vi "OP_Print_TPS_cluster_20171103.vi"() -> ()   [LabVIEW 2013]
uses:
  <vilib>/addons/database/Connection.llb/DB Tools Open Connec (Path).vi
  <vilib>/addons/database/Connection.llb/Conn Execute.vi
  <vilib>/addons/database/Recordset.llb/Rec Fetch Recordset Data (R).vi
  <vilib>/addons/database/Recordset.llb/Rec Destroy - Connection.vi
  <userlib>/caLab/Private/Get_PV-1D.vi
  <userlib>/caLab/Private/Get_PV.vi
  <vilib>/addons/database/_DB Variant To Data/Database Variant To Data.xnode
  <vilib>/addons/database/NI_Database_API.lvlib
panel:
  in  "Switch Tab":bool=TRUE
  out "Tab Control":enum32{"_____", "           "}(tab)
  out "Cluster":T1={"SR Fill Pattern"=array[864 elements], "Beam Current(mA"=320.769453, "Beam Lifetime(min)"=354.3939151043138, "Beamsize X(um)"=63.15189373514937, "Beamsize Y(um)"=38.03691397287648, "Tune X(from BPM)"=0.1487279843444227, "Tune Y(from BPM)"=0.2309197651663405, "Mode"="Top-Up", "NuX(from BBF) "=0.15142063757609414, "NuY(from BBF)"=0.22496346361412184, "IU22-23gap(R)"=7.0, "IU22-05gap(R)"=7.372, "IU22-05M"=TRUE, "IU22A-09gap(R)"=8.05, "IU22A-09M"=TRUE, "IU22B-09gap(R)"=40.001, "IU22B-09M"=FALSE, "IUT22-21gap(R)"=7.0, "IUT22-21M"=TRUE, "IU22-23M"=TRUE, "IU22A-25gap(R)"=7.0, "IU22A-25M"=TRUE, "IU22B-25gap(R)"=40.0, "IU22B-25M"=FALSE, "EPU48A-41gap(R)"=65.00055, "EPU48A-41gM"=FALSE, "EPU48B-41gap(R)"=27.450000000000003, "EPU48B-41gM"=TRUE, "EPU46-45gap(R)"=44.99850000000001, "EPU46-45gM"=FALSE, "EPU48A-41phase(R)"=0.00055, "EPU48B-41phase(R)"=0.0, "EPU46-45phase(R)"=5e-05, "Grid volt.(V)(S)"=33.0, "Gun mode"="MBM", "Mod.3 HV(kV)(S)"=35.37999999999996, "SR"="SR_DMB_2017_1024_0300LOCO.data", "BR"="Booster_2017_1023_0900.data", "Linac"="Linac_2017_0413_1015.data", "LTB"="LTB_JT_2017_0828_1050.data", "BTS"="BTS_2017_1023_0900.data", "RF2 remote"=TRUE, "RF2 OP mode"=TRUE, "RF2 phase.(S)"=-42.0, "RF Freq.(s)"=499655365.67399085, "RF2 gap volt.(S)"=1600.0, "RF3 remote"=TRUE, "RF3 OP mode"=TRUE, "RF3 phase.(S)"=1.1999999999999995, "RF3 gap volt.(S)"=1600.0, "BBF V"=TRUE, "BBF H"=TRUE, "BR ext. kicker1(kV)"=17.666, "BR ext. kicker2(kV)"=17.666, "BR ext. sep.1(V)"=322.14, "BR ext. sep.2(V)"=441.1, "BR inj. sep.(V)"=104.95, "BR inj. kicker(kV)"=13.449999999999969, "SR kicker4(kV)"=7.945, "SR kicker3(kV)"=8.02, "SR kicker2(kV)"=8.142, "SR kicker1(kV)"=8.1, "SR inj. sep.2(V)"=397.2, "SR inj. sep.1(V)"=398.04, "Bucket Start"=100.0, "Bucket Last"=450.0, "Bucket Step"=10.0, "Orbit ILK(P)"=TRUE, "IU22-05 Hutch Enable"=TRUE, "IU22A-09M Hutch Enable"=TRUE, "IUT22-21M Hutch Enable"=TRUE, "IU22-23M Hutch Enable"=TRUE, "IU22A-25M Hutch Enable"=TRUE, "EPU48A-41M Hutch Enable"=TRUE, "EPU46-45M Hutch Enable"=FALSE, "EPU46-45 FE Enable"=TRUE, "EPU48A-41 FE Enable"=TRUE, "IU22A-25 FE Enable"=TRUE, "IU22-23 FE Enable"=TRUE, "IUT22-21 FE Enable"=TRUE, "IU22A-09 FE Enable"=TRUE, "IU22-05 FE Enable"=TRUE, "EPU48A-41pM"=FALSE, "EPU48B-41pM"=TRUE, "EPU46-45pM"=FALSE, "Gun volt.(V)(S)"=23.5, "Width count"=75.0, "2ns step"=2.0, "10ps delay"=150.0, "phase shifter"=130.0015, "Taper"=1.0899999999999999, "05XBPMX 1"=14.279, "09XBPMX 1"=-34.837, "21XBPMX 1"=-36.466, "23XBPMX 1"=-38.547000000000004, "25XBPMX 1"=-40.08, "41XBPMX 1"=-513.551, "45XBPMX 1"=-12.86, "05XBPMY 1"=51.999, "09XBPMY 1"=30.004, "21XBPMY 1"=-4.771, "23XBPMY 1"=19.080000000000002, "25XBPMY 1"=-4.366, "41XBPMY 1"=309.241, "45XBPMY 1"=1.842, "FOFB H"="On", "FOFB V"="On", "time string"="15:45:09", "date"="2017/10/28", "date (last kicker ON)"="2017/10/28", "time string (last kicker ON)"="15:43:52", "Radio Buttons 2"=enum."absolute", "09XBPMX 2"="23.77", "09XBPMY 2"="-18.01", "05XBPMY 2"="-459.85", "05XBPMX 2"="-403.56", "21XBPMY 2"="-134.87", "21XBPMX 2"="-31.92", "23XBPMY 2"="233.82", "23XBPMX 2"="11.09", "25XBPMY 2"="5171.53", "25XBPMX 2"="2152.43", "41XBPMY 2"=" closed", "41XBPMX 2"=" PAB ", "45XBPMX 2"=" Hutch ", "45XBPMY 2"=" closed", "05 mode"="Follow", "09A mode"="Follow", "09B mode"="Follow", "21 mode"="Follow", "23 mode"="Follow", "25A mode"="Follow", "25B mode"="Follow", "41A mode"="Follow", "41B mode"="Follow", "46 mode"="Follow", "BeamCurrent History"={"BPM NO.  1_172"=array[4319 elements], array[4319 elements]}, "SR Beam Current in            hours"=12.0, "RF FB"="On", "BPMX Graph 2"={"Array of X axis  平均分配至各段"=[1.0, 1.1666666666666667, 1.3333333333333333, 1.5, 1.6666666666666665, 1.8333333333333333, 2.0, 2.142857142857143, 2.2857142857142856, 2.4285714285714284, 2.571428571428571, 2.7142857142857144, 2.857142857142857, 3.0, 3.142857142857143, 3.2857142857142856, 3.4285714285714284, 3.571428571428571, 3.7142857142857144, 3.857142857142857, 4.0, 4.125, 4.25, 4.375, 4.5, 4.625, 4.75, 4.875, 5.0, 5.125, 5.25, 5.375, 5.5, 5.625, 5.75, 5.875, 6.0, 6.142857142857143, 6.285714285714286, 6.428571428571429, 6.571428571428571, 6.714285714285714, 6.857142857142857, 7.0, 7.142857142857143, 7.285714285714286, 7.428571428571429, 7.571428571428571, 7.714285714285714, 7.857142857142857, 8.0, 8.142857142857142, 8.285714285714286, 8.428571428571429, 8.571428571428571, 8.714285714285714, 8.857142857142858, 9.0, 9.142857142857142, 9.285714285714286, 9.428571428571429, 9.571428571428571, 9.714285714285714, 9.857142857142858, 10.0, 10.142857142857142, 10.285714285714286, 10.428571428571429, 10.571428571428571, 10.714285714285714, 10.857142857142858, 11.0, 11.142857142857142, 11.285714285714286, 11.428571428571429, 11.571428571428571, 11.714285714285714, 11.857142857142858, 12.0, 12.125, 12.25, 12.375, 12.5, 12.625, 12.75, 12.875, 13.0, 13.125, 13.25, 13.375, 13.5, 13.625, 13.75, 13.875, 14.0, 14.142857142857142, 14.285714285714286, 14.428571428571429, 14.571428571428571, 14.714285714285714, 14.857142857142858, 15.0, 15.142857142857142, 15.285714285714286, 15.428571428571429, 15.571428571428571, 15.714285714285714, 15.857142857142858, 16.0, 16.142857142857142, 16.285714285714285, 16.428571428571427, 16.571428571428573, 16.714285714285715, 16.857142857142858, 17.0, 17.142857142857142, 17.285714285714285, 17.428571428571427, 17.571428571428573, 17.714285714285715, 17.857142857142858, 18.0, 18.142857142857142, 18.285714285714285, 18.428571428571427, 18.571428571428573, 18.714285714285715, 18.857142857142858, 19.0, 19.142857142857142, 19.285714285714285, 19.428571428571427, 19.571428571428573, 19.714285714285715, 19.857142857142858, 20.0, 20.125, 20.25, 20.375, 20.5, 20.625, 20.75, 20.875, 21.0, 21.125, 21.25, 21.375, 21.5, 21.625, 21.75, 21.875, 22.0, 22.142857142857142, 22.285714285714285, 22.428571428571427, 22.571428571428573, 22.714285714285715, 22.857142857142858, 23.0, 23.142857142857142, 23.285714285714285, 23.428571428571427, 23.571428571428573, 23.714285714285715, 23.857142857142858, 24.0, 24.166666666666668, 24.333333333333332, 24.5, 24.666666666666668, 24.833333333333332], [-104.35000000000001, -27.61, -81.269, 31.074, 6.062, -136.0, 99.494, -88.141, -46.889, -165.06900000000002, 6.021, -84.98, 1.75, -8.811, 8.532, -133.949, -96.848, 24.799, 5.059, -100.301, 144.643, -9.353, 21.271, -55.053000000000004, 53.308, 191.175, 158.868, 222.566, -123.501, -26.869, 534.8770000000001, 573.141, -225.076, -6.779, 120.711, -75.419, 85.256, 50.948, -59.4, -203.09900000000002, -20.847, 130.465, -112.508, 76.115, 15.039, -35.207, -105.659, -16.897000000000002, 68.91, -141.159, 107.378, 144.351, -55.053000000000004, -193.076, 129.21, 58.157000000000004, -162.566, 153.643, 28.149, 9.358, -84.211, 85.112, 22.422, -31.252, 89.379, -47.49, 54.793, -68.275, 110.611, -118.584, -371.90500000000003, -20.115000000000002, -329.103, -249.097, -146.817, 118.556, -25.749, -98.32600000000001, 55.269, -122.093, 50.967, -55.89, 88.019, -0.462, -608.1560000000001, -139.752, -304.999, -215.022, 93.23400000000001, 44.699, -65.235, 37.049, -3.491, -169.852, 216.458, 50.398, -92.285, -132.13400000000001, -12.869, 66.74, -188.53300000000002, 148.653, -5.112, -71.334, -177.681, 41.168, -12.532, -184.913, 194.919, 52.414, -75.628, -80.415, -36.814, 105.73100000000001, -104.36800000000001, 110.101, 49.669000000000004, -67.327, -157.372, 29.624000000000002, 22.156, -105.663, 47.799, 11.591000000000001, -75.285, -79.821, 34.331, -24.937, -158.703, 177.15, 200.872, -165.849, -60.67, 20.183, -15.311, -111.206, 107.58800000000001, 26.489, 69.547, -41.230000000000004, 81.986, 54.43, 253.076, 378.43600000000004, -117.003, -304.999, 131.013, 2.21, -158.435, 94.489, 63.017, -82.94500000000001, 99.147, 65.752, -37.261, -102.577, 41.791000000000004, 66.599, -163.73, 160.137, -7.15, -51.275, -140.353, 33.772, 54.203, -147.597, 128.696, 58.22, -47.144, -184.493, 56.980000000000004, 67.437, -54.227000000000004, -0.031]}, "BPMY Graph 2"={"Array of X axis  平均分配至各段"=[1.0, 1.1666666666666667, 1.3333333333333333, 1.5, 1.6666666666666665, 1.8333333333333333, 2.0, 2.142857142857143, 2.2857142857142856, 2.4285714285714284, 2.571428571428571, 2.7142857142857144, 2.857142857142857, 3.0, 3.142857142857143, 3.2857142857142856, 3.4285714285714284, 3.571428571428571, 3.7142857142857144, 3.857142857142857, 4.0, 4.125, 4.25, 4.375, 4.5, 4.625, 4.75, 4.875, 5.0, 5.125, 5.25, 5.375, 5.5, 5.625, 5.75, 5.875, 6.0, 6.142857142857143, 6.285714285714286, 6.428571428571429, 6.571428571428571, 6.714285714285714, 6.857142857142857, 7.0, 7.142857142857143, 7.285714285714286, 7.428571428571429, 7.571428571428571, 7.714285714285714, 7.857142857142857, 8.0, 8.142857142857142, 8.285714285714286, 8.428571428571429, 8.571428571428571, 8.714285714285714, 8.857142857142858, 9.0, 9.142857142857142, 9.285714285714286, 9.428571428571429, 9.571428571428571, 9.714285714285714, 9.857142857142858, 10.0, 10.142857142857142, 10.285714285714286, 10.428571428571429, 10.571428571428571, 10.714285714285714, 10.857142857142858, 11.0, 11.142857142857142, 11.285714285714286, 11.428571428571429, 11.571428571428571, 11.714285714285714, 11.857142857142858, 12.0, 12.125, 12.25, 12.375, 12.5, 12.625, 12.75, 12.875, 13.0, 13.125, 13.25, 13.375, 13.5, 13.625, 13.75, 13.875, 14.0, 14.142857142857142, 14.285714285714286, 14.428571428571429, 14.571428571428571, 14.714285714285714, 14.857142857142858, 15.0, 15.142857142857142, 15.285714285714286, 15.428571428571429, 15.571428571428571, 15.714285714285714, 15.857142857142858, 16.0, 16.142857142857142, 16.285714285714285, 16.428571428571427, 16.571428571428573, 16.714285714285715, 16.857142857142858, 17.0, 17.142857142857142, 17.285714285714285, 17.428571428571427, 17.571428571428573, 17.714285714285715, 17.857142857142858, 18.0, 18.142857142857142, 18.285714285714285, 18.428571428571427, 18.571428571428573, 18.714285714285715, 18.857142857142858, 19.0, 19.142857142857142, 19.285714285714285, 19.428571428571427, 19.571428571428573, 19.714285714285715, 19.857142857142858, 20.0, 20.125, 20.25, 20.375, 20.5, 20.625, 20.75, 20.875, 21.0, 21.125, 21.25, 21.375, 21.5, 21.625, 21.75, 21.875, 22.0, 22.142857142857142, 22.285714285714285, 22.428571428571427, 22.571428571428573, 22.714285714285715, 22.857142857142858, 23.0, 23.142857142857142, 23.285714285714285, 23.428571428571427, 23.571428571428573, 23.714285714285715, 23.857142857142858, 24.0, 24.166666666666668, 24.333333333333332, 24.5, 24.666666666666668, 24.833333333333332], [-143.858, -13.775, -13.785, 122.665, -66.475, 31.541, 2.118, -24.67, 28.275000000000002, 0.139, -36.578, -28.396, 48.925000000000004, 9.287, -3.412, 70.053, -21.479, 14.89, -7.234, 5.521, -3.164, 19.558, -37.538000000000004, 37.11, -77.159, -13.755, 77.63, 28.249000000000002, -209.114, -44.569, 92.851, 173.641, -70.156, -22.722, 17.795, -6.59, 25.654, -41.882, 53.713, 9.237, -26.164, 18.357, 63.695, -8.542, 5.183, -5.99, 9.508000000000001, -5.462, -29.446, 36.574, -52.552, 51.439, -48.502, 0.73, -23.836000000000002, -3.648, -9.628, -5.485, -68.679, 95.486, -62.041000000000004, 54.633, -58.791000000000004, 68.305, -49.682, 29.838, -8.459, 3.213, -5.561, -80.617, 58.144, 15.346, -158.743, -40.726, 5.259, 3.258, 41.128, -54.377, 5.01, 18.84, 11.403, -20.73, 21.792, -17.296, 27.29, 0.783, -6.804, -137.476, 116.70700000000001, -6.929, 17.846, -3.586, 11.754, 6.341, 0.292, -0.911, -8.236, -5.312, 14.939, -29.945, 30.573, -9.991, -49.344, 82.117, -27.45, 22.291, -6.636, -9.389, 10.034, -14.218, 14.215, -7.3, 12.409, -44.302, 50.197, -36.089, -9.120000000000001, 45.881, 14.836, -27.324, 10.765, -10.139, -33.252, 2.737, -9.99, -6.019, -53.329, -28.159, 2.676, -36.9, -2.372, 8.92, 13.599, -25.723, -16.436, 7.722, -0.088, -29.122, 32.814, -20.521, 30.155, -45.734, 36.611000000000004, 74.528, 68.482, -22.548000000000002, -31.398, 134.603, -45.587, -0.981, -40.156, 24.441, 20.477, -31.424, 19.5, -11.789, 16.394000000000002, -38.567, 9.523, 0.09, -0.058, -4.8500000000000005, 11.71, 25.637, -10.51, -18.101, -12.389000000000001, 95.417, -138.726, 30.355, 96.245, -48.666000000000004, 40.851, -0.71]}, "gap value："=0} {"SR Beam Current in            hours" min=1.0 max=24.0 step=1.0 format="%#_2f"; "45XBPMY 1" format="%#.2f"; "41XBPMY 1" format="%#.2f"; "25XBPMY 1" format="%#.2f"; "23XBPMY 1" format="%#.2f"; "21XBPMY 1" format="%#.2f"; "09XBPMY 1" format="%#.2f"; "05XBPMY 1" format="%#.2f"; "45XBPMX 1" format="%#.2f"; "41XBPMX 1" format="%#.2f"; "25XBPMX 1" format="%#.2f"; "23XBPMX 1" format="%#.2f"; "21XBPMX 1" format="%#.2f"; "09XBPMX 1" format="%#.2f"; "05XBPMX 1" format="%#.2f"; "Taper" format="%#.4f"; "phase shifter" format="%#.3f"; "10ps delay" format="%#.1f"; "2ns step" format="%#.1f"; "Width count" format="%#.1f"; "Gun volt.(V)(S)" format="%#.1f"; "Bucket Step" format="%#.2f"; "Bucket Last" format="%#.2f"; "Bucket Start" format="%#.2f"; "BR ext. kicker1(kV)" format="%#.2f"; "BR ext. kicker2(kV)" format="%#.2f"; "BR ext. sep.1(V)" format="%#.2f"; "BR ext. sep.2(V)" format="%#.2f"; "BR inj. sep.(V)" format="%#.3f"; "BR inj. kicker(kV)" format="%#.3f"; "SR kicker4(kV)" format="%#.2f"; "SR kicker3(kV)" format="%#.2f"; "SR kicker2(kV)" format="%#.2f"; "SR kicker1(kV)" format="%#.2f"; "SR inj. sep.2(V)" format="%#.2f"; "SR inj. sep.1(V)" format="%#.2f"; "RF3 gap volt.(S)" format="%#.0f"; "RF3 phase.(S)" format="%#.1f"; "RF2 gap volt.(S)" format="%#.0f"; "RF Freq.(s)" format="%#.1f"; "RF2 phase.(S)" format="%#.1f"; "Mod.3 HV(kV)(S)" format="%#.3f"; "Grid volt.(V)(S)" format="%#.1f"; "EPU46-45phase(R)" format="%#.4f"; "EPU48B-41phase(R)" format="%#.4f"; "EPU48A-41phase(R)" format="%#.4f"; "EPU46-45gap(R)" format="%#.4f"; "EPU48B-41gap(R)" format="%#.4f"; "EPU48A-41gap(R)" format="%#.4f"; "IU22B-25gap(R)" format="%#.4f"; "IU22A-25gap(R)" format="%#.4f"; "IUT22-21gap(R)" format="%#.4f"; "IU22B-09gap(R)" format="%#.4f"; "IU22A-09gap(R)" format="%#.4f"; "IU22-05gap(R)" format="%#.4f"; "IU22-23gap(R)" format="%#.4f"; "NuY(from BBF)" format="%#.4f"; "NuX(from BBF)" format="%#.4f"; "Tune Y(from BPM)" format="%#.4f"; "Tune X(from BPM)" format="%#.4f"; "Beamsize Y(um)" format="%#.2f"; "Beamsize X(um)" format="%#.2f"; "Beam Lifetime(min)" format="%#.3f"; "Beam Current(mA" format="%#.3f"}
  out "Diff list":string[][](array[string])
  out "EVENTs":i32
  out "check loop":i32
  in  "Check period":i32=10 min=0 max=10
  out "Program Start Time":dbl=3592021508.642459
  out "dT":u32=325
  out "x > y?":bool
  out "PV list":string[](array[string])=["LI-ES-CPS-01:SETMODE", "LI-ES-CPS-01:PULSEMODE", "LI-ES-BPS-01:SETU:GRID", "LI-ES-BPS-01:SETU:SBM", "LI-ES-BPS-01:SETU:MBM", "LI-RF-CAB-07:SET:MODE", "LI-RF-HVP-11:SET:U", "LI-RF-CAB-09:SET:MODE", "LI-RF-HVP-21:SET:U", "LI-RF-CAB-11:SET:MODE", "LI-RF-HVP-31:SET:U", "LI-RF-WGA-01:SET:POS", "LI-RF-WGA-02:SET:POS", "LI-RF-WGA-03:SET:POS", "LI-RF-SFT-01:SET:POS", "LI-RF-SFT-02:SET:POS", "LI-RF-SFT-03:SET:POS", "LI-RF-CTR-01:ES:SET:DEG", "LI-RF-CTR-01:SP:SET:DEG", "LI-RF-CTR-01:K123:SET:DEG", "LI-RF-CTR-01:K1:SET:DEG", "LI-RF-CTR-01:K3:SET:DEG", "LI-RF-AMP-01:SET:PWR", "LI-RF-AMP-02:SET:PWR", "LI-MA-SPS-01:SET:I", "LI-MA-SPS-02:SET:I", "LI-MA-SPS-03:SET:I", "LI-MA-SPS-04:SET:I", "LI-MA-SPS-05:SET:I", "LI-MA-SPS-06:SET:I", "LI-MA-SPS-07:SET:I", "LI-MA-SPS-08:SET:I", "LI-MA-SPS-09:SET:I", "LI-MA-SPS-10:SET:I", "LI-MA-SPS-11:SET:I", "LI-MA-SPS-12:SET:I", "LI-MA-SPS-13:SET:I", "LI-MA-SPS-14:SET:I", "LI-MA-SPS-15:SET:I", "LI-MA-SPS-16:SET:I", "LI-MA-STP-01:SET:I", "LI-MA-STP-02:SET:I", "LI-MA-STP-03:SET:I", "LI-MA-STP-04:SET:I", "LI-MA-STP-05:SET:I", "LI-MA-STP-06:SET:I", "LI-MA-STP-07:SET:I", "LI-MA-STP-08:SET:I", "LI-MA-STP-09:SET:I", "LI-MA-STP-10:SET:I", "LI-MA-STP-11:SET:I", "LI-MA-STP-12:SET:I", "LI-MA-STP-13:SET:I", "LI-MA-STP-14:SET:I", "LI-MA-STP-15:SET:I", "LI-MA-STP-16:SET:I", "LI-MA-QPS-01:SET:I", "LI-MA-QPS-02:SET:I", "LI-MA-QPS-03:SET:I", "LI-MA-QPS-04:SET:I", "LI-MA-QPS-05:SET:I", "LI-MA-QPS-06:SET:I", "CPCITM-TI-EVRTG:Pulse7DelaySet", "CPCITM-TI-EVRTG:Pulse7WidthSet", "CPCITM-TI-EVRTG:GTX7CtrlGTXPHSet", "CPCITM-TI-EVRTG:GTX7DlySet", "CPCITM-TI-EVRTG:Pulse6DelaySet", "CPCITM-TI-EVRTG:Pulse6WidthSet", "CPCITM-TI-EVRTG:GTX6CtrlGTXPHSet", "CPCITM-TI-EVRTG:GTX6DlySet", "CPCILI-TI-EVR:Pulse2DelaySet", "CPCILI-TI-EVR:Pulse2WidthSet", "CPCILI-TI-EVR:Pulse3DelaySet", "CPCILI-TI-EVR:Pulse3WidthSet", "CPCILI-TI-EVR:Pulse4DelaySet", "CPCILI-TI-EVR:Pulse4WidthSet", "CPCILI-TI-EVR:Pulse5DelaySet", "CPCILI-TI-EVR:Pulse5WidthSet", "CPCILI-TI-EVR:Pulse6DelaySet", "CPCILI-TI-EVR:Pulse6WidthSet", "CPCILI-TI-EVR:Pulse7DelaySet", "CPCILI-TI-EVR:Pulse7WidthSet", "CPCILI-TI-EVR:Pulse8DelaySet", "CPCILI-TI-EVR:Pulse8WidthSet", "CPCILI-TI-EVR:Pulse9DelaySet", "CPCILI-TI-EVR:Pulse9WidthSet", "CPCITM-TI-EVRTG:GTX6DlySet", "CPCITM-TI-EVRTG:GTX7DlySet", "LTB-PS-HC-1:setI", "LTB-PS-HC-2:setI", "LTB-PS-HC-3:setI", "LTB-PS-HC-4:setI", "LTB-PS-HC-5:setI", "LTB-PS-VC-1:setI", "LTB-PS-VC-2:setI", "LTB-PS-VC-3:setI", "LTB-PS-VC-4:setI", "LTB-PS-VC-5:setI", "LTB-PS-VC-6:setI", "LTB-PS-VC-7:setI", "LTB-PS-Q1A:setI", "LTB-PS-Q1B:setI", "LTB-PS-Q1C:setI", "LTB-PS-Q2A:setI", "LTB-PS-Q2B:setI", "LTB-PS-Q2C:setI", "LTB-PS-Q3A:setI", "LTB-PS-Q3B:setI", "LTB-PS-Q4A:setI", "LTB-PS-Q4B:setI", "LTB-PS-QQ:setI", "LTB-PS-BEND-1:setI", "LTB-PS-VC-2a:setI", "LTB-PS-HC-3a:setI", "LTB-PS-HC-3b:setI", "LTB-PS-HC-4a:setI", "LTB-PS-HC-5a:setI", "LI-DI-SLIT-motor:axis2Position1", "LI-DI-SLIT-motor:axis1Position1", "BR-PS-HC-101:setI", "BR-PS-HC-102:setI", "BR-PS-HC-103:setI", "BR-PS-HC-104:setI", "BR-PS-HC-105:setI", "BR-PS-HC-106:setI", "BR-PS-HC-107:setI", "BR-PS-HC-108:setI", "BR-PS-HC-109:setI", "BR-PS-HC-110:setI", "BR-PS-HC-201:setI", "BR-PS-HC-202:setI", "BR-PS-HC-203:setI", "BR-PS-HC-204:setI", "BR-PS-HC-205:setI", "BR-PS-HC-206:setI", "BR-PS-HC-207:setI", "BR-PS-HC-208:setI", "BR-PS-HC-209:setI", "BR-PS-HC-210:setI", "BR-PS-HC-301:setI", "BR-PS-HC-302:setI", "BR-PS-HC-303:setI", "BR-PS-HC-304:setI", "BR-PS-HC-305:setI", "BR-PS-HC-306:setI", "BR-PS-HC-307:setI", "BR-PS-HC-308:setI", "BR-PS-HC-309:setI", "BR-PS-HC-310:setI", "BR-PS-HC-401:setI", "BR-PS-HC-402:setI", "BR-PS-HC-403:setI", "BR-PS-HC-404:setI", "BR-PS-HC-405:setI", "BR-PS-HC-406:setI", "BR-PS-HC-407:setI", "BR-PS-HC-408:setI", "BR-PS-HC-409:setI", "BR-PS-HC-410:setI", "BR-PS-HC-501:setI", "BR-PS-HC-502:setI", "BR-PS-HC-503:setI", "BR-PS-HC-504:setI", "BR-PS-HC-505:setI", "BR-PS-HC-506:setI", "BR-PS-HC-507:setI", "BR-PS-HC-508:setI", "BR-PS-HC-509:setI", "BR-PS-HC-510:setI", "BR-PS-HC-601:setI", "BR-PS-HC-602:setI", "BR-PS-HC-603:setI", "BR-PS-HC-603a:setI", "BR-PS-HC-604:setI", "BR-PS-HC-605:setI", "BR-PS-HC-606:setI", "BR-PS-HC-606a:setI", "BR-PS-HC-607:setI", "BR-PS-HC-608:setI", "BR-PS-HC-609:setI", "BR-PS-HC-610:setI", "BR-PS-VC-101:setI", "BR-PS-VC-102:setI", "BR-PS-VC-103:setI", "BR-PS-VC-104:setI", "BR-PS-VC-105:setI", "BR-PS-VC-106:setI", "BR-PS-VC-201:setI", "BR-PS-VC-202:setI", "BR-PS-VC-203:setI", "BR-PS-VC-204:setI", "BR-PS-VC-205:setI", "BR-PS-VC-206:setI", "BR-PS-VC-301:setI", "BR-PS-VC-302:setI", "BR-PS-VC-303:setI", "BR-PS-VC-304:setI", "BR-PS-VC-305:setI", "BR-PS-VC-306:setI", "BR-PS-VC-401:setI", "BR-PS-VC-402:setI", "BR-PS-VC-403:setI", "BR-PS-VC-404:setI", "BR-PS-VC-405:setI", "BR-PS-VC-406:setI", "BR-PS-VC-501:setI", "BR-PS-VC-502:setI", "BR-PS-VC-503:setI", "BR-PS-VC-504:setI", "BR-PS-VC-505:setI", "BR-PS-VC-506:setI", "BR-PS-VC-601:setI", "BR-PS-VC-602:setI", "BR-PS-VC-602a:setI", "BR-PS-VC-603:setI", "BR-PS-VC-604:setI", "BR-PS-VC-604a:setI", "BR-PS-VC-605:setI", "BR-PS-VC-606:setI", "BR-PS-VC-100a:setI", "BR-PS-SD:setI", "BR-PS-SF:setI", "cpsc_027:AO:SLOW_SET:CH:1", "cpsc_037:AO:SLOW_SET:CH:3", "BR-RF-LLRF:setStationPhase", "TI-INJ-PROC:setTinj", "BR-PS-INJ-SE:setHV", "CPCIPM-TI-EVR:Pulse1DelaySet", "BR-PS-INJ-KI:setHV", "CPCIPM-TI-EVR:Pulse2DelaySet", "BR-PS-QF:setWfDC", "BR-PS-QM:setWfDC", "BR-PS-Q1:setWfDC", "BR-PS-Q2:setWfDC", "BR-PS-BEND:setWfDC", "BTS-PS-HC-1:setI", "BTS-PS-HC-2:setI", "BTS-PS-HC-3:setI", "BTS-PS-HC-4:setI", "BTS-PS-HC-5:setI", "BTS-PS-VC-2:setI", "BTS-PS-VC-3:setI", "BTS-PS-VC-4:setI", "BTS-PS-VC-5:setI", "BTS-PS-VC-6:setI", "BTS-PS-Q1A:setI", "BTS-PS-Q1B:setI", "BTS-PS-Q1C:setI", "BTS-PS-Q2A:setI", "BTS-PS-Q2B:setI", "BTS-PS-Q2C:setI", "BTS-PS-Q3A:setI", "BTS-PS-BEND-1:setI", "BTS-PS-BEND-2:setI", "BR-PS-EXT-K1:setHV", "BR-PS-EXT-K2:setHV", "SR-PS-INJ-SE1:setHV", "SR-PS-INJ-SE2:setHV", "SR-PS-INJ-K1:setHV", "SR-PS-INJ-K2:setHV", "SR-PS-INJ-K3:setHV", "SR-PS-INJ-K4:setHV", "CPCIPM-TI-EVR:Pulse4DelaySet", "CPCIPM-TI-EVR:Pulse5DelaySet", "CPCIPM-TI-EVR:Pulse3DelaySet", "CPCIPM-TI-EVR:Pulse6DelaySet", "CPCIPM-TI-EVR:Pulse7DelaySet", "T560:setADelay", "T560:setBDelay", "T560:setCDelay", "T560:setDDelay", "CPCIPM-TI-EVR:Pulse4DelaySet", "CPCIPM-TI-EVR:Pulse5DelaySet", "BR-PS-EXT-SE1:setHV", "BR-PS-EXT-SE2:setHV", "CPCIPM-TI-EVR:Pulse3DelaySet", "CPCIPM-TI-EVR:Pulse11DelaySet", "SR-PS-BEND:setI", "SR-PS-HC-011:setI", "SR-PS-HC-012:setI", "SR-PS-HC-013:setI", "SR-PS-HC-014:setI", "SR-PS-HC-015:setI", "SR-PS-HC-016:setI", "SR-PS-HC-017:setI", "SR-PS-HC-021:setI", "SR-PS-HC-022:setI", "SR-PS-HC-023:setI", "SR-PS-HC-024:setI", "SR-PS-HC-025:setI", "SR-PS-HC-026:setI", "SR-PS-HC-027:setI", "SR-PS-HC-031:setI", "SR-PS-HC-032:setI", "SR-PS-HC-033:setI", "SR-PS-HC-034:setI", "SR-PS-HC-035:setI", "SR-PS-HC-036:setI", "SR-PS-HC-037:setI", "SR-PS-HC-041:setI", "SR-PS-HC-042:setI", "SR-PS-HC-043:setI", "SR-PS-HC-044:setI", "SR-PS-HC-045:setI", "SR-PS-HC-046:setI", "SR-PS-HC-047:setI", "SR-PS-HC-051:setI", "SR-PS-HC-052:setI", "SR-PS-HC-053:setI", "SR-PS-HC-054:setI", "SR-PS-HC-055:setI", "SR-PS-HC-056:setI", "SR-PS-HC-057:setI", "SR-PS-HC-061:setI", "SR-PS-HC-062:setI", "SR-PS-HC-063:setI", "SR-PS-HC-064:setI", "SR-PS-HC-065:setI", "SR-PS-HC-066:setI", "SR-PS-HC-067:setI", "SR-PS-HC-071:setI", "SR-PS-HC-072:setI", "SR-PS-HC-073:setI", "SR-PS-HC-074:setI", "SR-PS-HC-075:setI", "SR-PS-HC-076:setI", "SR-PS-HC-077:setI", "SR-PS-HC-081:setI", "SR-PS-HC-082:setI", "SR-PS-HC-083:setI", "SR-PS-HC-084:setI", "SR-PS-HC-085:setI", "SR-PS-HC-086:setI", "SR-PS-HC-087:setI", "SR-PS-HC-091:setI", "SR-PS-HC-092:setI", "SR-PS-HC-093:setI", "SR-PS-HC-094:setI", "SR-PS-HC-095:setI", "SR-PS-HC-096:setI", "SR-PS-HC-097:setI", "SR-PS-HC-101:setI", "SR-PS-HC-102:setI", "SR-PS-HC-103:setI", "SR-PS-HC-104:setI", "SR-PS-HC-105:setI", "SR-PS-HC-106:setI", "SR-PS-HC-107:setI", "SR-PS-HC-111:setI", "SR-PS-HC-112:setI", "SR-PS-HC-113:setI", "SR-PS-HC-114:setI", "SR-PS-HC-115:setI", "SR-PS-HC-116:setI", "SR-PS-HC-117:setI", "SR-PS-HC-121:setI", "SR-PS-HC-122:setI", "SR-PS-HC-123:setI", "SR-PS-HC-124:setI", "SR-PS-HC-125:setI", "SR-PS-HC-126:setI", "SR-PS-HC-127:setI", "SR-PS-HC-131:setI", "SR-PS-HC-132:setI", "SR-PS-HC-133:setI", "SR-PS-HC-134:setI", "SR-PS-HC-135:setI", "SR-PS-HC-136:setI", "SR-PS-HC-137:setI", "SR-PS-HC-141:setI", "SR-PS-HC-142:setI", "SR-PS-HC-143:setI", "SR-PS-HC-144:setI", "SR-PS-HC-145:setI", "SR-PS-HC-146:setI", "SR-PS-HC-147:setI", "SR-PS-HC-151:setI", "SR-PS-HC-152:setI", "SR-PS-HC-153:setI", "SR-PS-HC-154:setI", "SR-PS-HC-155:setI", "SR-PS-HC-156:setI", "SR-PS-HC-157:setI", "SR-PS-HC-161:setI", "SR-PS-HC-162:setI", "SR-PS-HC-163:setI", "SR-PS-HC-164:setI", "SR-PS-HC-165:setI", "SR-PS-HC-166:setI", "SR-PS-HC-167:setI", "SR-PS-HC-171:setI", "SR-PS-HC-172:setI", "SR-PS-HC-173:setI", "SR-PS-HC-174:setI", "SR-PS-HC-175:setI", "SR-PS-HC-176:setI", "SR-PS-HC-177:setI", "SR-PS-HC-181:setI", "SR-PS-HC-182:setI", "SR-PS-HC-183:setI", "SR-PS-HC-184:setI", "SR-PS-HC-185:setI", "SR-PS-HC-186:setI", "SR-PS-HC-187:setI", "SR-PS-HC-191:setI", "SR-PS-HC-192:setI", "SR-PS-HC-193:setI", "SR-PS-HC-194:setI", "SR-PS-HC-195:setI", "SR-PS-HC-196:setI", "SR-PS-HC-197:setI", "SR-PS-HC-201:setI", "SR-PS-HC-202:setI", "SR-PS-HC-203:setI", "SR-PS-HC-204:setI", "SR-PS-HC-205:setI", "SR-PS-HC-206:setI", "SR-PS-HC-207:setI", "SR-PS-HC-211:setI", "SR-PS-HC-212:setI", "SR-PS-HC-213:setI", "SR-PS-HC-214:setI", "SR-PS-HC-215:setI", "SR-PS-HC-216:setI", "SR-PS-HC-217:setI", "SR-PS-HC-221:setI", "SR-PS-HC-222:setI", "SR-PS-HC-223:setI", "SR-PS-HC-224:setI", "SR-PS-HC-225:setI", "SR-PS-HC-226:setI", "SR-PS-HC-227:setI", "SR-PS-HC-231:setI", "SR-PS-HC-232:setI", "SR-PS-HC-233:setI", "SR-PS-HC-234:setI", "SR-PS-HC-235:setI", "SR-PS-HC-236:setI", "SR-PS-HC-237:setI", "SR-PS-HC-241:setI", "SR-PS-HC-242:setI", "SR-PS-HC-243:setI", "SR-PS-HC-244:setI", "SR-PS-HC-245:setI", "SR-PS-HC-246:setI", "SR-PS-HC-247:setI", "SR-PS-VC-011:setI", "SR-PS-VC-012:setI", "SR-PS-VC-013:setI", "SR-PS-VC-014:setI", "SR-PS-VC-015:setI", "SR-PS-VC-016:setI", "SR-PS-VC-017:setI", "SR-PS-VC-021:setI", "SR-PS-VC-022:setI", "SR-PS-VC-023:setI", "SR-PS-VC-024:setI", "SR-PS-VC-025:setI", "SR-PS-VC-026:setI", "SR-PS-VC-027:setI", "SR-PS-VC-031:setI", "SR-PS-VC-032:setI", "SR-PS-VC-033:setI", "SR-PS-VC-034:setI", "SR-PS-VC-035:setI", "SR-PS-VC-036:setI", "SR-PS-VC-037:setI", "SR-PS-VC-041:setI", "SR-PS-VC-042:setI", "SR-PS-VC-043:setI", "SR-PS-VC-044:setI", "SR-PS-VC-045:setI", "SR-PS-VC-046:setI", "SR-PS-VC-047:setI", "SR-PS-VC-051:setI", "SR-PS-VC-052:setI", "SR-PS-VC-053:setI", "SR-PS-VC-054:setI", "SR-PS-VC-055:setI", "SR-PS-VC-056:setI", "SR-PS-VC-057:setI", "SR-PS-VC-061:setI", "SR-PS-VC-062:setI", "SR-PS-VC-063:setI", "SR-PS-VC-064:setI", "SR-PS-VC-065:setI", "SR-PS-VC-066:setI", "SR-PS-VC-067:setI", "SR-PS-VC-071:setI", "SR-PS-VC-072:setI", "SR-PS-VC-073:setI", "SR-PS-VC-074:setI", "SR-PS-VC-075:setI", "SR-PS-VC-076:setI", "SR-PS-VC-077:setI", "SR-PS-VC-081:setI", "SR-PS-VC-082:setI", "SR-PS-VC-083:setI", "SR-PS-VC-084:setI", "SR-PS-VC-085:setI", "SR-PS-VC-086:setI", "SR-PS-VC-087:setI", "SR-PS-VC-091:setI", "SR-PS-VC-092:setI", "SR-PS-VC-093:setI", "SR-PS-VC-094:setI", "SR-PS-VC-095:setI", "SR-PS-VC-096:setI", "SR-PS-VC-097:setI", "SR-PS-VC-101:setI", "SR-PS-VC-102:setI", "SR-PS-VC-103:setI", "SR-PS-VC-104:setI", "SR-PS-VC-105:setI", "SR-PS-VC-106:setI", "SR-PS-VC-107:setI", "SR-PS-VC-111:setI", "SR-PS-VC-112:setI", "SR-PS-VC-113:setI", "SR-PS-VC-114:setI", "SR-PS-VC-115:setI", "SR-PS-VC-116:setI", "SR-PS-VC-117:setI", "SR-PS-VC-121:setI", "SR-PS-VC-122:setI", "SR-PS-VC-123:setI", "SR-PS-VC-124:setI", "SR-PS-VC-125:setI", "SR-PS-VC-126:setI", "SR-PS-VC-127:setI", "SR-PS-VC-131:setI", "SR-PS-VC-132:setI", "SR-PS-VC-133:setI", "SR-PS-VC-134:setI", "SR-PS-VC-135:setI", "SR-PS-VC-136:setI", "SR-PS-VC-137:setI", "SR-PS-VC-141:setI", "SR-PS-VC-142:setI", "SR-PS-VC-143:setI", "SR-PS-VC-144:setI", "SR-PS-VC-145:setI", "SR-PS-VC-146:setI", "SR-PS-VC-147:setI", "SR-PS-VC-151:setI", "SR-PS-VC-152:setI", "SR-PS-VC-153:setI", "SR-PS-VC-154:setI", "SR-PS-VC-155:setI", "SR-PS-VC-156:setI", "SR-PS-VC-157:setI", "SR-PS-VC-161:setI", "SR-PS-VC-162:setI", "SR-PS-VC-163:setI", "SR-PS-VC-164:setI", "SR-PS-VC-165:setI", "SR-PS-VC-166:setI", "SR-PS-VC-167:setI", "SR-PS-VC-171:setI", "SR-PS-VC-172:setI", "SR-PS-VC-173:setI", "SR-PS-VC-174:setI", "SR-PS-VC-175:setI", "SR-PS-VC-176:setI", "SR-PS-VC-177:setI", "SR-PS-VC-181:setI", "SR-PS-VC-182:setI", "SR-PS-VC-183:setI", "SR-PS-VC-184:setI", "SR-PS-VC-185:setI", "SR-PS-VC-186:setI", "SR-PS-VC-187:setI", "SR-PS-VC-191:setI", "SR-PS-VC-192:setI", "SR-PS-VC-193:setI", "SR-PS-VC-194:setI", "SR-PS-VC-195:setI", "SR-PS-VC-196:setI", "SR-PS-VC-197:setI", "SR-PS-VC-201:setI", "SR-PS-VC-202:setI", "SR-PS-VC-203:setI", "SR-PS-VC-204:setI", "SR-PS-VC-205:setI", "SR-PS-VC-206:setI", "SR-PS-VC-207:setI", "SR-PS-VC-211:setI", "SR-PS-VC-212:setI", "SR-PS-VC-213:setI", "SR-PS-VC-214:setI", "SR-PS-VC-215:setI", "SR-PS-VC-216:setI", "SR-PS-VC-217:setI", "SR-PS-VC-221:setI", "SR-PS-VC-222:setI", "SR-PS-VC-223:setI", "SR-PS-VC-224:setI", "SR-PS-VC-225:setI", "SR-PS-VC-226:setI", "SR-PS-VC-227:setI", "SR-PS-VC-231:setI", "SR-PS-VC-232:setI", "SR-PS-VC-233:setI", "SR-PS-VC-234:setI", "SR-PS-VC-235:setI", "SR-PS-VC-236:setI", "SR-PS-VC-237:setI", "SR-PS-VC-241:setI", "SR-PS-VC-242:setI", "SR-PS-VC-243:setI", "SR-PS-VC-244:setI", "SR-PS-VC-245:setI", "SR-PS-VC-246:setI", "SR-PS-VC-247:setI", "SR-PS-QL1-0101:setI", "SR-PS-QL2-0102:setI", "SR-PS-QL3-0103:setI", "SR-PS-QS4-0104:setI", "SR-PS-QS5-0105:setI", "SR-PS-QS5-0106:setI", "SR-PS-QS4-0107:setI", "SR-PS-QS3-0108:setI", "SR-PS-QS2-0109:setI", "SR-PS-QS1-0110:setI", "SR-PS-QS1-0201:setI", "SR-PS-QS2-0202:setI", "SR-PS-QS3-0203:setI", "SR-PS-QS4-0204:setI", "SR-PS-QS5-0205:setI", "SR-PS-QS5-0206:setI", "SR-PS-QS4-0207:setI", "SR-PS-QS3-0208:setI", "SR-PS-QS2-0209:setI", "SR-PS-QS1-0210:setI", "SR-PS-QS1-0301:setI", "SR-PS-QS2-0302:setI", "SR-PS-QS3-0303:setI", "SR-PS-QS4-0304:setI", "SR-PS-QS5-0305:setI", "SR-PS-QS5-0306:setI", "SR-PS-QS4-0307:setI", "SR-PS-QS3-0308:setI", "SR-PS-QS2-0309:setI", "SR-PS-QS1-0310:setI", "SR-PS-QS1-0401:setI", "SR-PS-QS2-0402:setI", "SR-PS-QS3-0403:setI", "SR-PS-QS4-0404:setI", "SR-PS-QS5-0405:setI", "SR-PS-QS5-0406:setI", "SR-PS-QS4-0407:setI", "SR-PS-QL3-0408:setI", "SR-PS-QL2-0409:setI", "SR-PS-QL1-0410:setI", "SR-PS-QL1-0501:setI", "SR-PS-QL2-0502:setI", "SR-PS-QL3-0503:setI", "SR-PS-QS4-0504:setI", "SR-PS-QS5-0505:setI", "SR-PS-QS5-0506:setI", "SR-PS-QS4-0507:setI", "SR-PS-QS3-0508:setI", "SR-PS-QS2-0509:setI", "SR-PS-QS1-0510:setI", "SR-PS-QS1-0601:setI", "SR-PS-QS2-0602:setI", "SR-PS-QS3-0603:setI", "SR-PS-QS4-0604:setI", "SR-PS-QS5-0605:setI", "SR-PS-QS5-0606:setI", "SR-PS-QS4-0607:setI", "SR-PS-QS3-0608:setI", "SR-PS-QS2-0609:setI", "SR-PS-QS1-0610:setI", "SR-PS-QS1-0701:setI", "SR-PS-QS2-0702:setI", "SR-PS-QS3-0703:setI", "SR-PS-QS4-0704:setI", "SR-PS-QS5-0705:setI", "SR-PS-QS5-0706:setI", "SR-PS-QS4-0707:setI", "SR-PS-QS3-0708:setI", "SR-PS-QS2-0709:setI", "SR-PS-QS1-0710:setI", "SR-PS-QS1-0801:setI", "SR-PS-QS2-0802:setI", "SR-PS-QS3-0803:setI", "SR-PS-QS4-0804:setI", "SR-PS-QS5-0805:setI", "SR-PS-QS5-0806:setI", "SR-PS-QS4-0807:setI", "SR-PS-QL3-0808:setI", "SR-PS-QL2-0809:setI", "SR-PS-QL1-0810:setI", "SR-PS-QL1-0901:setI", "SR-PS-QL2-0902:setI", "SR-PS-QL3-0903:setI", "SR-PS-QS4-0904:setI", "SR-PS-QS5-0905:setI", "SR-PS-QS5-0906:setI", "SR-PS-QS4-0907:setI", "SR-PS-QS3-0908:setI", "SR-PS-QS2-0909:setI", "SR-PS-QS1-0910:setI", "SR-PS-QS1-1001:setI", "SR-PS-QS2-1002:setI", "SR-PS-QS3-1003:setI", "SR-PS-QS4-1004:setI", "SR-PS-QS5-1005:setI", "SR-PS-QS5-1006:setI", "SR-PS-QS4-1007:setI", "SR-PS-QS3-1008:setI", "SR-PS-QS2-1009:setI", "SR-PS-QS1-1010:setI", "SR-PS-QS1-1101:setI", "SR-PS-QS2-1102:setI", "SR-PS-QS3-1103:setI", "SR-PS-QS4-1104:setI", "SR-PS-QS5-1105:setI", "SR-PS-QS5-1106:setI", "SR-PS-QS4-1107:setI", "SR-PS-QS3-1108:setI", "SR-PS-QS2-1109:setI", "SR-PS-QS1-1110:setI", "SR-PS-QS1-1201:setI", "SR-PS-QS2-1202:setI", "SR-PS-QS3-1203:setI", "SR-PS-QS4-1204:setI", "SR-PS-QS5-1205:setI", "SR-PS-QS5-1206:setI", "SR-PS-QS4-1207:setI", "SR-PS-QL3-1208:setI", "SR-PS-QL2-1209:setI", "SR-PS-QL1-1210:setI", "SR-PS-QL1-1301:setI", "SR-PS-QL2-1302:setI", "SR-PS-QL3-1303:setI", "SR-PS-QS4-1304:setI", "SR-PS-QS5-1305:setI", "SR-PS-QS5-1306:setI", "SR-PS-QS4-1307:setI", "SR-PS-QS3-1308:setI", "SR-PS-QS2-1309:setI", "SR-PS-QS1-1310:setI", "SR-PS-QS1-1401:setI", "SR-PS-QS2-1402:setI", "SR-PS-QS3-1403:setI", "SR-PS-QS4-1404:setI", "SR-PS-QS5-1405:setI", "SR-PS-QS5-1406:setI", "SR-PS-QS4-1407:setI", "SR-PS-QS3-1408:setI", "SR-PS-QS2-1409:setI", "SR-PS-QS1-1410:setI", "SR-PS-QS1-1501:setI", "SR-PS-QS2-1502:setI", "SR-PS-QS3-1503:setI", "SR-PS-QS4-1504:setI", "SR-PS-QS5-1505:setI", "SR-PS-QS5-1506:setI", "SR-PS-QS4-1507:setI", "SR-PS-QS3-1508:setI", "SR-PS-QS2-1509:setI", "SR-PS-QS1-1510:setI", "SR-PS-QS1-1601:setI", "SR-PS-QS2-1602:setI", "SR-PS-QS3-1603:setI", "SR-PS-QS4-1604:setI", "SR-PS-QS5-1605:setI", "SR-PS-QS5-1606:setI", "SR-PS-QS4-1607:setI", "SR-PS-QL3-1608:setI", "SR-PS-QL2-1609:setI", "SR-PS-QL1-1610:setI", "SR-PS-QL1-1701:setI", "SR-PS-QL2-1702:setI", "SR-PS-QL3-1703:setI", "SR-PS-QS4-1704:setI", "SR-PS-QS5-1705:setI", "SR-PS-QS5-1706:setI", "SR-PS-QS4-1707:setI", "SR-PS-QS3-1708:setI", "SR-PS-QS2-1709:setI", "SR-PS-QS1-1710:setI", "SR-PS-QS1-1801:setI", "SR-PS-QS2-1802:setI", "SR-PS-QS3-1803:setI", "SR-PS-QS4-1804:setI", "SR-PS-QS5-1805:setI", "SR-PS-QS5-1806:setI", "SR-PS-QS4-1807:setI", "SR-PS-QS3-1808:setI", "SR-PS-QS2-1809:setI", "SR-PS-QS1-1810:setI", "SR-PS-QS1-1901:setI", "SR-PS-QS2-1902:setI", "SR-PS-QS3-1903:setI", "SR-PS-QS4-1904:setI", "SR-PS-QS5-1905:setI", "SR-PS-QS5-1906:setI", "SR-PS-QS4-1907:setI", "SR-PS-QS3-1908:setI", "SR-PS-QS2-1909:setI", "SR-PS-QS1-1910:setI", "SR-PS-QS1-2001:setI", "SR-PS-QS2-2002:setI", "SR-PS-QS3-2003:setI", "SR-PS-QS4-2004:setI", "SR-PS-QS5-2005:setI", "SR-PS-QS5-2006:setI", "SR-PS-QS4-2007:setI", "SR-PS-QL3-2008:setI", "SR-PS-QL2-2009:setI", "SR-PS-QL1-2010:setI", "SR-PS-QL1-2101:setI", "SR-PS-QL2-2102:setI", "SR-PS-QL3-2103:setI", "SR-PS-QS4-2104:setI", "SR-PS-QS5-2105:setI", "SR-PS-QS5-2106:setI", "SR-PS-QS4-2107:setI", "SR-PS-QS3-2108:setI", "SR-PS-QS2-2109:setI", "SR-PS-QS1-2110:setI", "SR-PS-QS1-2201:setI", "SR-PS-QS2-2202:setI", "SR-PS-QS3-2203:setI", "SR-PS-QS4-2204:setI", "SR-PS-QS5-2205:setI", "SR-PS-QS5-2206:setI", "SR-PS-QS4-2207:setI", "SR-PS-QS3-2208:setI", "SR-PS-QS2-2209:setI", "SR-PS-QS1-2210:setI", "SR-PS-QS1-2301:setI", "SR-PS-QS2-2302:setI", "SR-PS-QS3-2303:setI", "SR-PS-QS4-2304:setI", "SR-PS-QS5-2305:setI", "SR-PS-QS5-2306:setI", "SR-PS-QS4-2307:setI", "SR-PS-QS3-2308:setI", "SR-PS-QS2-2309:setI", "SR-PS-QS1-2310:setI", "SR-PS-QS1-2401:setI", "SR-PS-QS2-2402:setI", "SR-PS-QS3-2403:setI", "SR-PS-QS4-2404:setI", "SR-PS-QS5-2405:setI", "SR-PS-QS5-2406:setI", "SR-PS-QS4-2407:setI", "SR-PS-QL3-2408:setI", "SR-PS-QL2-2409:setI", "SR-PS-QL1-2410:setI", "SR-PS-S1-011:setI", "SR-PS-S2-012:setI", "SR-PS-SD-013:setI", "SR-PS-SF-014:setI", "SR-PS-SD-015:setI", "SR-PS-S4-016:setI", "SR-PS-S3-017:setI", "SR-PS-S5-021:setI", "SR-PS-S6-022:setI", "SR-PS-SD-023:setI", "SR-PS-SF-024:setI", "SR-PS-SD-025:setI", "SR-PS-S6-026:setI", "SR-PS-S5-027:setI", "SR-PS-S5-031:setI", "SR-PS-S6-032:setI", "SR-PS-SD-033:setI", "SR-PS-SF-034:setI", "SR-PS-SD-035:setI", "SR-PS-S6-036:setI", "SR-PS-S5-037:setI", "SR-PS-S3-041:setI", "SR-PS-S4-042:setI", "SR-PS-SD-043:setI", "SR-PS-SF-044:setI", "SR-PS-SD-045:setI", "SR-PS-S2-046:setI", "SR-PS-S1-047:setI", "SR-PS-S1-051:setI", "SR-PS-S2-052:setI", "SR-PS-SD-053:setI", "SR-PS-SF-054:setI", "SR-PS-SD-055:setI", "SR-PS-S4-056:setI", "SR-PS-S3-057:setI", "SR-PS-S5-061:setI", "SR-PS-S6-062:setI", "SR-PS-SD-063:setI", "SR-PS-SF-064:setI", "SR-PS-SD-065:setI", "SR-PS-S6-066:setI", "SR-PS-S5-067:setI", "SR-PS-S5-071:setI", "SR-PS-S6-072:setI", "SR-PS-SD-073:setI", "SR-PS-SF-074:setI", "SR-PS-SD-075:setI", "SR-PS-S6-076:setI", "SR-PS-S5-077:setI", "SR-PS-S3-081:setI", "SR-PS-S4-082:setI", "SR-PS-SD-083:setI", "SR-PS-SF-084:setI", "SR-PS-SD-085:setI", "SR-PS-S2-086:setI", "SR-PS-S1-087:setI", "SR-PS-S1-091:setI", "SR-PS-S2-092:setI", "SR-PS-SD-093:setI", "SR-PS-SF-094:setI", "SR-PS-SD-095:setI", "SR-PS-S4-096:setI", "SR-PS-S3-097:setI", "SR-PS-S5-101:setI", "SR-PS-S6-102:setI", "SR-PS-SD-103:setI", "SR-PS-SF-104:setI", "SR-PS-SD-105:setI", "SR-PS-S6-106:setI", "SR-PS-S5-107:setI", "SR-PS-S5-111:setI", "SR-PS-S6-112:setI", "SR-PS-SD-113:setI", "SR-PS-SF-114:setI", "SR-PS-SD-115:setI", "SR-PS-S6-116:setI", "SR-PS-S5-117:setI", "SR-PS-S3-121:setI", "SR-PS-S4-122:setI", "SR-PS-SD-123:setI", "SR-PS-SF-124:setI", "SR-PS-SD-125:setI", "SR-PS-S2-126:setI", "SR-PS-S1-127:setI", "SR-PS-S1-131:setI", "SR-PS-S2-132:setI", "SR-PS-SD-133:setI", "SR-PS-SF-134:setI", "SR-PS-SD-135:setI", "SR-PS-S4-136:setI", "SR-PS-S3-137:setI", "SR-PS-S5-141:setI", "SR-PS-S6-142:setI", "SR-PS-SD-143:setI", "SR-PS-SF-144:setI", "SR-PS-SD-145:setI", "SR-PS-S6-146:setI", "SR-PS-S5-147:setI", "SR-PS-S5-151:setI", "SR-PS-S6-152:setI", "SR-PS-SD-153:setI", "SR-PS-SF-154:setI", "SR-PS-SD-155:setI", "SR-PS-S6-156:setI", "SR-PS-S5-157:setI", "SR-PS-S3-161:setI", "SR-PS-S4-162:setI", "SR-PS-SD-163:setI", "SR-PS-SF-164:setI", "SR-PS-SD-165:setI", "SR-PS-S2-166:setI", "SR-PS-S1-167:setI", "SR-PS-S1-171:setI", "SR-PS-S2-172:setI", "SR-PS-SD-173:setI", "SR-PS-SF-174:setI", "SR-PS-SD-175:setI", "SR-PS-S4-176:setI", "SR-PS-S3-177:setI", "SR-PS-S5-181:setI", "SR-PS-S6-182:setI", "SR-PS-SD-183:setI", "SR-PS-SF-184:setI", "SR-PS-SD-185:setI", "SR-PS-S6-186:setI", "SR-PS-S5-187:setI", "SR-PS-S5-191:setI", "SR-PS-S6-192:setI", "SR-PS-SD-193:setI", "SR-PS-SF-194:setI", "SR-PS-SD-195:setI", "SR-PS-S6-196:setI", "SR-PS-S5-197:setI", "SR-PS-S3-201:setI", "SR-PS-S4-202:setI", "SR-PS-SD-203:setI", "SR-PS-SF-204:setI", "SR-PS-SD-205:setI", "SR-PS-S2-206:setI", "SR-PS-S1-207:setI", "SR-PS-S1-211:setI", "SR-PS-S2-212:setI", "SR-PS-SD-213:setI", "SR-PS-SF-214:setI", "SR-PS-SD-215:setI", "SR-PS-S4-216:setI", "SR-PS-S3-217:setI", "SR-PS-S5-221:setI", "SR-PS-S6-222:setI", "SR-PS-SD-223:setI", "SR-PS-SF-224:setI", "SR-PS-SD-225:setI", "SR-PS-S6-226:setI", "SR-PS-S5-227:setI", "SR-PS-S5-231:setI", "SR-PS-S6-232:setI", "SR-PS-SD-233:setI", "SR-PS-SF-234:setI", "SR-PS-SD-235:setI", "SR-PS-S6-236:setI", "SR-PS-S5-237:setI", "SR-PS-S3-241:setI", "SR-PS-S4-242:setI", "SR-PS-SD-243:setI", "SR-PS-SF-244:setI", "SR-PS-SD-245:setI", "SR-PS-S2-246:setI", "SR-PS-S1-247:setI", "SR-PS-SKEW-011:setI", "SR-PS-SKEW-012:setI", "SR-PS-SKEW-013:setI", "SR-PS-SKEW-014:setI", "SR-PS-SKEW-015:setI", "SR-PS-SKEW-016:setI", "SR-PS-SKEW-017:setI", "SR-PS-SKEW-021:setI", "SR-PS-SKEW-022:setI", "SR-PS-SKEW-023:setI", "SR-PS-SKEW-024:setI", "SR-PS-SKEW-025:setI", "SR-PS-SKEW-026:setI", "SR-PS-SKEW-027:setI", "SR-PS-SKEW-031:setI", "SR-PS-SKEW-032:setI", "SR-PS-SKEW-033:setI", "SR-PS-SKEW-034:setI", "SR-PS-SKEW-035:setI", "SR-PS-SKEW-036:setI", "SR-PS-SKEW-037:setI", "SR-PS-SKEW-041:setI", "SR-PS-SKEW-042:setI", "SR-PS-SKEW-043:setI", "SR-PS-SKEW-044:setI", "SR-PS-SKEW-045:setI", "SR-PS-SKEW-046:setI", "SR-PS-SKEW-047:setI", "SR-PS-SKEW-051:setI", "SR-PS-SKEW-052:setI", "SR-PS-SKEW-053:setI", "SR-PS-SKEW-054:setI", "SR-PS-SKEW-055:setI", "SR-PS-SKEW-056:setI", "SR-PS-SKEW-057:setI", "SR-PS-SKEW-061:setI", "SR-PS-SKEW-062:setI", "SR-PS-SKEW-063:setI", "SR-PS-SKEW-064:setI", "SR-PS-SKEW-065:setI", "SR-PS-SKEW-066:setI", "SR-PS-SKEW-067:setI", "SR-PS-SKEW-071:setI", "SR-PS-SKEW-072:setI", "SR-PS-SKEW-073:setI", "SR-PS-SKEW-074:setI", "SR-PS-SKEW-075:setI", "SR-PS-SKEW-076:setI", "SR-PS-SKEW-077:setI", "SR-PS-SKEW-081:setI", "SR-PS-SKEW-082:setI", "SR-PS-SKEW-083:setI", "SR-PS-SKEW-084:setI", "SR-PS-SKEW-085:setI", "SR-PS-SKEW-086:setI", "SR-PS-SKEW-087:setI", "SR-PS-SKEW-091:setI", "SR-PS-SKEW-092:setI", "SR-PS-SKEW-093:setI", "SR-PS-SKEW-094:setI", "SR-PS-SKEW-095:setI", "SR-PS-SKEW-096:setI", "SR-PS-SKEW-097:setI", "SR-PS-SKEW-101:setI", "SR-PS-SKEW-102:setI", "SR-PS-SKEW-103:setI", "SR-PS-SKEW-104:setI", "SR-PS-SKEW-105:setI", "SR-PS-SKEW-106:setI", "SR-PS-SKEW-107:setI", "SR-PS-SKEW-111:setI", "SR-PS-SKEW-112:setI", "SR-PS-SKEW-113:setI", "SR-PS-SKEW-114:setI", "SR-PS-SKEW-115:setI", "SR-PS-SKEW-116:setI", "SR-PS-SKEW-117:setI", "SR-PS-SKEW-121:setI", "SR-PS-SKEW-122:setI", "SR-PS-SKEW-123:setI", "SR-PS-SKEW-124:setI", "SR-PS-SKEW-125:setI", "SR-PS-SKEW-126:setI", "SR-PS-SKEW-127:setI", "SR-PS-SKEW-131:setI", "SR-PS-SKEW-132:setI", "SR-PS-SKEW-133:setI", "SR-PS-SKEW-134:setI", "SR-PS-SKEW-135:setI", "SR-PS-SKEW-136:setI", "SR-PS-SKEW-137:setI", "SR-PS-SKEW-141:setI", "SR-PS-SKEW-142:setI", "SR-PS-SKEW-143:setI", "SR-PS-SKEW-144:setI", "SR-PS-SKEW-145:setI", "SR-PS-SKEW-146:setI", "SR-PS-SKEW-147:setI", "SR-PS-SKEW-151:setI", "SR-PS-SKEW-152:setI", "SR-PS-SKEW-153:setI", "SR-PS-SKEW-154:setI", "SR-PS-SKEW-155:setI", "SR-PS-SKEW-156:setI", "SR-PS-SKEW-157:setI", "SR-PS-SKEW-161:setI", "SR-PS-SKEW-162:setI", "SR-PS-SKEW-163:setI", "SR-PS-SKEW-164:setI", "SR-PS-SKEW-165:setI", "SR-PS-SKEW-166:setI", "SR-PS-SKEW-167:setI", "SR-PS-SKEW-171:setI", "SR-PS-SKEW-172:setI", "SR-PS-SKEW-173:setI", "SR-PS-SKEW-174:setI", "SR-PS-SKEW-175:setI", "SR-PS-SKEW-176:setI", "SR-PS-SKEW-177:setI", "SR-PS-SKEW-181:setI", "SR-PS-SKEW-182:setI", "SR-PS-SKEW-183:setI", "SR-PS-SKEW-184:setI", "SR-PS-SKEW-185:setI", "SR-PS-SKEW-186:setI", "SR-PS-SKEW-187:setI", "SR-PS-SKEW-191:setI", "SR-PS-SKEW-192:setI", "SR-PS-SKEW-193:setI", "SR-PS-SKEW-194:setI", "SR-PS-SKEW-195:setI", "SR-PS-SKEW-196:setI", "SR-PS-SKEW-197:setI", "SR-PS-SKEW-201:setI", "SR-PS-SKEW-202:setI", "SR-PS-SKEW-203:setI", "SR-PS-SKEW-204:setI", "SR-PS-SKEW-205:setI", "SR-PS-SKEW-206:setI", "SR-PS-SKEW-207:setI", "SR-PS-SKEW-211:setI", "SR-PS-SKEW-212:setI", "SR-PS-SKEW-213:setI", "SR-PS-SKEW-214:setI", "SR-PS-SKEW-215:setI", "SR-PS-SKEW-216:setI", "SR-PS-SKEW-217:setI", "SR-PS-SKEW-221:setI", "SR-PS-SKEW-222:setI", "SR-PS-SKEW-223:setI", "SR-PS-SKEW-224:setI", "SR-PS-SKEW-225:setI", "SR-PS-SKEW-226:setI", "SR-PS-SKEW-227:setI", "SR-PS-SKEW-231:setI", "SR-PS-SKEW-232:setI", "SR-PS-SKEW-233:setI", "SR-PS-SKEW-234:setI", "SR-PS-SKEW-235:setI", "SR-PS-SKEW-236:setI", "SR-PS-SKEW-237:setI", "SR-PS-SKEW-241:setI", "SR-PS-SKEW-242:setI", "SR-PS-SKEW-243:setI", "SR-PS-SKEW-244:setI", "SR-PS-SKEW-245:setI", "SR-PS-SKEW-246:setI", "SR-PS-SKEW-247:setI", "SR-RF2-LLRF:setGapVoltage", "SR-RF2-LLRF:setStationPhase", "SR-RF3-LLRF:setGapVoltage", "SR-RF3-LLRF:setStationPhase", "SR-PS-DMB09-Q1:setI", "SR-PS-DMB09-Q2:setI", "SR-PS-DMB09-Q3:setI", "SR-PS-DMB25-Q1:setI", "SR-PS-DMB25-Q2:setI", "SR-PS-DMB25-Q3:setI", "SR-PS-DMB41-Q1:setI", "SR-PS-DMB41-Q2:setI", "SR-PS-DMB41-Q3:setI", "SR-PS-DMB09-HC1:setI", "SR-PS-DMB09-HC2:setI", "SR-PS-DMB09-VC1:setI", "SR-PS-DMB09-VC2:setI", "SR-PS-DMB25-HC1:setI", "SR-PS-DMB25-HC2:setI", "SR-PS-DMB25-VC1:setI", "SR-PS-DMB25-VC2:setI", "SR-PS-DMB41-HC1:setI", "SR-PS-DMB41-HC2:setI", "SR-PS-DMB41-VC1:setI", "SR-PS-DMB41-VC2:setI", "SR-ID-IU22-05:setGap", "SR-ID-IU22A-09:setGap", "SR-ID-IU22B-09:setGap", "SR-ID-IUT22-21:setGap", "SR-ID-IU22-23:setGap", "SR-ID-IU22A-25:setGap", "SR-ID-IU22B-25:setGap", "SR-ID-EPU48A-41:setGap", "SR-ID-EPU48A-41:setPhase", "SR-ID-EPU48B-41:setGap", "SR-ID-EPU48B-41:setPhase", "SR-ID-EPU46-45:setGap", "SR-ID-EPU46-45:setPhase", "SR-ID-IUT22-21:setGapTaper", "SR-ID-EPU48PS-41:setGap", "SR-ID-IU22-05:gapMotorOff", "SR-ID-IU22A-09:gapMotorOff", "SR-ID-IU22B-09:gapMotorOff", "SR-ID-IUT22-21:gapMotorOff", "SR-ID-IU22-23:gapMotorOff", "SR-ID-IU22A-25:gapMotorOff", "SR-ID-IU22B-25:gapMotorOff", "SR-ID-EPU48A-41:gapMotorOff", "SR-ID-EPU48B-41:gapMotorOff", "SR-ID-EPU46-45:gapMotorOff", "SR-ID-EPU48A-41:phaseMotorOff", "SR-ID-EPU48B-41:phaseMotorOff", "SR-ID-EPU46-45:phaseMotorOff", "SR-DI-FOFB-H:setStatus", "SR-DI-FOFB-V:setStatus", "IGPF:TPSX:FBCTRL", "IGPF:TPSY:FBCTRL", "TPS-SR-022:bpm3:ilk:enabled", "SR-DI-ANGLE-ILK:StatusX", "SR-DI-ANGLE-ILK:StatusY", "SR-DI-RF-FB:setStatus", "SR-ID-EPU48-TFF:status", "SR-ID-EPU48-CFF:status", "SR-ID-EPU46-TFF:status", "SR-ID-EPU46-CFF:status", "TI-INJ-PROC:TopupHiLowStart"]
  out "error out 5":errorcluster
  out "error out 4":errorcluster
  out "result":string="Beam Trip Events \nTatal Counts: 0"
  in  "last ? Hrs":dbl=12.0 min=1.0 max=24.0 step=1.0
  in  "Trip Evt B":bool
  in  "Show Check list Button":bool=TRUE
  in  "View Diff Button":bool
  in  "Save Lattice Button":bool
  in  "Refresh B":bool
  out "x = y?":bool
  out "NOW time":string="15:45:10"
  out "NOW date":string="2017/10/28"
  in  "Save Button":bool
  out "error out 3":errorcluster
  in  "stop":bool
  out "time kickeron":string="15:43:52"
  out "date kickeron":string="2017/10/28"
  out "Orbit ILK(A)":bool
  out "Orbit INT. Ang Active":bool
  out "Orbit INT.Ang. On":bool
  out "Orbit INT. Pos Active":bool
  out "Orbit INT.Pos. On":bool
  in  "Copy Button":bool
  in  "Print Button":bool
  in  "Help Button":bool
  in  "Open Button":bool
  # "TPS OP Handover Information"
  # "Others"
  # "Additional Functions"
  # "Time："
  # "follow"
  # "歷史電流圖\ntrip次數?\n輻射劑量?\n平均氣壓\n目前最高累計劑量\n最近一次觸發時BR電流及WCM數值"
  # "Valve  Status"
  # "TFF"
  # "CFF"
  # "SM Status"
  # "TPS Operational Handover Information v1.4.5"
  # "SR Status"
  # "Feedback"
  # "Pulse Mag"
  # "LINAC"
  # "x8(ns)"
  # "x2(ns)"
  # "x0.01(ns)"
  # "RF Status"
  # "Hz"
  # "(kV)"
  # "(kV)"
  # "Changeliang@LOP.NSRRC"
  # "SR Fill Pattern"
  # "Lattice Files in Using"
  # "ID &Beamline (R)"
  # "mode"
  # "Gap\nmm"
  # "Motor"
  # "Phase"
  # "FE/Hutch"
  # "Phase\nShifter"
  # "XBPM1X\num"
  # "XBPM1Y\num"
  # "XBPM2X\num"
  # "XBPM2Y\num"
  # "Note"
  # "05"
  # "09"
  # "Taper(enc)"
  # "21"
  # "23"
  # "25"
  # "41"
  # "45"
  # "SR Orbit"
  # "BPMX"
  # "BPMY"
  # "SR Beam Current History"
  # "ns"
  # "threshold:0.05mA"
  # "Adjusted History\n#Note: This file recorded PVs(set values) that were changed during this time.\n#(RF frequency was not recorded in this file)"
  # "Event Time"
  # "PV_name"
  # "Ori_Value"
  # "New_Value"
  # "hrs"
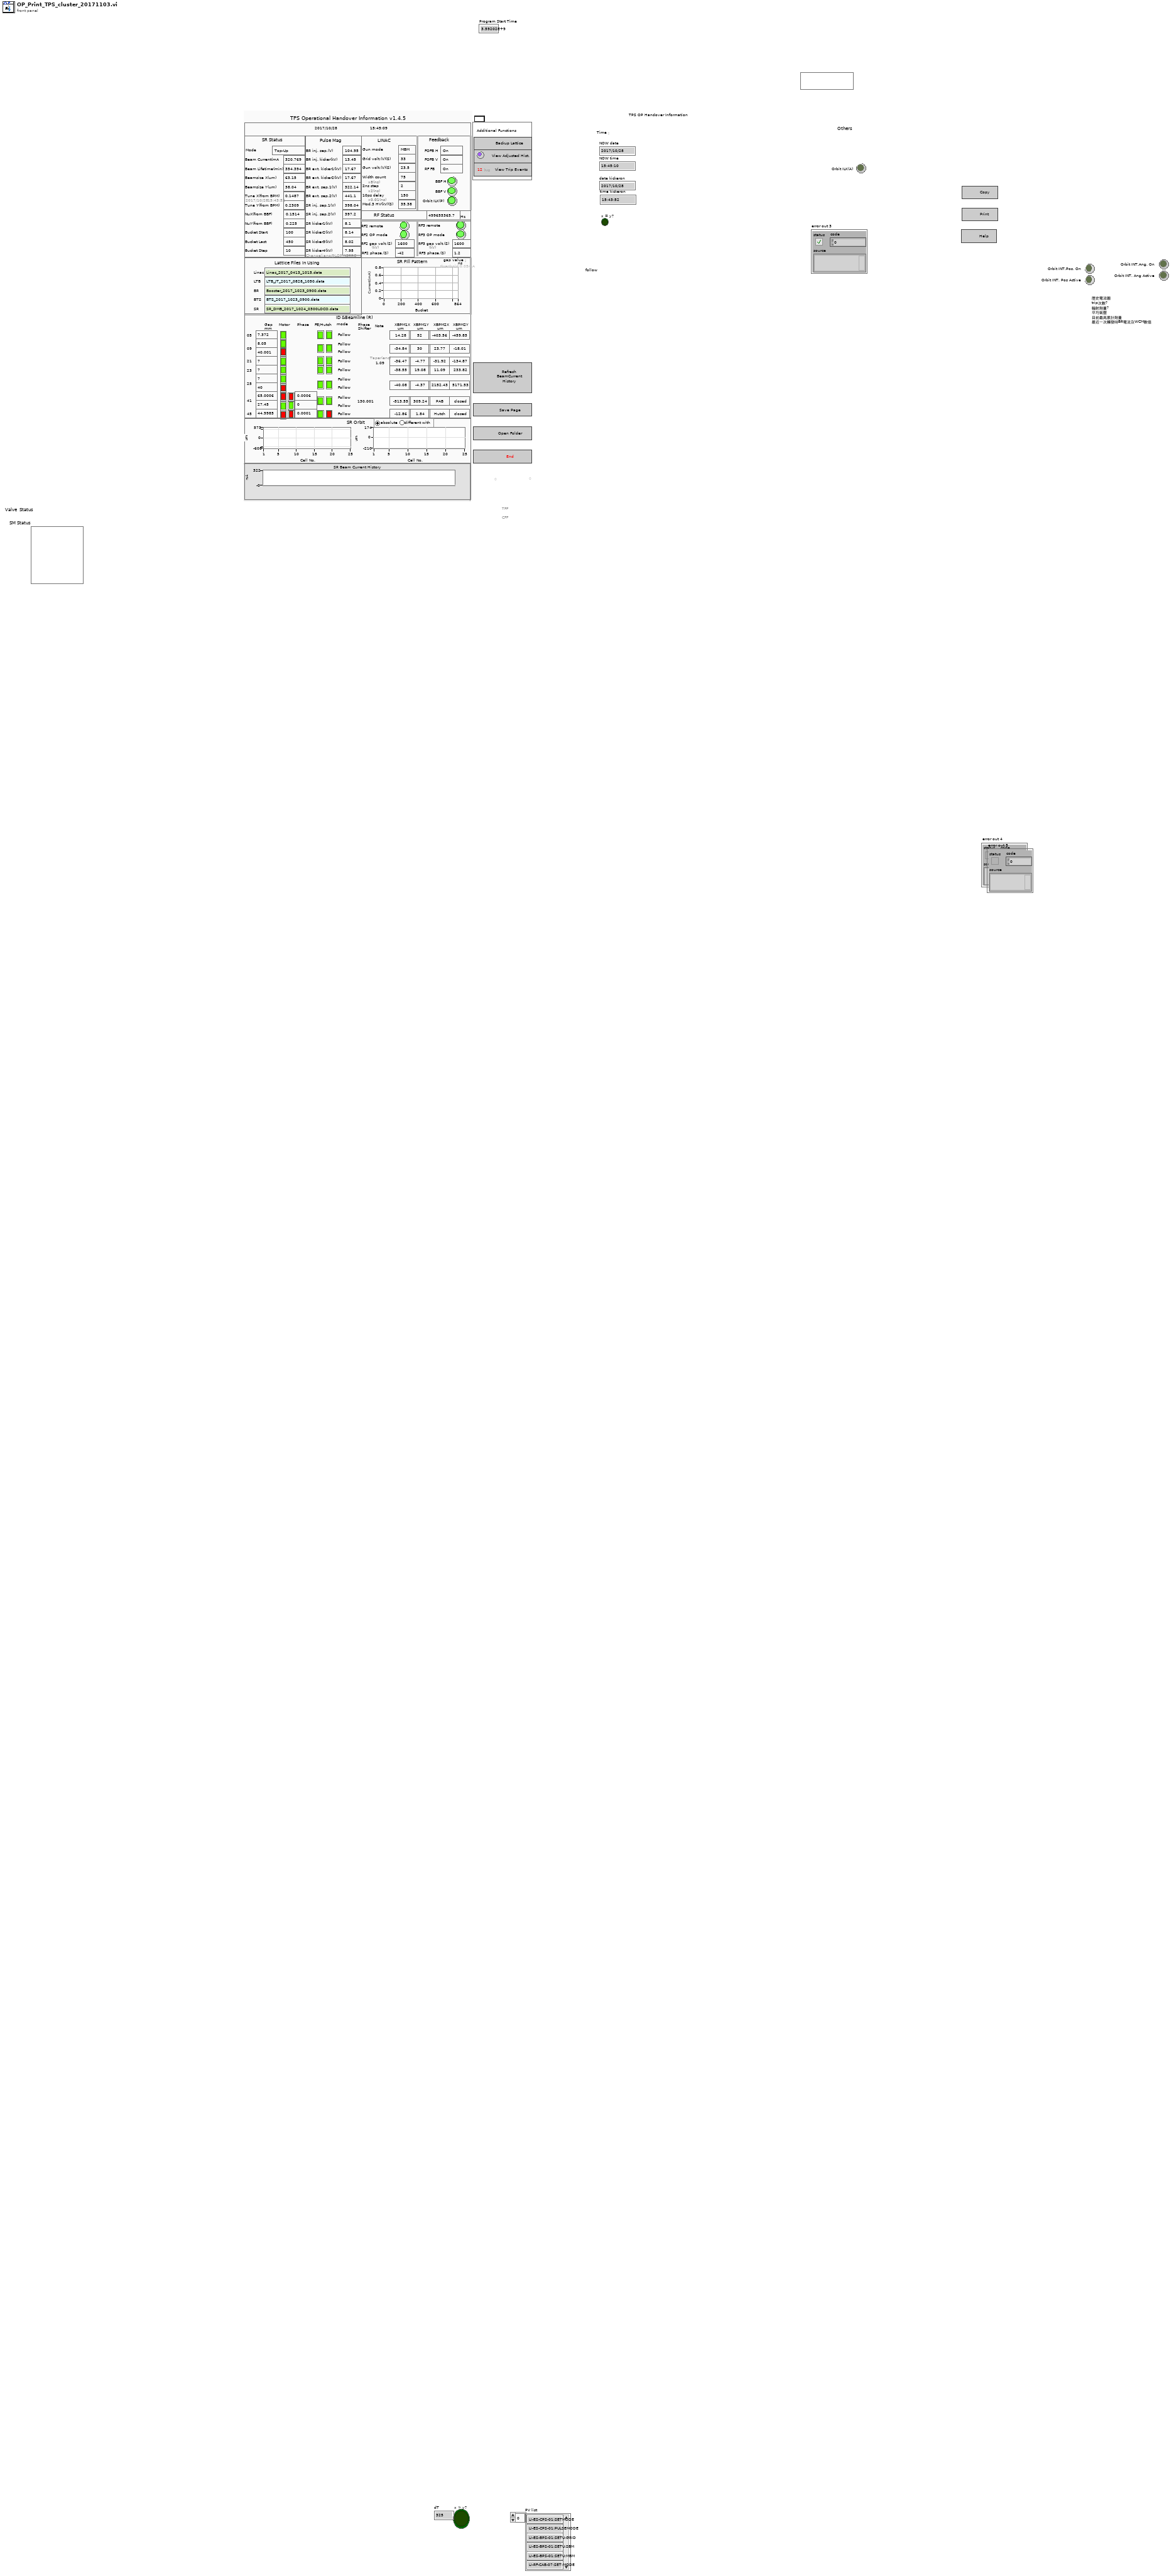
[diagram p1: front panel]
types:
  T1 = cluster{"SR Fill Pattern":dbl[], "Beam Current(mA":dbl, "Beam Lifetime(min)":dbl, "Beamsize X(um)":dbl, "Beamsize Y(um)":dbl, "Tune X(from BPM)":dbl, "Tune Y(from BPM)":dbl, "Mode":string, "NuX(from BBF) ":dbl, "NuY(from BBF)":dbl, "IU22-23gap(R)":dbl, "IU22-05gap(R)":dbl, "IU22-05M":bool, "IU22A-09gap(R)":dbl, "IU22A-09M":bool, "IU22B-09gap(R)":dbl, "IU22B-09M":bool, "IUT22-21gap(R)":dbl, "IUT22-21M":bool, "IU22-23M":bool, "IU22A-25gap(R)":dbl, "IU22A-25M":bool, "IU22B-25gap(R)":dbl, "IU22B-25M":bool, "EPU48A-41gap(R)":dbl, "EPU48A-41gM":bool, "EPU48B-41gap(R)":dbl, "EPU48B-41gM":bool, "EPU46-45gap(R)":dbl, "EPU46-45gM":bool, "EPU48A-41phase(R)":dbl, "EPU48B-41phase(R)":dbl, "EPU46-45phase(R)":dbl, "Grid volt.(V)(S)":dbl, "Gun mode":string, "Mod.3 HV(kV)(S)":dbl, "SR":string, "BR":string, "Linac":string, "LTB":string, "BTS":string, "RF2 remote":bool, "RF2 OP mode":bool, "RF2 phase.(S)":dbl, "RF Freq.(s)":dbl, "RF2 gap volt.(S)":dbl, "RF3 remote":bool, "RF3 OP mode":bool, "RF3 phase.(S)":dbl, "RF3 gap volt.(S)":dbl, "BBF V":bool, "BBF H":bool, "BR ext. kicker1(kV)":dbl, "BR ext. kicker2(kV)":dbl, "BR ext. sep.1(V)":dbl, "BR ext. sep.2(V)":dbl, "BR inj. sep.(V)":dbl, "BR inj. kicker(kV)":dbl, "SR kicker4(kV)":dbl, "SR kicker3(kV)":dbl, "SR kicker2(kV)":dbl, "SR kicker1(kV)":dbl, "SR inj. sep.2(V)":dbl, "SR inj. sep.1(V)":dbl, "Bucket Start":dbl, "Bucket Last":dbl, "Bucket Step":dbl, "Orbit ILK(P)":bool, "IU22-05 Hutch Enable":bool, "IU22A-09M Hutch Enable":bool, "IUT22-21M Hutch Enable":bool, "IU22-23M Hutch Enable":bool, "IU22A-25M Hutch Enable":bool, "EPU48A-41M Hutch Enable":bool, "EPU46-45M Hutch Enable":bool, "EPU46-45 FE Enable":bool, "EPU48A-41 FE Enable":bool, "IU22A-25 FE Enable":bool, "IU22-23 FE Enable":bool, "IUT22-21 FE Enable":bool, "IU22A-09 FE Enable":bool, "IU22-05 FE Enable":bool, "EPU48A-41pM":bool, "EPU48B-41pM":bool, "EPU46-45pM":bool, "Gun volt.(V)(S)":dbl, "Width count":dbl, "2ns step":dbl, "10ps delay":dbl, "phase shifter":dbl, "Taper":dbl, "05XBPMX 1":dbl, "09XBPMX 1":dbl, "21XBPMX 1":dbl, "23XBPMX 1":dbl, "25XBPMX 1":dbl, "41XBPMX 1":dbl, "45XBPMX 1":dbl, "05XBPMY 1":dbl, "09XBPMY 1":dbl, "21XBPMY 1":dbl, "23XBPMY 1":dbl, "25XBPMY 1":dbl, "41XBPMY 1":dbl, "45XBPMY 1":dbl, "FOFB H":string, "FOFB V":string, "time string":string, "date":string, "date (last kicker ON)":string, "time string (last kicker ON)":string, "Radio Buttons 2":enum32{"absolute", "different with"}, "09XBPMX 2":string, "09XBPMY 2":string, "05XBPMY 2":string, "05XBPMX 2":string, "21XBPMY 2":string, "21XBPMX 2":string, "23XBPMY 2":string, "23XBPMX 2":string, "25XBPMY 2":string, "25XBPMX 2":string, "41XBPMY 2":string, "41XBPMX 2":string, "45XBPMX 2":string, "45XBPMY 2":string, "05 mode":string, "09A mode":string, "09B mode":string, "21 mode":string, "23 mode":string, "25A mode":string, "25B mode":string, "41A mode":string, "41B mode":string, "46 mode":string, "BeamCurrent History":cluster{"BPM NO.  1_172":dbl[], dbl[]}, "SR Beam Current in            hours":dbl, "RF FB":string, "BPMX Graph 2":cluster{"Array of X axis  平均分配至各段":dbl[], dbl[]}, "BPMY Graph 2":cluster{"Array of X axis  平均分配至各段":dbl[], dbl[]}, "gap value：":i32}
  T2 = typedef "NI_Database_API.lvlib/Conn ObjectReference.ctl" = refnum<k1>
  T3 = typedef "NI_Database_API.lvlib/Rec ObjectReference.ctl" = refnum<k1>
  T4 = typedef "imagedata.ctl" = cluster{"image type":i32, "image depth":i32, "image":u8[], "mask":u8[], "colors":u32[], "Rectangle":cluster{"left":i16, "top":i16, "right":i16, "bottom":i16}}
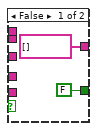
[diagram p2: hidden frame]
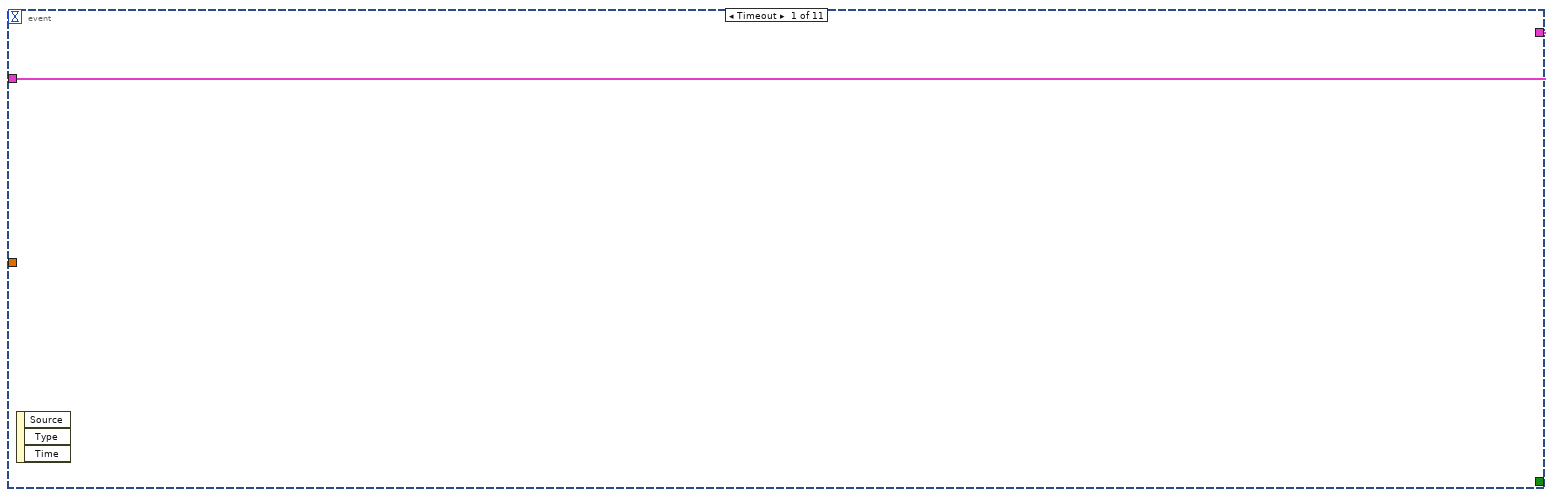
[diagram p4: hidden frame]
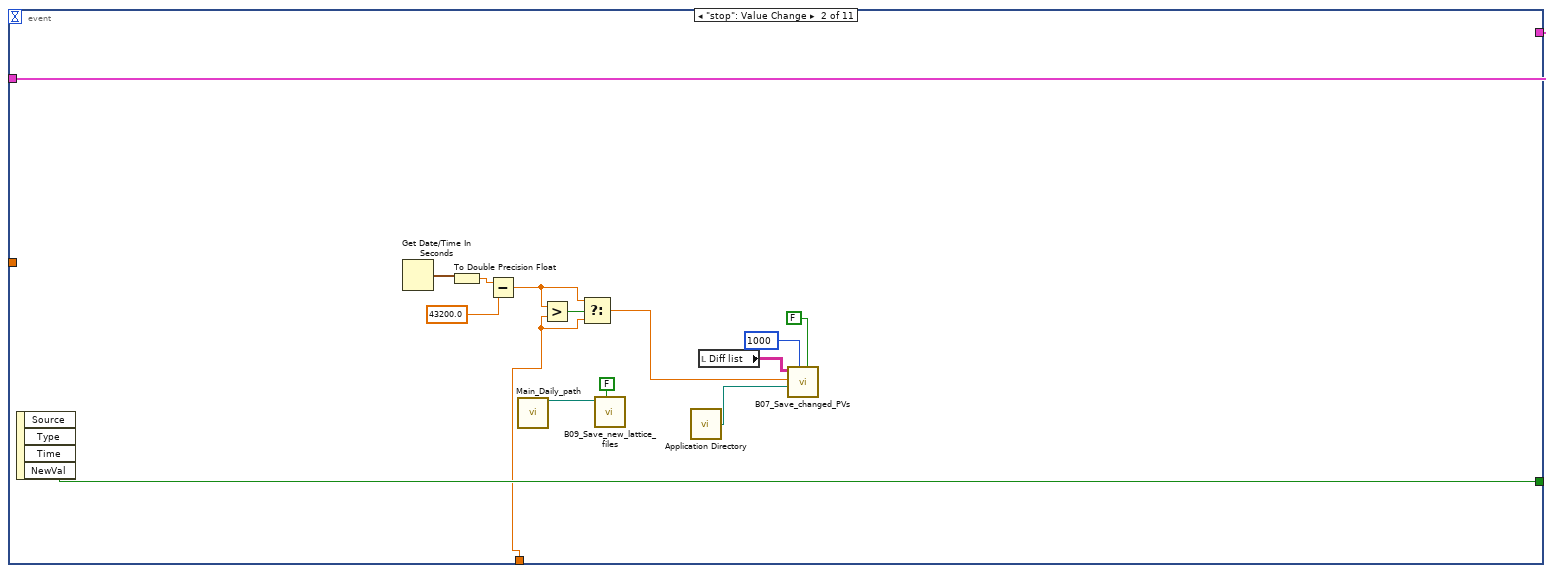
[diagram p5: hidden frame]
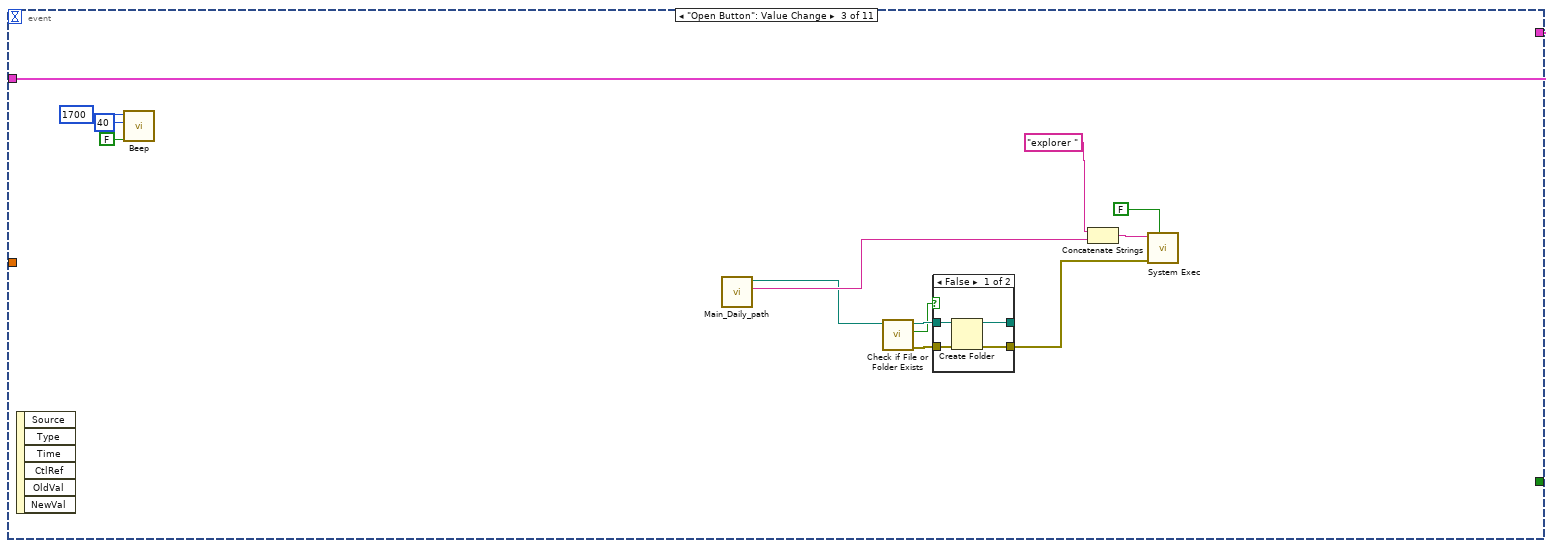
[diagram p6: hidden frame]
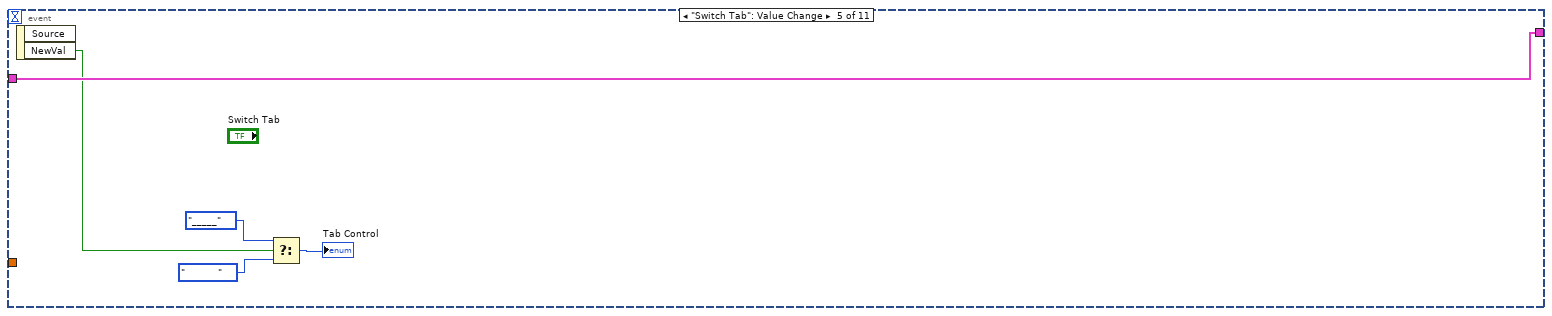
[diagram p9: hidden frame]
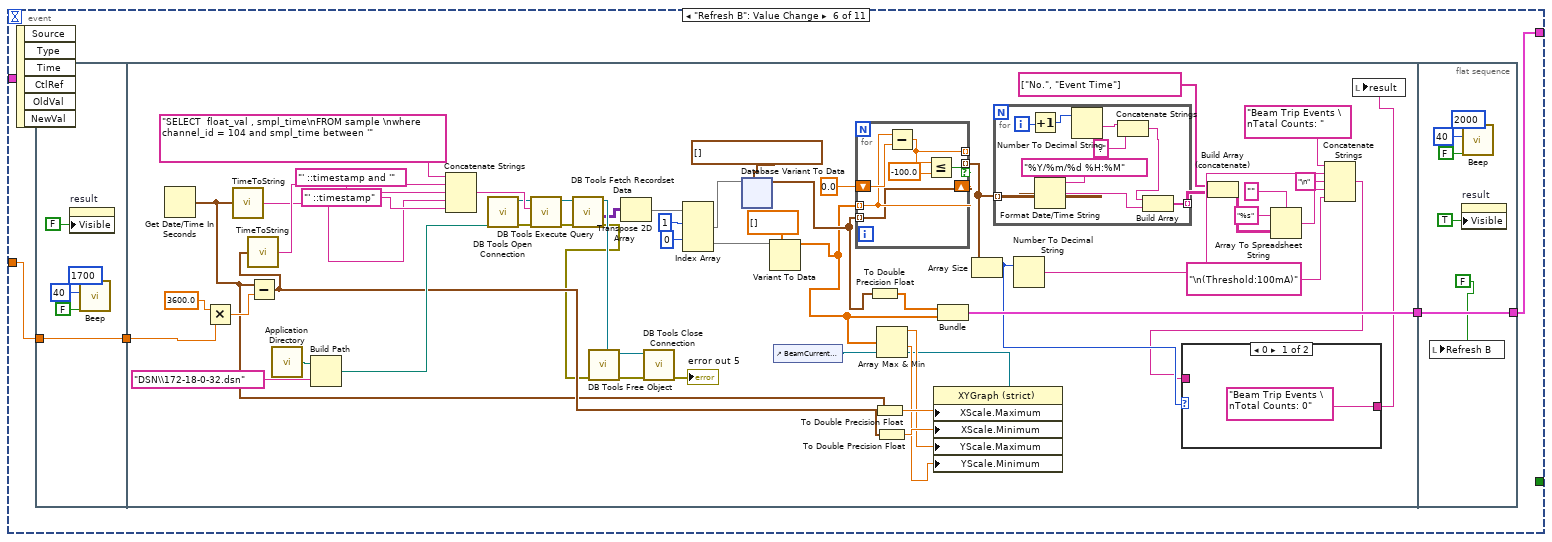
[diagram p10: hidden frame]
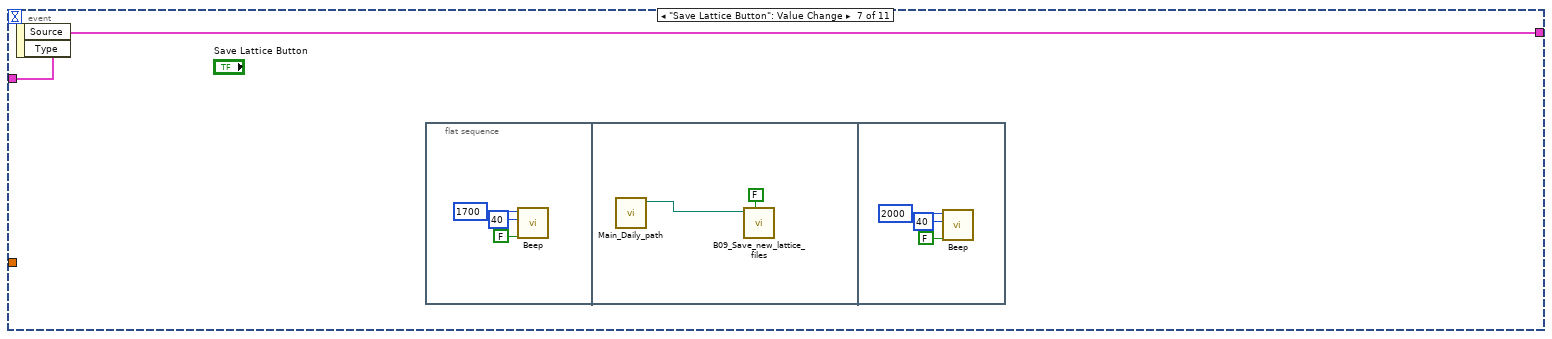
[diagram p12: hidden frame]
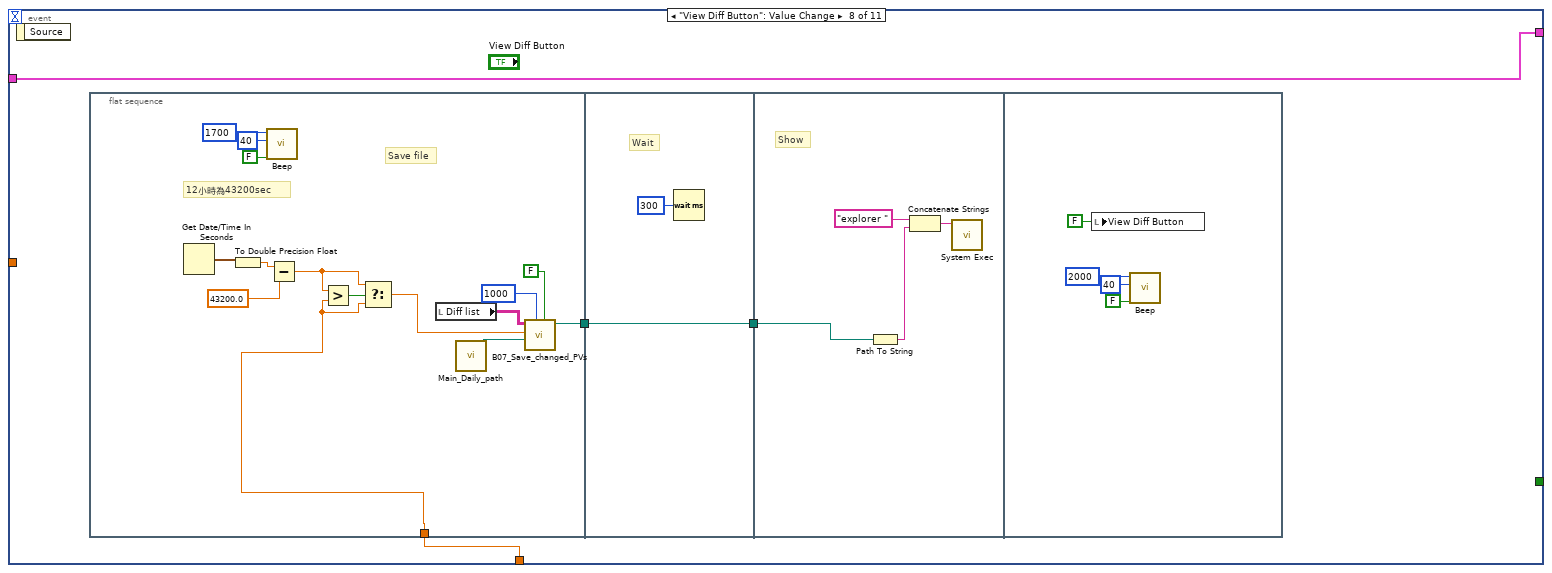
[diagram p13: hidden frame]
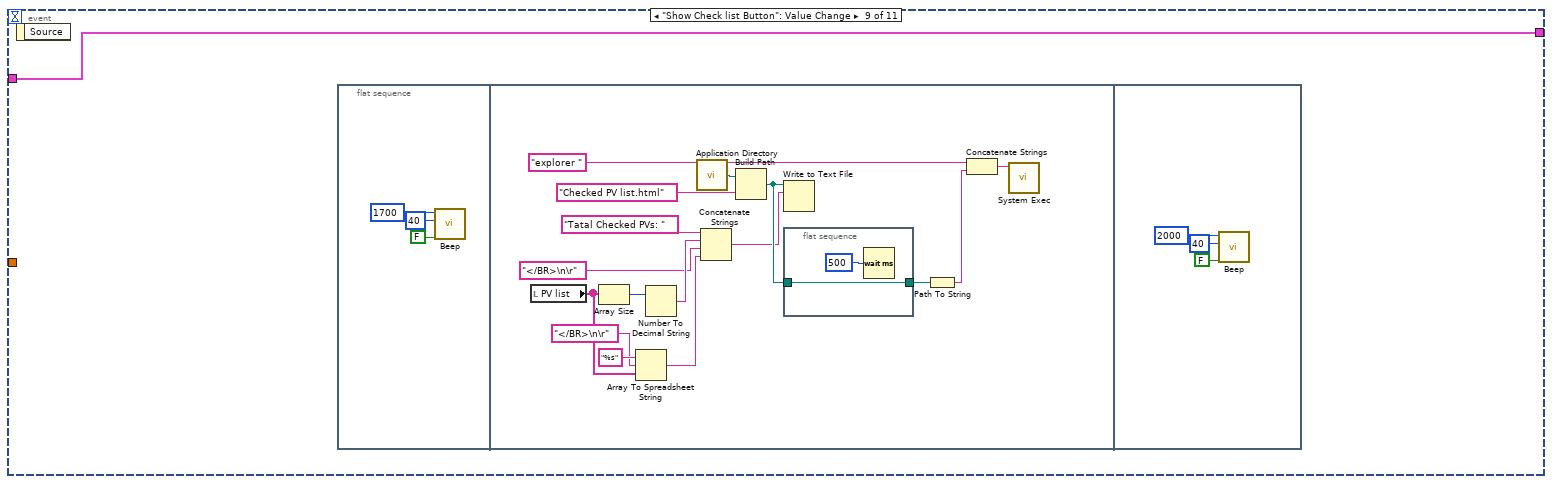
[diagram p14: hidden frame]
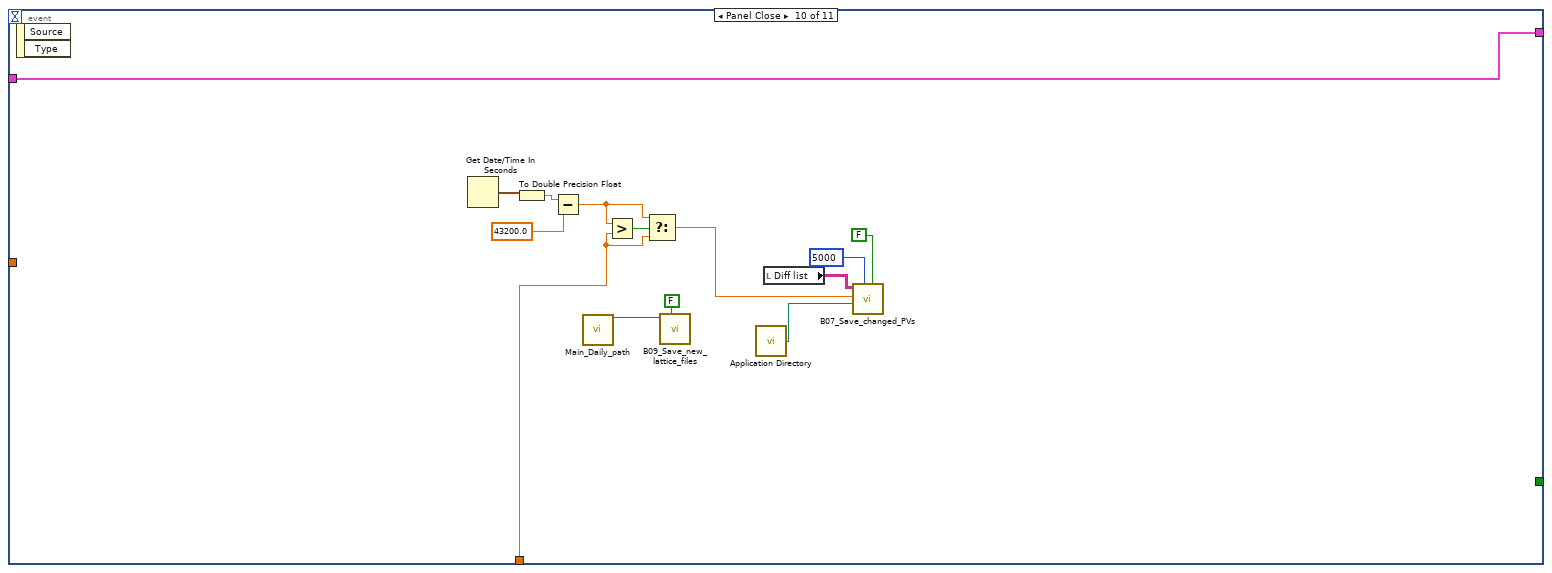
[diagram p15: hidden frame]
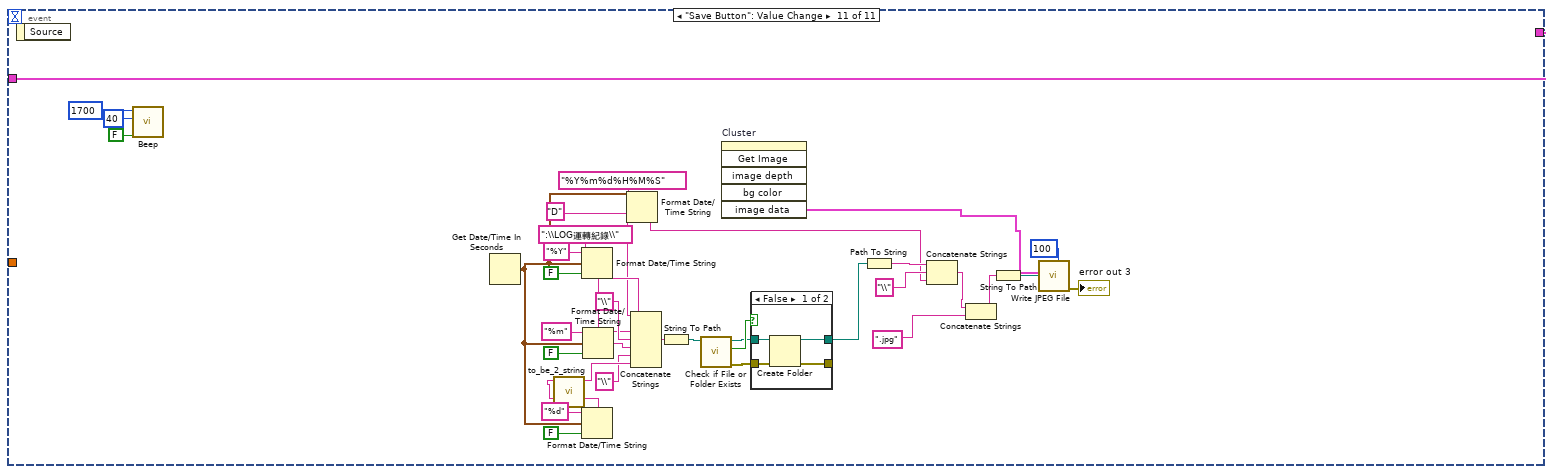
[diagram p16: hidden frame]
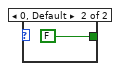
[diagram p18: hidden frame]
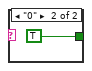
[diagram p19: hidden frame]
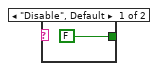
[diagram p20: hidden frame]
diagram:
  w1 = string[] ["SR-ID-IU22-05:setECMode", "SR-ID-IU22A-09:setECMode", "SR-ID-IU22B-09:setECMode", "SR-ID-IUT22-21:setECMode", "SR-ID-IU22-23:setECMode", "SR-ID-IU22A-25:setECMode", "SR-ID-IU22B-25:setECMode", "SR-ID-EPU48A-41:setECMode", "SR-ID-EPU48B-41:setECMode", "SR-ID-EPU46-45:setECMode"]  # ID_mode
  (unwired) "cpsc_037:AO:SLOW_SET:CH:3" ("regular expression")
  w2 = string[] ["LI-ES-CPS-01:SETMODE", "LI-ES-CPS-01:PULSEMODE", "LI-ES-BPS-01:SETU:GRID", "LI-ES-BPS-01:SETU:SBM", "LI-ES-BPS-01:SETU:MBM", "LI-RF-CAB-07:SET:MODE", "LI-RF-HVP-11:SET:U", "LI-RF-CAB-09:SET:MODE", "LI-RF-HVP-21:SET:U", "LI-RF-CAB-11:SET:MODE", "LI-RF-HVP-31:SET:U", "LI-RF-WGA-01:SET:POS", "LI-RF-WGA-02:SET:POS", "LI-RF-WGA-03:SET:POS", "LI-RF-SFT-01:SET:POS", "LI-RF-SFT-02:SET:POS", "LI-RF-SFT-03:SET:POS", "LI-RF-CTR-01:ES:SET:DEG", "LI-RF-CTR-01:SP:SET:DEG", "LI-RF-CTR-01:K123:SET:DEG", "LI-RF-CTR-01:K1:SET:DEG", "LI-RF-CTR-01:K3:SET:DEG", "LI-RF-AMP-01:SET:PWR", "LI-RF-AMP-02:SET:PWR", "LI-MA-SPS-01:SET:I", "LI-MA-SPS-02:SET:I", "LI-MA-SPS-03:SET:I", "LI-MA-SPS-04:SET:I", "LI-MA-SPS-05:SET:I", "LI-MA-SPS-06:SET:I", "LI-MA-SPS-07:SET:I", "LI-MA-SPS-08:SET:I", "LI-MA-SPS-09:SET:I", "LI-MA-SPS-10:SET:I", "LI-MA-SPS-11:SET:I", "LI-MA-SPS-12:SET:I", "LI-MA-SPS-13:SET:I", "LI-MA-SPS-14:SET:I", "LI-MA-SPS-15:SET:I", "LI-MA-SPS-16:SET:I", "LI-MA-STP-01:SET:I", "LI-MA-STP-02:SET:I", "LI-MA-STP-03:SET:I", "LI-MA-STP-04:SET:I", "LI-MA-STP-05:SET:I", "LI-MA-STP-06:SET:I", "LI-MA-STP-07:SET:I", "LI-MA-STP-08:SET:I", "LI-MA-STP-09:SET:I", "LI-MA-STP-10:SET:I", "LI-MA-STP-11:SET:I", "LI-MA-STP-12:SET:I", "LI-MA-STP-13:SET:I", "LI-MA-STP-14:SET:I", "LI-MA-STP-15:SET:I", "LI-MA-STP-16:SET:I", "LI-MA-QPS-01:SET:I", "LI-MA-QPS-02:SET:I", "LI-MA-QPS-03:SET:I", "LI-MA-QPS-04:SET:I", "LI-MA-QPS-05:SET:I", "LI-MA-QPS-06:SET:I", "CPCITM-TI-EVRTG:Pulse7DelaySet", "CPCITM-TI-EVRTG:Pulse7WidthSet", "CPCITM-TI-EVRTG:GTX7CtrlGTXPHSet", "CPCITM-TI-EVRTG:GTX7DlySet", "CPCITM-TI-EVRTG:Pulse6DelaySet", "CPCITM-TI-EVRTG:Pulse6WidthSet", "CPCITM-TI-EVRTG:GTX6DlySet", "CPCILI-TI-EVR:Pulse2DelaySet", "CPCILI-TI-EVR:Pulse2WidthSet", "CPCILI-TI-EVR:Pulse3DelaySet", "CPCILI-TI-EVR:Pulse3WidthSet", "CPCILI-TI-EVR:Pulse4DelaySet", "CPCILI-TI-EVR:Pulse4WidthSet", "CPCILI-TI-EVR:Pulse5DelaySet", "CPCILI-TI-EVR:Pulse5WidthSet", "CPCILI-TI-EVR:Pulse6DelaySet", "CPCILI-TI-EVR:Pulse6WidthSet", "CPCILI-TI-EVR:Pulse7DelaySet", "CPCILI-TI-EVR:Pulse7WidthSet", "CPCILI-TI-EVR:Pulse8DelaySet", "CPCILI-TI-EVR:Pulse8WidthSet", "CPCILI-TI-EVR:Pulse9DelaySet", "CPCILI-TI-EVR:Pulse9WidthSet", "CPCITM-TI-EVRTG:GTX6DlySet", "CPCITM-TI-EVRTG:GTX7DlySet"]  # PV nanes(LINAC) without 3 set
  w3 = string[] ["SR-DI-XPC-40:cam:AcquireTime", "SR-DI-XPC-40:cam:Gain"]  # Port40
  w4 = string[] ["LI:controlState0", "TI-INJ-PROC:trig-BRAC-ONOFF", "SR:controlState0"]  # Power Saving
  (unwired) "CPCITM-TI-EVRTG:GTX6CtrlGTXPHSet" ("regular expression")
  (unwired) "CPCITM-TI-EVRTG:GTX7CtrlGTXPHSet" ("regular expression")
  w6 = string[] ["SR-ID-IU22-05:setGap", "SR-ID-IU22A-09:setGap", "SR-ID-IU22B-09:setGap", "SR-ID-IUT22-21:setGap", "SR-ID-IU22-23:setGap", "SR-ID-IU22A-25:setGap", "SR-ID-IU22B-25:setGap", "SR-ID-EPU48A-41:setGap", "SR-ID-EPU48A-41:setPhase", "SR-ID-EPU48B-41:setGap", "SR-ID-EPU48B-41:setPhase", "SR-ID-EPU46-45:setGap", "SR-ID-EPU46-45:setPhase", "SR-ID-IUT22-21:setGapTaper", "SR-ID-EPU48PS-41:setGap"]  # PV nanes(ID gap_phase_Taper_)
  w17 = string[] ["TI-INJ-PROC:TopupHiLowStart", "TI-INJ-PROC:setBucketAddressStart", "TI-INJ-PROC:setBucketAddressLast", "TI-INJ-PROC:setBucketAddressStep", "TI-INJ-PROC:setPreCycle", "TI-INJ-PROC:setPostCycle", "TI-INJ-PROC:setBBeamCurrentTopupHi", "TI-INJ-PROC:setBBeamCurrentTopupLow"]  # PV nanes(Others)
  w16 = string[] ["SR-PS-BEND:setI", "SR-PS-HC-011:setI", "SR-PS-HC-012:setI", "SR-PS-HC-013:setI", "SR-PS-HC-014:setI", "SR-PS-HC-015:setI", "SR-PS-HC-016:setI", "SR-PS-HC-017:setI", "SR-PS-HC-021:setI", "SR-PS-HC-022:setI", "SR-PS-HC-023:setI", "SR-PS-HC-024:setI", "SR-PS-HC-025:setI", "SR-PS-HC-026:setI", "SR-PS-HC-027:setI", "SR-PS-HC-031:setI", "SR-PS-HC-032:setI", "SR-PS-HC-033:setI", "SR-PS-HC-034:setI", "SR-PS-HC-035:setI", "SR-PS-HC-036:setI", "SR-PS-HC-037:setI", "SR-PS-HC-041:setI", "SR-PS-HC-042:setI", "SR-PS-HC-043:setI", "SR-PS-HC-044:setI", "SR-PS-HC-045:setI", "SR-PS-HC-046:setI", "SR-PS-HC-047:setI", "SR-PS-HC-051:setI", "SR-PS-HC-052:setI", "SR-PS-HC-053:setI", "SR-PS-HC-054:setI", "SR-PS-HC-055:setI", "SR-PS-HC-056:setI", "SR-PS-HC-057:setI", "SR-PS-HC-061:setI", "SR-PS-HC-062:setI", "SR-PS-HC-063:setI", "SR-PS-HC-064:setI", "SR-PS-HC-065:setI", "SR-PS-HC-066:setI", "SR-PS-HC-067:setI", "SR-PS-HC-071:setI", "SR-PS-HC-072:setI", "SR-PS-HC-073:setI", "SR-PS-HC-074:setI", "SR-PS-HC-075:setI", "SR-PS-HC-076:setI", "SR-PS-HC-077:setI", "SR-PS-HC-081:setI", "SR-PS-HC-082:setI", "SR-PS-HC-083:setI", "SR-PS-HC-084:setI", "SR-PS-HC-085:setI", "SR-PS-HC-086:setI", "SR-PS-HC-087:setI", "SR-PS-HC-091:setI", "SR-PS-HC-092:setI", "SR-PS-HC-093:setI", "SR-PS-HC-094:setI", "SR-PS-HC-095:setI", "SR-PS-HC-096:setI", "SR-PS-HC-097:setI", "SR-PS-HC-101:setI", "SR-PS-HC-102:setI", "SR-PS-HC-103:setI", "SR-PS-HC-104:setI", "SR-PS-HC-105:setI", "SR-PS-HC-106:setI", "SR-PS-HC-107:setI", "SR-PS-HC-111:setI", "SR-PS-HC-112:setI", "SR-PS-HC-113:setI", "SR-PS-HC-114:setI", "SR-PS-HC-115:setI", "SR-PS-HC-116:setI", "SR-PS-HC-117:setI", "SR-PS-HC-121:setI", "SR-PS-HC-122:setI", "SR-PS-HC-123:setI", "SR-PS-HC-124:setI", "SR-PS-HC-125:setI", "SR-PS-HC-126:setI", "SR-PS-HC-127:setI", "SR-PS-HC-131:setI", "SR-PS-HC-132:setI", "SR-PS-HC-133:setI", "SR-PS-HC-134:setI", "SR-PS-HC-135:setI", "SR-PS-HC-136:setI", "SR-PS-HC-137:setI", "SR-PS-HC-141:setI", "SR-PS-HC-142:setI", "SR-PS-HC-143:setI", "SR-PS-HC-144:setI", "SR-PS-HC-145:setI", "SR-PS-HC-146:setI", "SR-PS-HC-147:setI", "SR-PS-HC-151:setI", "SR-PS-HC-152:setI", "SR-PS-HC-153:setI", "SR-PS-HC-154:setI", "SR-PS-HC-155:setI", "SR-PS-HC-156:setI", "SR-PS-HC-157:setI", "SR-PS-HC-161:setI", "SR-PS-HC-162:setI", "SR-PS-HC-163:setI", "SR-PS-HC-164:setI", "SR-PS-HC-165:setI", "SR-PS-HC-166:setI", "SR-PS-HC-167:setI", "SR-PS-HC-171:setI", "SR-PS-HC-172:setI", "SR-PS-HC-173:setI", "SR-PS-HC-174:setI", "SR-PS-HC-175:setI", "SR-PS-HC-176:setI", "SR-PS-HC-177:setI", "SR-PS-HC-181:setI", "SR-PS-HC-182:setI", "SR-PS-HC-183:setI", "SR-PS-HC-184:setI", "SR-PS-HC-185:setI", "SR-PS-HC-186:setI", "SR-PS-HC-187:setI", "SR-PS-HC-191:setI", "SR-PS-HC-192:setI", "SR-PS-HC-193:setI", "SR-PS-HC-194:setI", "SR-PS-HC-195:setI", "SR-PS-HC-196:setI", "SR-PS-HC-197:setI", "SR-PS-HC-201:setI", "SR-PS-HC-202:setI", "SR-PS-HC-203:setI", "SR-PS-HC-204:setI", "SR-PS-HC-205:setI", "SR-PS-HC-206:setI", "SR-PS-HC-207:setI", "SR-PS-HC-211:setI", "SR-PS-HC-212:setI", "SR-PS-HC-213:setI", "SR-PS-HC-214:setI", "SR-PS-HC-215:setI", "SR-PS-HC-216:setI", "SR-PS-HC-217:setI", "SR-PS-HC-221:setI", "SR-PS-HC-222:setI", "SR-PS-HC-223:setI", "SR-PS-HC-224:setI", "SR-PS-HC-225:setI", "SR-PS-HC-226:setI", "SR-PS-HC-227:setI", "SR-PS-HC-231:setI", "SR-PS-HC-232:setI", "SR-PS-HC-233:setI", "SR-PS-HC-234:setI", "SR-PS-HC-235:setI", "SR-PS-HC-236:setI", "SR-PS-HC-237:setI", "SR-PS-HC-241:setI", "SR-PS-HC-242:setI", "SR-PS-HC-243:setI", "SR-PS-HC-244:setI", "SR-PS-HC-245:setI", "SR-PS-HC-246:setI", "SR-PS-HC-247:setI", "SR-PS-VC-011:setI", "SR-PS-VC-012:setI", "SR-PS-VC-013:setI", "SR-PS-VC-014:setI", "SR-PS-VC-015:setI", "SR-PS-VC-016:setI", "SR-PS-VC-017:setI", "SR-PS-VC-021:setI", "SR-PS-VC-022:setI", "SR-PS-VC-023:setI", "SR-PS-VC-024:setI", "SR-PS-VC-025:setI", "SR-PS-VC-026:setI", "SR-PS-VC-027:setI", "SR-PS-VC-031:setI", "SR-PS-VC-032:setI", "SR-PS-VC-033:setI", "SR-PS-VC-034:setI", "SR-PS-VC-035:setI", "SR-PS-VC-036:setI", "SR-PS-VC-037:setI", "SR-PS-VC-041:setI", "SR-PS-VC-042:setI", "SR-PS-VC-043:setI", "SR-PS-VC-044:setI", "SR-PS-VC-045:setI", "SR-PS-VC-046:setI", "SR-PS-VC-047:setI", "SR-PS-VC-051:setI", "SR-PS-VC-052:setI", "SR-PS-VC-053:setI", "SR-PS-VC-054:setI", "SR-PS-VC-055:setI", "SR-PS-VC-056:setI", "SR-PS-VC-057:setI", "SR-PS-VC-061:setI", "SR-PS-VC-062:setI", "SR-PS-VC-063:setI", "SR-PS-VC-064:setI", "SR-PS-VC-065:setI", "SR-PS-VC-066:setI", "SR-PS-VC-067:setI", "SR-PS-VC-071:setI", "SR-PS-VC-072:setI", "SR-PS-VC-073:setI", "SR-PS-VC-074:setI", "SR-PS-VC-075:setI", "SR-PS-VC-076:setI", "SR-PS-VC-077:setI", "SR-PS-VC-081:setI", "SR-PS-VC-082:setI", "SR-PS-VC-083:setI", "SR-PS-VC-084:setI", "SR-PS-VC-085:setI", "SR-PS-VC-086:setI", "SR-PS-VC-087:setI", "SR-PS-VC-091:setI", "SR-PS-VC-092:setI", "SR-PS-VC-093:setI", "SR-PS-VC-094:setI", "SR-PS-VC-095:setI", "SR-PS-VC-096:setI", "SR-PS-VC-097:setI", "SR-PS-VC-101:setI", "SR-PS-VC-102:setI", "SR-PS-VC-103:setI", "SR-PS-VC-104:setI", "SR-PS-VC-105:setI", "SR-PS-VC-106:setI", "SR-PS-VC-107:setI", "SR-PS-VC-111:setI", "SR-PS-VC-112:setI", "SR-PS-VC-113:setI", "SR-PS-VC-114:setI", "SR-PS-VC-115:setI", "SR-PS-VC-116:setI", "SR-PS-VC-117:setI", "SR-PS-VC-121:setI", "SR-PS-VC-122:setI", "SR-PS-VC-123:setI", "SR-PS-VC-124:setI", "SR-PS-VC-125:setI", "SR-PS-VC-126:setI", "SR-PS-VC-127:setI", "SR-PS-VC-131:setI", "SR-PS-VC-132:setI", "SR-PS-VC-133:setI", "SR-PS-VC-134:setI", "SR-PS-VC-135:setI", "SR-PS-VC-136:setI", "SR-PS-VC-137:setI", "SR-PS-VC-141:setI", "SR-PS-VC-142:setI", "SR-PS-VC-143:setI", "SR-PS-VC-144:setI", "SR-PS-VC-145:setI", "SR-PS-VC-146:setI", "SR-PS-VC-147:setI", "SR-PS-VC-151:setI", "SR-PS-VC-152:setI", "SR-PS-VC-153:setI", "SR-PS-VC-154:setI", "SR-PS-VC-155:setI", "SR-PS-VC-156:setI", "SR-PS-VC-157:setI", "SR-PS-VC-161:setI", "SR-PS-VC-162:setI", "SR-PS-VC-163:setI", "SR-PS-VC-164:setI", "SR-PS-VC-165:setI", "SR-PS-VC-166:setI", "SR-PS-VC-167:setI", "SR-PS-VC-171:setI", "SR-PS-VC-172:setI", "SR-PS-VC-173:setI", "SR-PS-VC-174:setI", "SR-PS-VC-175:setI", "SR-PS-VC-176:setI", "SR-PS-VC-177:setI", "SR-PS-VC-181:setI", "SR-PS-VC-182:setI", "SR-PS-VC-183:setI", "SR-PS-VC-184:setI", "SR-PS-VC-185:setI", "SR-PS-VC-186:setI", "SR-PS-VC-187:setI", "SR-PS-VC-191:setI", "SR-PS-VC-192:setI", "SR-PS-VC-193:setI", "SR-PS-VC-194:setI", "SR-PS-VC-195:setI", "SR-PS-VC-196:setI", "SR-PS-VC-197:setI", "SR-PS-VC-201:setI", "SR-PS-VC-202:setI", "SR-PS-VC-203:setI", "SR-PS-VC-204:setI", "SR-PS-VC-205:setI", "SR-PS-VC-206:setI", "SR-PS-VC-207:setI", "SR-PS-VC-211:setI", "SR-PS-VC-212:setI", "SR-PS-VC-213:setI", "SR-PS-VC-214:setI", "SR-PS-VC-215:setI", "SR-PS-VC-216:setI", "SR-PS-VC-217:setI", "SR-PS-VC-221:setI", "SR-PS-VC-222:setI", "SR-PS-VC-223:setI", "SR-PS-VC-224:setI", "SR-PS-VC-225:setI", "SR-PS-VC-226:setI", "SR-PS-VC-227:setI", "SR-PS-VC-231:setI", "SR-PS-VC-232:setI", "SR-PS-VC-233:setI", "SR-PS-VC-234:setI", "SR-PS-VC-235:setI", "SR-PS-VC-236:setI", "SR-PS-VC-237:setI", "SR-PS-VC-241:setI", "SR-PS-VC-242:setI", "SR-PS-VC-243:setI", "SR-PS-VC-244:setI", "SR-PS-VC-245:setI", "SR-PS-VC-246:setI", "SR-PS-VC-247:setI", "SR-PS-QL1-0101:setI", "SR-PS-QL2-0102:setI", "SR-PS-QL3-0103:setI", "SR-PS-QS4-0104:setI", "SR-PS-QS5-0105:setI", "SR-PS-QS5-0106:setI", "SR-PS-QS4-0107:setI", "SR-PS-QS3-0108:setI", "SR-PS-QS2-0109:setI", "SR-PS-QS1-0110:setI", "SR-PS-QS1-0201:setI", "SR-PS-QS2-0202:setI", "SR-PS-QS3-0203:setI", "SR-PS-QS4-0204:setI", "SR-PS-QS5-0205:setI", "SR-PS-QS5-0206:setI", "SR-PS-QS4-0207:setI", "SR-PS-QS3-0208:setI", "SR-PS-QS2-0209:setI", "SR-PS-QS1-0210:setI", "SR-PS-QS1-0301:setI", "SR-PS-QS2-0302:setI", "SR-PS-QS3-0303:setI", "SR-PS-QS4-0304:setI", "SR-PS-QS5-0305:setI", "SR-PS-QS5-0306:setI", "SR-PS-QS4-0307:setI", "SR-PS-QS3-0308:setI", "SR-PS-QS2-0309:setI", "SR-PS-QS1-0310:setI", "SR-PS-QS1-0401:setI", "SR-PS-QS2-0402:setI", "SR-PS-QS3-0403:setI", "SR-PS-QS4-0404:setI", "SR-PS-QS5-0405:setI", "SR-PS-QS5-0406:setI", "SR-PS-QS4-0407:setI", "SR-PS-QL3-0408:setI", "SR-PS-QL2-0409:setI", "SR-PS-QL1-0410:setI", "SR-PS-QL1-0501:setI", "SR-PS-QL2-0502:setI", "SR-PS-QL3-0503:setI", "SR-PS-QS4-0504:setI", "SR-PS-QS5-0505:setI", "SR-PS-QS5-0506:setI", "SR-PS-QS4-0507:setI", "SR-PS-QS3-0508:setI", "SR-PS-QS2-0509:setI", "SR-PS-QS1-0510:setI", "SR-PS-QS1-0601:setI", "SR-PS-QS2-0602:setI", "SR-PS-QS3-0603:setI", "SR-PS-QS4-0604:setI", "SR-PS-QS5-0605:setI", "SR-PS-QS5-0606:setI", "SR-PS-QS4-0607:setI", "SR-PS-QS3-0608:setI", "SR-PS-QS2-0609:setI", "SR-PS-QS1-0610:setI", "SR-PS-QS1-0701:setI", "SR-PS-QS2-0702:setI", "SR-PS-QS3-0703:setI", "SR-PS-QS4-0704:setI", "SR-PS-QS5-0705:setI", "SR-PS-QS5-0706:setI", "SR-PS-QS4-0707:setI", "SR-PS-QS3-0708:setI", "SR-PS-QS2-0709:setI", "SR-PS-QS1-0710:setI", "SR-PS-QS1-0801:setI", "SR-PS-QS2-0802:setI", "SR-PS-QS3-0803:setI", "SR-PS-QS4-0804:setI", "SR-PS-QS5-0805:setI", "SR-PS-QS5-0806:setI", "SR-PS-QS4-0807:setI", "SR-PS-QL3-0808:setI", "SR-PS-QL2-0809:setI", "SR-PS-QL1-0810:setI", "SR-PS-QL1-0901:setI", "SR-PS-QL2-0902:setI", "SR-PS-QL3-0903:setI", "SR-PS-QS4-0904:setI", "SR-PS-QS5-0905:setI", "SR-PS-QS5-0906:setI", "SR-PS-QS4-0907:setI", "SR-PS-QS3-0908:setI", "SR-PS-QS2-0909:setI", "SR-PS-QS1-0910:setI", "SR-PS-QS1-1001:setI", "SR-PS-QS2-1002:setI", "SR-PS-QS3-1003:setI", "SR-PS-QS4-1004:setI", "SR-PS-QS5-1005:setI", "SR-PS-QS5-1006:setI", "SR-PS-QS4-1007:setI", "SR-PS-QS3-1008:setI", "SR-PS-QS2-1009:setI", "SR-PS-QS1-1010:setI", "SR-PS-QS1-1101:setI", "SR-PS-QS2-1102:setI", "SR-PS-QS3-1103:setI", "SR-PS-QS4-1104:setI", "SR-PS-QS5-1105:setI", "SR-PS-QS5-1106:setI", "SR-PS-QS4-1107:setI", "SR-PS-QS3-1108:setI", "SR-PS-QS2-1109:setI", "SR-PS-QS1-1110:setI", "SR-PS-QS1-1201:setI", "SR-PS-QS2-1202:setI", "SR-PS-QS3-1203:setI", "SR-PS-QS4-1204:setI", "SR-PS-QS5-1205:setI", "SR-PS-QS5-1206:setI", "SR-PS-QS4-1207:setI", "SR-PS-QL3-1208:setI", "SR-PS-QL2-1209:setI", "SR-PS-QL1-1210:setI", "SR-PS-QL1-1301:setI", "SR-PS-QL2-1302:setI", "SR-PS-QL3-1303:setI", "SR-PS-QS4-1304:setI", "SR-PS-QS5-1305:setI", "SR-PS-QS5-1306:setI", "SR-PS-QS4-1307:setI", "SR-PS-QS3-1308:setI", "SR-PS-QS2-1309:setI", "SR-PS-QS1-1310:setI", "SR-PS-QS1-1401:setI", "SR-PS-QS2-1402:setI", "SR-PS-QS3-1403:setI", "SR-PS-QS4-1404:setI", "SR-PS-QS5-1405:setI", "SR-PS-QS5-1406:setI", "SR-PS-QS4-1407:setI", "SR-PS-QS3-1408:setI", "SR-PS-QS2-1409:setI", "SR-PS-QS1-1410:setI", "SR-PS-QS1-1501:setI", "SR-PS-QS2-1502:setI", "SR-PS-QS3-1503:setI", "SR-PS-QS4-1504:setI", "SR-PS-QS5-1505:setI", "SR-PS-QS5-1506:setI", "SR-PS-QS4-1507:setI", "SR-PS-QS3-1508:setI", "SR-PS-QS2-1509:setI", "SR-PS-QS1-1510:setI", "SR-PS-QS1-1601:setI", "SR-PS-QS2-1602:setI", "SR-PS-QS3-1603:setI", "SR-PS-QS4-1604:setI", "SR-PS-QS5-1605:setI", "SR-PS-QS5-1606:setI", "SR-PS-QS4-1607:setI", "SR-PS-QL3-1608:setI", "SR-PS-QL2-1609:setI", "SR-PS-QL1-1610:setI", "SR-PS-QL1-1701:setI", "SR-PS-QL2-1702:setI", "SR-PS-QL3-1703:setI", "SR-PS-QS4-1704:setI", "SR-PS-QS5-1705:setI", "SR-PS-QS5-1706:setI", "SR-PS-QS4-1707:setI", "SR-PS-QS3-1708:setI", "SR-PS-QS2-1709:setI", "SR-PS-QS1-1710:setI", "SR-PS-QS1-1801:setI", "SR-PS-QS2-1802:setI", "SR-PS-QS3-1803:setI", "SR-PS-QS4-1804:setI", "SR-PS-QS5-1805:setI", "SR-PS-QS5-1806:setI", "SR-PS-QS4-1807:setI", "SR-PS-QS3-1808:setI", "SR-PS-QS2-1809:setI", "SR-PS-QS1-1810:setI", "SR-PS-QS1-1901:setI", "SR-PS-QS2-1902:setI", "SR-PS-QS3-1903:setI", "SR-PS-QS4-1904:setI", "SR-PS-QS5-1905:setI", "SR-PS-QS5-1906:setI", "SR-PS-QS4-1907:setI", "SR-PS-QS3-1908:setI", "SR-PS-QS2-1909:setI", "SR-PS-QS1-1910:setI", "SR-PS-QS1-2001:setI", "SR-PS-QS2-2002:setI", "SR-PS-QS3-2003:setI", "SR-PS-QS4-2004:setI", "SR-PS-QS5-2005:setI", "SR-PS-QS5-2006:setI", "SR-PS-QS4-2007:setI", "SR-PS-QL3-2008:setI", "SR-PS-QL2-2009:setI", "SR-PS-QL1-2010:setI", "SR-PS-QL1-2101:setI", "SR-PS-QL2-2102:setI", "SR-PS-QL3-2103:setI", "SR-PS-QS4-2104:setI", "SR-PS-QS5-2105:setI", "SR-PS-QS5-2106:setI", "SR-PS-QS4-2107:setI", "SR-PS-QS3-2108:setI", "SR-PS-QS2-2109:setI", "SR-PS-QS1-2110:setI", "SR-PS-QS1-2201:setI", "SR-PS-QS2-2202:setI", "SR-PS-QS3-2203:setI", "SR-PS-QS4-2204:setI", "SR-PS-QS5-2205:setI", "SR-PS-QS5-2206:setI", "SR-PS-QS4-2207:setI", "SR-PS-QS3-2208:setI", "SR-PS-QS2-2209:setI", "SR-PS-QS1-2210:setI", "SR-PS-QS1-2301:setI", "SR-PS-QS2-2302:setI", "SR-PS-QS3-2303:setI", "SR-PS-QS4-2304:setI", "SR-PS-QS5-2305:setI", "SR-PS-QS5-2306:setI", "SR-PS-QS4-2307:setI", "SR-PS-QS3-2308:setI", "SR-PS-QS2-2309:setI", "SR-PS-QS1-2310:setI", "SR-PS-QS1-2401:setI", "SR-PS-QS2-2402:setI", "SR-PS-QS3-2403:setI", "SR-PS-QS4-2404:setI", "SR-PS-QS5-2405:setI", "SR-PS-QS5-2406:setI", "SR-PS-QS4-2407:setI", "SR-PS-QL3-2408:setI", "SR-PS-QL2-2409:setI", "SR-PS-QL1-2410:setI", "SR-PS-S1-011:setI", "SR-PS-S2-012:setI", "SR-PS-SD-013:setI", "SR-PS-SF-014:setI", "SR-PS-SD-015:setI", "SR-PS-S4-016:setI", "SR-PS-S3-017:setI", "SR-PS-S5-021:setI", "SR-PS-S6-022:setI", "SR-PS-SD-023:setI", "SR-PS-SF-024:setI", "SR-PS-SD-025:setI", "SR-PS-S6-026:setI", "SR-PS-S5-027:setI", "SR-PS-S5-031:setI", "SR-PS-S6-032:setI", "SR-PS-SD-033:setI", "SR-PS-SF-034:setI", "SR-PS-SD-035:setI", "SR-PS-S6-036:setI", "SR-PS-S5-037:setI", "SR-PS-S3-041:setI", "SR-PS-S4-042:setI", "SR-PS-SD-043:setI", "SR-PS-SF-044:setI", "SR-PS-SD-045:setI", "SR-PS-S2-046:setI", "SR-PS-S1-047:setI", "SR-PS-S1-051:setI", "SR-PS-S2-052:setI", "SR-PS-SD-053:setI", "SR-PS-SF-054:setI", "SR-PS-SD-055:setI", "SR-PS-S4-056:setI", "SR-PS-S3-057:setI", "SR-PS-S5-061:setI", "SR-PS-S6-062:setI", "SR-PS-SD-063:setI", "SR-PS-SF-064:setI", "SR-PS-SD-065:setI", "SR-PS-S6-066:setI", "SR-PS-S5-067:setI", "SR-PS-S5-071:setI", "SR-PS-S6-072:setI", "SR-PS-SD-073:setI", "SR-PS-SF-074:setI", "SR-PS-SD-075:setI", "SR-PS-S6-076:setI", "SR-PS-S5-077:setI", "SR-PS-S3-081:setI", "SR-PS-S4-082:setI", "SR-PS-SD-083:setI", "SR-PS-SF-084:setI", "SR-PS-SD-085:setI", "SR-PS-S2-086:setI", "SR-PS-S1-087:setI", "SR-PS-S1-091:setI", "SR-PS-S2-092:setI", "SR-PS-SD-093:setI", "SR-PS-SF-094:setI", "SR-PS-SD-095:setI", "SR-PS-S4-096:setI", "SR-PS-S3-097:setI", "SR-PS-S5-101:setI", "SR-PS-S6-102:setI", "SR-PS-SD-103:setI", "SR-PS-SF-104:setI", "SR-PS-SD-105:setI", "SR-PS-S6-106:setI", "SR-PS-S5-107:setI", "SR-PS-S5-111:setI", "SR-PS-S6-112:setI", "SR-PS-SD-113:setI", "SR-PS-SF-114:setI", "SR-PS-SD-115:setI", "SR-PS-S6-116:setI", "SR-PS-S5-117:setI", "SR-PS-S3-121:setI", "SR-PS-S4-122:setI", "SR-PS-SD-123:setI", "SR-PS-SF-124:setI", "SR-PS-SD-125:setI", "SR-PS-S2-126:setI", "SR-PS-S1-127:setI", "SR-PS-S1-131:setI", "SR-PS-S2-132:setI", "SR-PS-SD-133:setI", "SR-PS-SF-134:setI", "SR-PS-SD-135:setI", "SR-PS-S4-136:setI", "SR-PS-S3-137:setI", "SR-PS-S5-141:setI", "SR-PS-S6-142:setI", "SR-PS-SD-143:setI", "SR-PS-SF-144:setI", "SR-PS-SD-145:setI", "SR-PS-S6-146:setI", "SR-PS-S5-147:setI", "SR-PS-S5-151:setI", "SR-PS-S6-152:setI", "SR-PS-SD-153:setI", "SR-PS-SF-154:setI", "SR-PS-SD-155:setI", "SR-PS-S6-156:setI", "SR-PS-S5-157:setI", "SR-PS-S3-161:setI", "SR-PS-S4-162:setI", "SR-PS-SD-163:setI", "SR-PS-SF-164:setI", "SR-PS-SD-165:setI", "SR-PS-S2-166:setI", "SR-PS-S1-167:setI", "SR-PS-S1-171:setI", "SR-PS-S2-172:setI", "SR-PS-SD-173:setI", "SR-PS-SF-174:setI", "SR-PS-SD-175:setI", "SR-PS-S4-176:setI", "SR-PS-S3-177:setI", "SR-PS-S5-181:setI", "SR-PS-S6-182:setI", "SR-PS-SD-183:setI", "SR-PS-SF-184:setI", "SR-PS-SD-185:setI", "SR-PS-S6-186:setI", "SR-PS-S5-187:setI", "SR-PS-S5-191:setI", "SR-PS-S6-192:setI", "SR-PS-SD-193:setI", "SR-PS-SF-194:setI", "SR-PS-SD-195:setI", "SR-PS-S6-196:setI", "SR-PS-S5-197:setI", "SR-PS-S3-201:setI", "SR-PS-S4-202:setI", "SR-PS-SD-203:setI", "SR-PS-SF-204:setI", "SR-PS-SD-205:setI", "SR-PS-S2-206:setI", "SR-PS-S1-207:setI", "SR-PS-S1-211:setI", "SR-PS-S2-212:setI", "SR-PS-SD-213:setI", "SR-PS-SF-214:setI", "SR-PS-SD-215:setI", "SR-PS-S4-216:setI", "SR-PS-S3-217:setI", "SR-PS-S5-221:setI", "SR-PS-S6-222:setI", "SR-PS-SD-223:setI", "SR-PS-SF-224:setI", "SR-PS-SD-225:setI", "SR-PS-S6-226:setI", "SR-PS-S5-227:setI", "SR-PS-S5-231:setI", "SR-PS-S6-232:setI", "SR-PS-SD-233:setI", "SR-PS-SF-234:setI", "SR-PS-SD-235:setI", "SR-PS-S6-236:setI", "SR-PS-S5-237:setI", "SR-PS-S3-241:setI", "SR-PS-S4-242:setI", "SR-PS-SD-243:setI", "SR-PS-SF-244:setI", "SR-PS-SD-245:setI", "SR-PS-S2-246:setI", "SR-PS-S1-247:setI", "SR-PS-SKEW-011:setI", "SR-PS-SKEW-012:setI", "SR-PS-SKEW-013:setI", "SR-PS-SKEW-014:setI", "SR-PS-SKEW-015:setI", "SR-PS-SKEW-016:setI", "SR-PS-SKEW-017:setI", "SR-PS-SKEW-021:setI", "SR-PS-SKEW-022:setI", "SR-PS-SKEW-023:setI", "SR-PS-SKEW-024:setI", "SR-PS-SKEW-025:setI", "SR-PS-SKEW-026:setI", "SR-PS-SKEW-027:setI", "SR-PS-SKEW-031:setI", "SR-PS-SKEW-032:setI", "SR-PS-SKEW-033:setI", "SR-PS-SKEW-034:setI", "SR-PS-SKEW-035:setI", "SR-PS-SKEW-036:setI", "SR-PS-SKEW-037:setI", "SR-PS-SKEW-041:setI", "SR-PS-SKEW-042:setI", "SR-PS-SKEW-043:setI", "SR-PS-SKEW-044:setI", "SR-PS-SKEW-045:setI", "SR-PS-SKEW-046:setI", "SR-PS-SKEW-047:setI", "SR-PS-SKEW-051:setI", "SR-PS-SKEW-052:setI", "SR-PS-SKEW-053:setI", "SR-PS-SKEW-054:setI", "SR-PS-SKEW-055:setI", "SR-PS-SKEW-056:setI", "SR-PS-SKEW-057:setI", "SR-PS-SKEW-061:setI", "SR-PS-SKEW-062:setI", "SR-PS-SKEW-063:setI", "SR-PS-SKEW-064:setI", "SR-PS-SKEW-065:setI", "SR-PS-SKEW-066:setI", "SR-PS-SKEW-067:setI", "SR-PS-SKEW-071:setI", "SR-PS-SKEW-072:setI", "SR-PS-SKEW-073:setI", "SR-PS-SKEW-074:setI", "SR-PS-SKEW-075:setI", "SR-PS-SKEW-076:setI", "SR-PS-SKEW-077:setI", "SR-PS-SKEW-081:setI", "SR-PS-SKEW-082:setI", "SR-PS-SKEW-083:setI", "SR-PS-SKEW-084:setI", "SR-PS-SKEW-085:setI", "SR-PS-SKEW-086:setI", "SR-PS-SKEW-087:setI", "SR-PS-SKEW-091:setI", "SR-PS-SKEW-092:setI", "SR-PS-SKEW-093:setI", "SR-PS-SKEW-094:setI", "SR-PS-SKEW-095:setI", "SR-PS-SKEW-096:setI", "SR-PS-SKEW-097:setI", "SR-PS-SKEW-101:setI", "SR-PS-SKEW-102:setI", "SR-PS-SKEW-103:setI", "SR-PS-SKEW-104:setI", "SR-PS-SKEW-105:setI", "SR-PS-SKEW-106:setI", "SR-PS-SKEW-107:setI", "SR-PS-SKEW-111:setI", "SR-PS-SKEW-112:setI", "SR-PS-SKEW-113:setI", "SR-PS-SKEW-114:setI", "SR-PS-SKEW-115:setI", "SR-PS-SKEW-116:setI", "SR-PS-SKEW-117:setI", "SR-PS-SKEW-121:setI", "SR-PS-SKEW-122:setI", "SR-PS-SKEW-123:setI", "SR-PS-SKEW-124:setI", "SR-PS-SKEW-125:setI", "SR-PS-SKEW-126:setI", "SR-PS-SKEW-127:setI", "SR-PS-SKEW-131:setI", "SR-PS-SKEW-132:setI", "SR-PS-SKEW-133:setI", "SR-PS-SKEW-134:setI", "SR-PS-SKEW-135:setI", "SR-PS-SKEW-136:setI", "SR-PS-SKEW-137:setI", "SR-PS-SKEW-141:setI", "SR-PS-SKEW-142:setI", "SR-PS-SKEW-143:setI", "SR-PS-SKEW-144:setI", "SR-PS-SKEW-145:setI", "SR-PS-SKEW-146:setI", "SR-PS-SKEW-147:setI", "SR-PS-SKEW-151:setI", "SR-PS-SKEW-152:setI", "SR-PS-SKEW-153:setI", "SR-PS-SKEW-154:setI", "SR-PS-SKEW-155:setI", "SR-PS-SKEW-156:setI", "SR-PS-SKEW-157:setI", "SR-PS-SKEW-161:setI", "SR-PS-SKEW-162:setI", "SR-PS-SKEW-163:setI", "SR-PS-SKEW-164:setI", "SR-PS-SKEW-165:setI", "SR-PS-SKEW-166:setI", "SR-PS-SKEW-167:setI", "SR-PS-SKEW-171:setI", "SR-PS-SKEW-172:setI", "SR-PS-SKEW-173:setI", "SR-PS-SKEW-174:setI", "SR-PS-SKEW-175:setI", "SR-PS-SKEW-176:setI", "SR-PS-SKEW-177:setI", "SR-PS-SKEW-181:setI", "SR-PS-SKEW-182:setI", "SR-PS-SKEW-183:setI", "SR-PS-SKEW-184:setI", "SR-PS-SKEW-185:setI", "SR-PS-SKEW-186:setI", "SR-PS-SKEW-187:setI", "SR-PS-SKEW-191:setI", "SR-PS-SKEW-192:setI", "SR-PS-SKEW-193:setI", "SR-PS-SKEW-194:setI", "SR-PS-SKEW-195:setI", "SR-PS-SKEW-196:setI", "SR-PS-SKEW-197:setI", "SR-PS-SKEW-201:setI", "SR-PS-SKEW-202:setI", "SR-PS-SKEW-203:setI", "SR-PS-SKEW-204:setI", "SR-PS-SKEW-205:setI", "SR-PS-SKEW-206:setI", "SR-PS-SKEW-207:setI", "SR-PS-SKEW-211:setI", "SR-PS-SKEW-212:setI", "SR-PS-SKEW-213:setI", "SR-PS-SKEW-214:setI", "SR-PS-SKEW-215:setI", "SR-PS-SKEW-216:setI", "SR-PS-SKEW-217:setI", "SR-PS-SKEW-221:setI", "SR-PS-SKEW-222:setI", "SR-PS-SKEW-223:setI", "SR-PS-SKEW-224:setI", "SR-PS-SKEW-225:setI", "SR-PS-SKEW-226:setI", "SR-PS-SKEW-227:setI", "SR-PS-SKEW-231:setI", "SR-PS-SKEW-232:setI", "SR-PS-SKEW-233:setI", "SR-PS-SKEW-234:setI", "SR-PS-SKEW-235:setI", "SR-PS-SKEW-236:setI", "SR-PS-SKEW-237:setI", "SR-PS-SKEW-241:setI", "SR-PS-SKEW-242:setI", "SR-PS-SKEW-243:setI", "SR-PS-SKEW-244:setI", "SR-PS-SKEW-245:setI", "SR-PS-SKEW-246:setI", "SR-PS-SKEW-247:setI", "SR-RF2-LLRF:setGapVoltage", "SR-RF2-LLRF:setStationPhase", "SR-RF3-LLRF:setGapVoltage", "SR-RF3-LLRF:setStationPhase", "SR-PS-DMB09-Q1:setI", "SR-PS-DMB09-Q2:setI", "SR-PS-DMB09-Q3:setI", "SR-PS-DMB25-Q1:setI", "SR-PS-DMB25-Q2:setI", "SR-PS-DMB25-Q3:setI", "SR-PS-DMB41-Q1:setI", "SR-PS-DMB41-Q2:setI", "SR-PS-DMB41-Q3:setI", "SR-PS-DMB09-HC1:setI", "SR-PS-DMB09-HC2:setI", "SR-PS-DMB09-VC1:setI", "SR-PS-DMB09-VC2:setI", "SR-PS-DMB25-HC1:setI", "SR-PS-DMB25-HC2:setI", "SR-PS-DMB25-VC1:setI", "SR-PS-DMB25-VC2:setI", "SR-PS-DMB41-HC1:setI", "SR-PS-DMB41-HC2:setI", "SR-PS-DMB41-VC1:setI", "SR-PS-DMB41-VC2:setI"]  # PV nanes(SR)
  w13 = string[] ["LTB-PS-HC-1:setI", "LTB-PS-HC-2:setI", "LTB-PS-HC-3:setI", "LTB-PS-HC-4:setI", "LTB-PS-HC-5:setI", "LTB-PS-VC-1:setI", "LTB-PS-VC-2:setI", "LTB-PS-VC-3:setI", "LTB-PS-VC-4:setI", "LTB-PS-VC-5:setI", "LTB-PS-VC-6:setI", "LTB-PS-VC-7:setI", "LTB-PS-Q1A:setI", "LTB-PS-Q1B:setI", "LTB-PS-Q1C:setI", "LTB-PS-Q2A:setI", "LTB-PS-Q2B:setI", "LTB-PS-Q2C:setI", "LTB-PS-Q3A:setI", "LTB-PS-Q3B:setI", "LTB-PS-Q4A:setI", "LTB-PS-Q4B:setI", "LTB-PS-QQ:setI", "LTB-PS-BEND-1:setI", "LTB-PS-VC-2a:setI", "LTB-PS-HC-3a:setI", "LTB-PS-HC-3b:setI", "LTB-PS-HC-4a:setI", "LTB-PS-HC-5a:setI", "LI-DI-SLIT-motor:axis2Position1", "LI-DI-SLIT-motor:axis1Position1"]  # PV nanes(LTB)
  w15 = string[] ["BTS-PS-HC-1:setI", "BTS-PS-HC-2:setI", "BTS-PS-HC-3:setI", "BTS-PS-HC-4:setI", "BTS-PS-HC-5:setI", "BTS-PS-VC-2:setI", "BTS-PS-VC-3:setI", "BTS-PS-VC-4:setI", "BTS-PS-VC-5:setI", "BTS-PS-VC-6:setI", "BTS-PS-Q1A:setI", "BTS-PS-Q1B:setI", "BTS-PS-Q1C:setI", "BTS-PS-Q2A:setI", "BTS-PS-Q2B:setI", "BTS-PS-Q2C:setI", "BTS-PS-Q3A:setI", "BTS-PS-BEND-1:setI", "BTS-PS-BEND-2:setI", "BR-PS-EXT-K1:setHV", "BR-PS-EXT-K2:setHV", "SR-PS-INJ-SE1:setHV", "SR-PS-INJ-SE2:setHV", "SR-PS-INJ-K1:setHV", "SR-PS-INJ-K2:setHV", "SR-PS-INJ-K3:setHV", "SR-PS-INJ-K4:setHV", "CPCIPM-TI-EVR:Pulse4DelaySet", "CPCIPM-TI-EVR:Pulse5DelaySet", "CPCIPM-TI-EVR:Pulse3DelaySet", "CPCIPM-TI-EVR:Pulse6DelaySet", "CPCIPM-TI-EVR:Pulse7DelaySet", "T560:setADelay", "T560:setBDelay", "T560:setCDelay", "T560:setDDelay", "CPCIPM-TI-EVR:Pulse4DelaySet", "CPCIPM-TI-EVR:Pulse5DelaySet", "BR-PS-EXT-SE1:setHV", "BR-PS-EXT-SE2:setHV", "CPCIPM-TI-EVR:Pulse3DelaySet", "CPCIPM-TI-EVR:Pulse11DelaySet"]  # PV nanes(BTS)
  w14 = string[] ["BR-PS-HC-101:setI", "BR-PS-HC-102:setI", "BR-PS-HC-103:setI", "BR-PS-HC-104:setI", "BR-PS-HC-105:setI", "BR-PS-HC-106:setI", "BR-PS-HC-107:setI", "BR-PS-HC-108:setI", "BR-PS-HC-109:setI", "BR-PS-HC-110:setI", "BR-PS-HC-201:setI", "BR-PS-HC-202:setI", "BR-PS-HC-203:setI", "BR-PS-HC-204:setI", "BR-PS-HC-205:setI", "BR-PS-HC-206:setI", "BR-PS-HC-207:setI", "BR-PS-HC-208:setI", "BR-PS-HC-209:setI", "BR-PS-HC-210:setI", "BR-PS-HC-301:setI", "BR-PS-HC-302:setI", "BR-PS-HC-303:setI", "BR-PS-HC-304:setI", "BR-PS-HC-305:setI", "BR-PS-HC-306:setI", "BR-PS-HC-307:setI", "BR-PS-HC-308:setI", "BR-PS-HC-309:setI", "BR-PS-HC-310:setI", "BR-PS-HC-401:setI", "BR-PS-HC-402:setI", "BR-PS-HC-403:setI", "BR-PS-HC-404:setI", "BR-PS-HC-405:setI", "BR-PS-HC-406:setI", "BR-PS-HC-407:setI", "BR-PS-HC-408:setI", "BR-PS-HC-409:setI", "BR-PS-HC-410:setI", "BR-PS-HC-501:setI", "BR-PS-HC-502:setI", "BR-PS-HC-503:setI", "BR-PS-HC-504:setI", "BR-PS-HC-505:setI", "BR-PS-HC-506:setI", "BR-PS-HC-507:setI", "BR-PS-HC-508:setI", "BR-PS-HC-509:setI", "BR-PS-HC-510:setI", "BR-PS-HC-601:setI", "BR-PS-HC-602:setI", "BR-PS-HC-603:setI", "BR-PS-HC-603a:setI", "BR-PS-HC-604:setI", "BR-PS-HC-605:setI", "BR-PS-HC-606:setI", "BR-PS-HC-606a:setI", "BR-PS-HC-607:setI", "BR-PS-HC-608:setI", "BR-PS-HC-609:setI", "BR-PS-HC-610:setI", "BR-PS-VC-101:setI", "BR-PS-VC-102:setI", "BR-PS-VC-103:setI", "BR-PS-VC-104:setI", "BR-PS-VC-105:setI", "BR-PS-VC-106:setI", "BR-PS-VC-201:setI", "BR-PS-VC-202:setI", "BR-PS-VC-203:setI", "BR-PS-VC-204:setI", "BR-PS-VC-205:setI", "BR-PS-VC-206:setI", "BR-PS-VC-301:setI", "BR-PS-VC-302:setI", "BR-PS-VC-303:setI", "BR-PS-VC-304:setI", "BR-PS-VC-305:setI", "BR-PS-VC-306:setI", "BR-PS-VC-401:setI", "BR-PS-VC-402:setI", "BR-PS-VC-403:setI", "BR-PS-VC-404:setI", "BR-PS-VC-405:setI", "BR-PS-VC-406:setI", "BR-PS-VC-501:setI", "BR-PS-VC-502:setI", "BR-PS-VC-503:setI", "BR-PS-VC-504:setI", "BR-PS-VC-505:setI", "BR-PS-VC-506:setI", "BR-PS-VC-601:setI", "BR-PS-VC-602:setI", "BR-PS-VC-602a:setI", "BR-PS-VC-603:setI", "BR-PS-VC-604:setI", "BR-PS-VC-604a:setI", "BR-PS-VC-605:setI", "BR-PS-VC-606:setI", "BR-PS-VC-100a:setI", "BR-PS-SD:setI", "BR-PS-SF:setI", "cpsc_027:AO:SLOW_SET:CH:1", "cpsc_037:AO:SLOW_SET:CH:3", "BR-RF-LLRF:setStationPhase", "TI-INJ-PROC:setTinj", "BR-PS-INJ-SE:setHV", "CPCIPM-TI-EVR:Pulse1DelaySet", "BR-PS-INJ-KI:setHV", "CPCIPM-TI-EVR:Pulse2DelaySet", "BR-PS-QF:setWfDC", "BR-PS-QM:setWfDC", "BR-PS-Q1:setWfDC", "BR-PS-Q2:setWfDC", "BR-PS-BEND:setWfDC"]  # PV nanes (BR_without_Wf)
  w19 = FALSE ("Trip Evt B")
  (unwired) string[] ["FE-DI-XBPM-051:SA:SA_X_MONITOR", "FE-DI-XBPM-051:SA:SA_Y_MONITOR", "FE-DI-XBPM-091:SA:SA_X_MONITOR", "FE-DI-XBPM-091:SA:SA_Y_MONITOR", "FE-DI-XBPM-211:SA:SA_X_MONITOR", "FE-DI-XBPM-211:SA:SA_Y_MONITOR", "FE-DI-XBPM-231:SA:SA_X_MONITOR", "FE-DI-XBPM-231:SA:SA_Y_MONITOR", "FE-DI-XBPM-251:SA:SA_X_MONITOR", "FE-DI-XBPM-251:SA:SA_Y_MONITOR", "FE-DI-XBPM-411:SA:SA_X_MONITOR", "FE-DI-XBPM-411:SA:SA_Y_MONITOR", "FE-DI-XBPM-451:SA:SA_X_MONITOR", "FE-DI-XBPM-451:SA:SA_Y_MONITOR"]
  (unwired) string[] ["LI-VA-VAL-01:STA:POS", "LI-VA-VAL-02:STA:POS", "LI-VA-VAL-03:STA:POS", "LI-VA-VAL-04:STA:POS", "LI-VA-VAL-05:STA:POS"]
  (unwired) string[] ["SR-DI-SOFB-H:getStatus", "SR-DI-SOFB-V:getStatus", "IGPF:TPSX:FBCTRL", "IGPF:TPSY:FBCTRL", "SR-DI-FOFB-H:getStatus", "SR-DI-FOFB-V:getStatus"]
  # "V1.4.5 \n修改shift register 儲存筆數上限(之前沒有)，改成5000\n增加fill pattern的gap值\n檢查處加入ID 的mode"
  # "這3個變動太頻繁，不紀錄"
  # "PV nanes(ID gap_phase_Taper_)"
  # "PV nanes(Feedback_ILK)"
  # "V1.4.2 改成直接用最大最小值當作scale的最大最小值"
  # "1.4.1\n將BeamCurrent 圖形的Y軸上下限\n改成取最大值的1.01倍，再無條件進位取整數\n最小值的0.99倍，再無條件捨去取整數"
  # "FE-DI-XBPM-051:SA:SA_Y_MONITOR"
  # "FE-DI-XBPM-051:SA:SA_X_MONITOR"
  # "TPS-SR-052:bpm4:ilk:enabled"
  # "0 為OPEN"
  # "VALVE(EPICS)"
  n1 = local read "last ? Hrs"() -> (w29:dbl)
  n2 = Multiply(x=3600.0 ("y"), y=w29) -> (x*y=w53:dbl)
  n3 = Get Date/Time In Seconds() -> (seconds since 1Jan1904=w24:timestamp)
  n4 = Subtract(x=w24, y=w53) -> (x-y=w23:timestamp)
  n5 = call "TimeToString.vi"("Time Stamp Control"=w24) -> ("result string"=w55:string)
  n6 = call "TimeToString.vi"("Time Stamp Control"=w23) -> ("result string"=w54:string)
  n7 = call <vilib>:"Application Directory.vi"() -> ("Application Directory"=w56:path)
  n8 = Build Path(base path=w56, name or relative path="DSN\\172-18-0-32.dsn") -> (appended path=w58:path)
  n9 = call-poly <vilib>:"DB Tools Open Connection.vi"("connection information"=w58) -> ("error out"=w47:errorcluster, "connection reference"=w46:T2)  [unwired: 7 in]
  n10 = Concatenate Strings("SELECT  float_val , smpl_time\nFROM sample \nwhere  channel_id = 104 and smpl_time between '" ("result string"), w54, "' ::timestamp and '" ("result string"), w55, "' ::timestamp" ("result string")) -> (w31:string)
  n11 = call-poly <vilib>:"DB Tools Execute Query.vi"("error in (no error)"=w47, "SQL query"=w31, "connection reference"=w46) -> ("error out"=w44:errorcluster, "recordset reference"=w45:T3)  [unwired: 5 in]
  n12 = call-poly <vilib>:"DB Tools Fetch Recordset Data.vi"("error in (no error)"=w44, "recordset reference"=w45) -> ("error out"=w42:errorcluster, "recordset data"=w39:variant[][], "recordset reference out"=w43:T3)  [unwired: 3 in]
  n13 = call-poly <vilib>:"DB Tools Free Object.vi"("error in (no error)"=w42, "recordset reference"=w43) -> ("error out"=w40:errorcluster, "connection reference"=w41:T2)  [unwired: 8 in]
  n14 = Variant To Data(type=string[][] [], Variant=w39) -> (data=w37:string[][])  [unwired: 1 in, 1 out]
  n15 = call <vilib>:"DB Tools Close Connection.vi"("error in (no error)"=w40, "connection reference"=w41) -> ()  [unwired: 5 in, 1 out]
  n16 = Transpose 2D Array(2D array=w37) -> (transposed array=w35:string[][])
  n17 = Index Array(array=w35, index (row) #1=0 ("index (row)"), index (row) #2=1 ("index (row)")) -> (element #1=w49:string[], element #2=w51:string[])  [unwired: 2 in]
  n18 = Fract/Exp String To Number(string=w49) -> (number=w25:dbl[])  [unwired: 3 in, 1 out]
  n19 = Array Max & Min(array=w25) -> (max value=w21:dbl, min value=w20:dbl)  [unwired: 2 out]
  n20 = for {
    tunnel: w51 -> [w62] mode=indexing
    tunnel: [w61] -> w50 mode=indexing
    n21 = Scan From String "Scan From String"(format string="%<%Y/%m/%d %p %I:%M:%S>T", input string=w62, initial scan location=u32 0, default 1=timestamp(-73814400 s since 1904-01-01)) -> (output 1=w65:timestamp)  [unwired: 1 in, 3 out]
    n22 = To Double Precision Float(number=w65) -> (double precision float=w61:dbl)
  }
  n23 = To Double Precision Float(number=w24) -> (double precision float=w27:dbl)
  n24 = To Double Precision Float(number=w23) -> (double precision float=w26:dbl)
  n25 = control-ref of="BeamCurrent History"() -> (w28:refnum<vi>)
  n26 = property on="Property Node" class="XYGraph (strict)"(reference=w28, "XScale.Maximum"=w27, "XScale.Minimum"=w26, "YScale.Maximum"=w21, "YScale.Minimum"=w20) -> ()  [unwired: 1 in, 2 out]
  n27 = local write "Refresh B"(w19) -> ()
  n28 = local write "Trip Evt B"(w19) -> ()
  n29 = Bundle(w50, w25) -> (w30:cluster{dbl[], dbl[]})  [unwired: 1 in]
  n30 = property on="result" class="Str"("Visible"=FALSE) -> ()  [unwired: 2 in, 2 out]
  n31 = Build Array (concatenate)(w6, string[] ["SR-ID-IU22-05:gapMotorOff", "SR-ID-IU22A-09:gapMotorOff", "SR-ID-IU22B-09:gapMotorOff", "SR-ID-IUT22-21:gapMotorOff", "SR-ID-IU22-23:gapMotorOff", "SR-ID-IU22A-25:gapMotorOff", "SR-ID-IU22B-25:gapMotorOff", "SR-ID-EPU48A-41:gapMotorOff", "SR-ID-EPU48B-41:gapMotorOff", "SR-ID-EPU46-45:gapMotorOff", "SR-ID-EPU48A-41:phaseMotorOff", "SR-ID-EPU48B-41:phaseMotorOff", "SR-ID-EPU46-45:phaseMotorOff"], w1) -> (w5:string[])
  n32 = Build Array (concatenate)(w2, w13, w14, w15, w16, w5, string[] ["SR-DI-FOFB-H:setStatus", "SR-DI-FOFB-V:setStatus", "IGPF:TPSX:FBCTRL", "IGPF:TPSY:FBCTRL", "TPS-SR-022:bpm3:ilk:enabled", "SR-DI-ANGLE-ILK:StatusX", "SR-DI-ANGLE-ILK:StatusY", "SR-DI-RF-FB:setStatus", "SR-ID-EPU48-TFF:status", "SR-ID-EPU48-CFF:status", "SR-ID-EPU46-TFF:status", "SR-ID-EPU46-CFF:status"], w17, w4, w3) -> (w18:string[])
  "PV list" <- w18
  n33 = Get Date/Time In Seconds() -> (seconds since 1Jan1904=w10:timestamp)
  n34 = To Double Precision Float(number=w10) -> (double precision float=w8:dbl)
  "Program Start Time" <- w8
  n35 = while {
    shift-right: [w217] -> _
    shift-left: _ -> [w215]
    shift-right: [w216] -> _
    shift-left: _ -> [w214]
    shift-right: [w83] -> _
    shift-left: w30 -> [w82]
    tunnel: w8 -> [w78]
    stop <- "stop" stop-if-true
    (unwired) string[] ["Event Time      ", "PV_name        ", "Ori_Value", "New_Value "] ("diff_Value")
    w77 = dbl[] [1.0, 1.1666666666666667, 1.3333333333333333, 1.5, 1.6666666666666665, 1.8333333333333333, 2.0, 2.142857142857143, 2.2857142857142856, 2.4285714285714284, 2.571428571428571, 2.7142857142857144, 2.857142857142857, 3.0, 3.142857142857143, 3.2857142857142856, 3.4285714285714284, 3.571428571428571, 3.7142857142857144, 3.857142857142857, 4.0, 4.125, 4.25, 4.375, 4.5, 4.625, 4.75, 4.875, 5.0, 5.125, 5.25, 5.375, 5.5, 5.625, 5.75, 5.875, 6.0, 6.142857142857143, 6.285714285714286, 6.428571428571429, 6.571428571428571, 6.714285714285714, 6.857142857142857, 7.0, 7.142857142857143, 7.285714285714286, 7.428571428571429, 7.571428571428571, 7.714285714285714, 7.857142857142857, 8.0, 8.142857142857142, 8.285714285714286, 8.428571428571429, 8.571428571428571, 8.714285714285714, 8.857142857142858, 9.0, 9.142857142857142, 9.285714285714286, 9.428571428571429, 9.571428571428571, 9.714285714285714, 9.857142857142858, 10.0, 10.142857142857142, 10.285714285714286, 10.428571428571429, 10.571428571428571, 10.714285714285714, 10.857142857142858, 11.0, 11.142857142857142, 11.285714285714286, 11.428571428571429, 11.571428571428571, 11.714285714285714, 11.857142857142858, 12.0, 12.125, 12.25, 12.375, 12.5, 12.625, 12.75, 12.875, 13.0, 13.125, 13.25, 13.375, 13.5, 13.625, 13.75, 13.875, 14.0, 14.142857142857142, 14.285714285714286, 14.428571428571429, 14.571428571428571, 14.714285714285714, 14.857142857142858, 15.0, 15.142857142857142, 15.285714285714286, 15.428571428571429, 15.571428571428571, 15.714285714285714, 15.857142857142858, 16.0, 16.142857142857142, 16.285714285714285, 16.428571428571427, 16.571428571428573, 16.714285714285715, 16.857142857142858, 17.0, 17.142857142857142, 17.285714285714285, 17.428571428571427, 17.571428571428573, 17.714285714285715, 17.857142857142858, 18.0, 18.142857142857142, 18.285714285714285, 18.428571428571427, 18.571428571428573, 18.714285714285715, 18.857142857142858, 19.0, 19.142857142857142, 19.285714285714285, 19.428571428571427, 19.571428571428573, 19.714285714285715, 19.857142857142858, 20.0, 20.125, 20.25, 20.375, 20.5, 20.625, 20.75, 20.875, 21.0, 21.125, 21.25, 21.375, 21.5, 21.625, 21.75, 21.875, 22.0, 22.142857142857142, 22.285714285714285, 22.428571428571427, 22.571428571428573, 22.714285714285715, 22.857142857142858, 23.0, 23.142857142857142, 23.285714285714285, 23.428571428571427, 23.571428571428573, 23.714285714285715, 23.857142857142858, 24.0, 24.166666666666668, 24.333333333333332, 24.5, 24.666666666666668, 24.833333333333332]  # Array of X axis  平均分配至各段
    w108 = string[] ["SR-ID-IU22-05:setECMode", "SR-ID-IU22A-09:setECMode", "SR-ID-IU22B-09:setECMode", "SR-ID-IUT22-21:setECMode", "SR-ID-IU22-23:setECMode", "SR-ID-IU22A-25:setECMode", "SR-ID-IU22B-25:setECMode", "SR-ID-EPU48A-41:setECMode", "SR-ID-EPU48B-41:setECMode", "SR-ID-EPU46-45:setECMode"]  # ID_mode
    w194 = string[] ["FE-05-PAB:Open", "FE-05-MGV:Open", "FE-05-FCV:Open", "FE-09-PAB:Open", "FE-09-MGV:Open", "FE-09-FCV:Open", "FE-21-PAB:Open", "FE-21-MGV:Open", "FE-21-FCV:Open", "FE-23-PAB:Open", "FE-23-PAB:Open", "FE-23-FCV:Open", "FE-25-PAB:Open", "FE-25-MGV:Open", "FE-25-FCV:Open", "FE-41-PAB:Open", "FE-41-MGV:Open", "FE-41-FCV:Open", "FE-45-PAB:Open", "FE-45-MGV:Open", "FE-45-FCV:Open"]  # PAB_MGV_FCV enable
    (unwired) "LI-DI-WCM:getWfCh1"
    (unwired) "SR-DI-FP:CurrentBuffer"
    w332 = 0.001
    w330 = string[] ["SR-DI-BPM-011:Y", "SR-DI-BPM-012:Y", "SR-DI-BPM-013:Y", "SR-DI-BPM-014:Y", "SR-DI-BPM-015:Y", "SR-DI-BPM-016:Y", "SR-DI-BPM-017:Y", "SR-DI-BPM-021:Y", "SR-DI-BPM-022:Y", "SR-DI-BPM-023:Y", "SR-DI-BPM-024:Y", "SR-DI-BPM-025:Y", "SR-DI-BPM-026:Y", "SR-DI-BPM-027:Y", "SR-DI-BPM-031:Y", "SR-DI-BPM-032:Y", "SR-DI-BPM-033:Y", "SR-DI-BPM-034:Y", "SR-DI-BPM-035:Y", "SR-DI-BPM-036:Y", "SR-DI-BPM-037:Y", "SR-DI-BPM-041:Y", "SR-DI-BPM-042:Y", "SR-DI-BPM-043:Y", "SR-DI-BPM-044:Y", "SR-DI-BPM-045:Y", "SR-DI-BPM-046:Y", "SR-DI-BPM-047:Y", "SR-DI-BPM-048:Y", "SR-DI-BPM-050:Y", "SR-DI-BPM-051:Y", "SR-DI-BPM-052:Y", "SR-DI-BPM-053:Y", "SR-DI-BPM-054:Y", "SR-DI-BPM-055:Y", "SR-DI-BPM-056:Y", "SR-DI-BPM-057:Y", "SR-DI-BPM-061:Y", "SR-DI-BPM-062:Y", "SR-DI-BPM-063:Y", "SR-DI-BPM-064:Y", "SR-DI-BPM-065:Y", "SR-DI-BPM-066:Y", "SR-DI-BPM-067:Y", "SR-DI-BPM-071:Y", "SR-DI-BPM-072:Y", "SR-DI-BPM-073:Y", "SR-DI-BPM-074:Y", "SR-DI-BPM-075:Y", "SR-DI-BPM-076:Y", "SR-DI-BPM-077:Y", "SR-DI-BPM-081:Y", "SR-DI-BPM-082:Y", "SR-DI-BPM-083:Y", "SR-DI-BPM-084:Y", "SR-DI-BPM-085:Y", "SR-DI-BPM-086:Y", "SR-DI-BPM-087:Y", "SR-DI-BPM-091:Y", "SR-DI-BPM-092:Y", "SR-DI-BPM-093:Y", "SR-DI-BPM-094:Y", "SR-DI-BPM-095:Y", "SR-DI-BPM-096:Y", "SR-DI-BPM-097:Y", "SR-DI-BPM-101:Y", "SR-DI-BPM-102:Y", "SR-DI-BPM-103:Y", "SR-DI-BPM-104:Y", "SR-DI-BPM-105:Y", "SR-DI-BPM-106:Y", "SR-DI-BPM-107:Y", "SR-DI-BPM-111:Y", "SR-DI-BPM-112:Y", "SR-DI-BPM-113:Y", "SR-DI-BPM-114:Y", "SR-DI-BPM-115:Y", "SR-DI-BPM-116:Y", "SR-DI-BPM-117:Y", "SR-DI-BPM-121:Y", "SR-DI-BPM-122:Y", "SR-DI-BPM-123:Y", "SR-DI-BPM-124:Y", "SR-DI-BPM-125:Y", "SR-DI-BPM-126:Y", "SR-DI-BPM-127:Y", "SR-DI-BPM-128:Y", "SR-DI-BPM-130:Y", "SR-DI-BPM-131:Y", "SR-DI-BPM-132:Y", "SR-DI-BPM-133:Y", "SR-DI-BPM-134:Y", "SR-DI-BPM-135:Y", "SR-DI-BPM-136:Y", "SR-DI-BPM-137:Y", "SR-DI-BPM-141:Y", "SR-DI-BPM-142:Y", "SR-DI-BPM-143:Y", "SR-DI-BPM-144:Y", "SR-DI-BPM-145:Y", "SR-DI-BPM-146:Y", "SR-DI-BPM-147:Y", "SR-DI-BPM-151:Y", "SR-DI-BPM-152:Y", "SR-DI-BPM-153:Y", "SR-DI-BPM-154:Y", "SR-DI-BPM-155:Y", "SR-DI-BPM-156:Y", "SR-DI-BPM-157:Y", "SR-DI-BPM-161:Y", "SR-DI-BPM-162:Y", "SR-DI-BPM-163:Y", "SR-DI-BPM-164:Y", "SR-DI-BPM-165:Y", "SR-DI-BPM-166:Y", "SR-DI-BPM-167:Y", "SR-DI-BPM-171:Y", "SR-DI-BPM-172:Y", "SR-DI-BPM-173:Y", "SR-DI-BPM-174:Y", "SR-DI-BPM-175:Y", "SR-DI-BPM-176:Y", "SR-DI-BPM-177:Y", "SR-DI-BPM-181:Y", "SR-DI-BPM-182:Y", "SR-DI-BPM-183:Y", "SR-DI-BPM-184:Y", "SR-DI-BPM-185:Y", "SR-DI-BPM-186:Y", "SR-DI-BPM-187:Y", "SR-DI-BPM-191:Y", "SR-DI-BPM-192:Y", "SR-DI-BPM-193:Y", "SR-DI-BPM-194:Y", "SR-DI-BPM-195:Y", "SR-DI-BPM-196:Y", "SR-DI-BPM-197:Y", "SR-DI-BPM-201:Y", "SR-DI-BPM-202:Y", "SR-DI-BPM-203:Y", "SR-DI-BPM-204:Y", "SR-DI-BPM-205:Y", "SR-DI-BPM-206:Y", "SR-DI-BPM-207:Y", "SR-DI-BPM-208:Y", "SR-DI-BPM-210:Y", "SR-DI-BPM-211:Y", "SR-DI-BPM-212:Y", "SR-DI-BPM-213:Y", "SR-DI-BPM-214:Y", "SR-DI-BPM-215:Y", "SR-DI-BPM-216:Y", "SR-DI-BPM-217:Y", "SR-DI-BPM-221:Y", "SR-DI-BPM-222:Y", "SR-DI-BPM-223:Y", "SR-DI-BPM-224:Y", "SR-DI-BPM-225:Y", "SR-DI-BPM-226:Y", "SR-DI-BPM-227:Y", "SR-DI-BPM-231:Y", "SR-DI-BPM-232:Y", "SR-DI-BPM-233:Y", "SR-DI-BPM-234:Y", "SR-DI-BPM-235:Y", "SR-DI-BPM-236:Y", "SR-DI-BPM-237:Y", "SR-DI-BPM-241:Y", "SR-DI-BPM-242:Y", "SR-DI-BPM-243:Y", "SR-DI-BPM-244:Y", "SR-DI-BPM-245:Y", "SR-DI-BPM-246:Y", "SR-DI-BPM-247:Y"]  # sorted BPMY_174
    w329 = string[] ["SR-DI-BPM-011:X", "SR-DI-BPM-012:X", "SR-DI-BPM-013:X", "SR-DI-BPM-014:X", "SR-DI-BPM-015:X", "SR-DI-BPM-016:X", "SR-DI-BPM-017:X", "SR-DI-BPM-021:X", "SR-DI-BPM-022:X", "SR-DI-BPM-023:X", "SR-DI-BPM-024:X", "SR-DI-BPM-025:X", "SR-DI-BPM-026:X", "SR-DI-BPM-027:X", "SR-DI-BPM-031:X", "SR-DI-BPM-032:X", "SR-DI-BPM-033:X", "SR-DI-BPM-034:X", "SR-DI-BPM-035:X", "SR-DI-BPM-036:X", "SR-DI-BPM-037:X", "SR-DI-BPM-041:X", "SR-DI-BPM-042:X", "SR-DI-BPM-043:X", "SR-DI-BPM-044:X", "SR-DI-BPM-045:X", "SR-DI-BPM-046:X", "SR-DI-BPM-047:X", "SR-DI-BPM-048:X", "SR-DI-BPM-050:X", "SR-DI-BPM-051:X", "SR-DI-BPM-052:X", "SR-DI-BPM-053:X", "SR-DI-BPM-054:X", "SR-DI-BPM-055:X", "SR-DI-BPM-056:X", "SR-DI-BPM-057:X", "SR-DI-BPM-061:X", "SR-DI-BPM-062:X", "SR-DI-BPM-063:X", "SR-DI-BPM-064:X", "SR-DI-BPM-065:X", "SR-DI-BPM-066:X", "SR-DI-BPM-067:X", "SR-DI-BPM-071:X", "SR-DI-BPM-072:X", "SR-DI-BPM-073:X", "SR-DI-BPM-074:X", "SR-DI-BPM-075:X", "SR-DI-BPM-076:X", "SR-DI-BPM-077:X", "SR-DI-BPM-081:X", "SR-DI-BPM-082:X", "SR-DI-BPM-083:X", "SR-DI-BPM-084:X", "SR-DI-BPM-085:X", "SR-DI-BPM-086:X", "SR-DI-BPM-087:X", "SR-DI-BPM-091:X", "SR-DI-BPM-092:X", "SR-DI-BPM-093:X", "SR-DI-BPM-094:X", "SR-DI-BPM-095:X", "SR-DI-BPM-096:X", "SR-DI-BPM-097:X", "SR-DI-BPM-101:X", "SR-DI-BPM-102:X", "SR-DI-BPM-103:X", "SR-DI-BPM-104:X", "SR-DI-BPM-105:X", "SR-DI-BPM-106:X", "SR-DI-BPM-107:X", "SR-DI-BPM-111:X", "SR-DI-BPM-112:X", "SR-DI-BPM-113:X", "SR-DI-BPM-114:X", "SR-DI-BPM-115:X", "SR-DI-BPM-116:X", "SR-DI-BPM-117:X", "SR-DI-BPM-121:X", "SR-DI-BPM-122:X", "SR-DI-BPM-123:X", "SR-DI-BPM-124:X", "SR-DI-BPM-125:X", "SR-DI-BPM-126:X", "SR-DI-BPM-127:X", "SR-DI-BPM-128:X", "SR-DI-BPM-130:X", "SR-DI-BPM-131:X", "SR-DI-BPM-132:X", "SR-DI-BPM-133:X", "SR-DI-BPM-134:X", "SR-DI-BPM-135:X", "SR-DI-BPM-136:X", "SR-DI-BPM-137:X", "SR-DI-BPM-141:X", "SR-DI-BPM-142:X", "SR-DI-BPM-143:X", "SR-DI-BPM-144:X", "SR-DI-BPM-145:X", "SR-DI-BPM-146:X", "SR-DI-BPM-147:X", "SR-DI-BPM-151:X", "SR-DI-BPM-152:X", "SR-DI-BPM-153:X", "SR-DI-BPM-154:X", "SR-DI-BPM-155:X", "SR-DI-BPM-156:X", "SR-DI-BPM-157:X", "SR-DI-BPM-161:X", "SR-DI-BPM-162:X", "SR-DI-BPM-163:X", "SR-DI-BPM-164:X", "SR-DI-BPM-165:X", "SR-DI-BPM-166:X", "SR-DI-BPM-167:X", "SR-DI-BPM-171:X", "SR-DI-BPM-172:X", "SR-DI-BPM-173:X", "SR-DI-BPM-174:X", "SR-DI-BPM-175:X", "SR-DI-BPM-176:X", "SR-DI-BPM-177:X", "SR-DI-BPM-181:X", "SR-DI-BPM-182:X", "SR-DI-BPM-183:X", "SR-DI-BPM-184:X", "SR-DI-BPM-185:X", "SR-DI-BPM-186:X", "SR-DI-BPM-187:X", "SR-DI-BPM-191:X", "SR-DI-BPM-192:X", "SR-DI-BPM-193:X", "SR-DI-BPM-194:X", "SR-DI-BPM-195:X", "SR-DI-BPM-196:X", "SR-DI-BPM-197:X", "SR-DI-BPM-201:X", "SR-DI-BPM-202:X", "SR-DI-BPM-203:X", "SR-DI-BPM-204:X", "SR-DI-BPM-205:X", "SR-DI-BPM-206:X", "SR-DI-BPM-207:X", "SR-DI-BPM-208:X", "SR-DI-BPM-210:X", "SR-DI-BPM-211:X", "SR-DI-BPM-212:X", "SR-DI-BPM-213:X", "SR-DI-BPM-214:X", "SR-DI-BPM-215:X", "SR-DI-BPM-216:X", "SR-DI-BPM-217:X", "SR-DI-BPM-221:X", "SR-DI-BPM-222:X", "SR-DI-BPM-223:X", "SR-DI-BPM-224:X", "SR-DI-BPM-225:X", "SR-DI-BPM-226:X", "SR-DI-BPM-227:X", "SR-DI-BPM-231:X", "SR-DI-BPM-232:X", "SR-DI-BPM-233:X", "SR-DI-BPM-234:X", "SR-DI-BPM-235:X", "SR-DI-BPM-236:X", "SR-DI-BPM-237:X", "SR-DI-BPM-241:X", "SR-DI-BPM-242:X", "SR-DI-BPM-243:X", "SR-DI-BPM-244:X", "SR-DI-BPM-245:X", "SR-DI-BPM-246:X", "SR-DI-BPM-247:X"]  # sorted BPMX_174
    w388 = string[] ["BL-05A:HutchA_Enable", "BL-09A:HutchA_Enable", "BL-21A:HutchA_Enable", "BL-23A:HutchA_Enable", "BL-25A:HutchA_Enable", "BL-41A:HutchA_Enable", "BL-45A:HutchA_Enable"]  # Hutch enable
    w407 = string[] ["CPCI03-adl7452-0:doBank0Ch5", "CPCI05-adl7452-0:doBank0Ch5", "CPCI11-adl7452-0:doBank0Ch5", "CPCI12-adl7452-0:doBank0Ch5", "CPCI13-adl7452-0:doBank0Ch5", "CPCI21-adl7452-0:doBank0Ch5", "CPCI23-adl7452-0:doBank0Ch5"]  # FE enable
    w484 = 578.303 ("y")
    w489 = 1.202 ("y")
    # "032  OPStatus    2195\n037  OPStatus    1899"
    # "SR-DI-RF-FB:getStatus"
    # "V1.4.2 改成直接用最大最小值當作scale的最大最小值"
    # "D:\\LOG運轉紀錄\\2016"
    # "45"
    # "41"
    # "25"
    # "23"
    # "21"
    # "09"
    # "05"
    # "05\n09\n21\n23\n25\n41\n45"
    # "gapMotorOff"
    n36 = event shown="[3] \"Trip Evt B\": Value Change" {
      selector: _ -> [_ _ _ _ _ _ _ _ _ _ _]
      dyn-events: _ -> [_ _ _ _ _ _ _ _ _ _ _]
      timeout: 233 -> [_ _ _ _ _ _ _ _ _ _ _]
      tunnel: [_ w541 _ _ _ _ _ _ _ _ _] -> w84
      tunnel: [w526 w540 w547 w563 w704 w707 w844 w856 w882 w919 w924] -> w83
      tunnel: w82 -> [w526 w540 w547 _ w704 _ w844 w856 w882 w919 w924]
      tunnel: "last ? Hrs" -> [_ _ _ w564 _ w708 _ _ _ _ _]
      tunnel: w78 -> [_ w527 _ _ _ _ _ w855 _ w909 _]
      event Timeout {
        n37 = event-data() -> ()  [unwired: 1 in, 3 out]
      }
      event "stop": Value Change {
        n38 = event-data() -> ("NewVal"=w541:bool)  [unwired: 1 in, 3 out]
        n39 = Get Date/Time In Seconds() -> (seconds since 1Jan1904=w534:timestamp)
        n40 = To Double Precision Float(number=w534) -> (double precision float=w533:dbl)
        n41 = Subtract(x=w533, y=43200.0) -> (x-y=w530:dbl)
        n42 = call "Main_Daily_path.vi"() -> ("Directory path"=w535:path)  [unwired: 10 in, 1 out]
        n43 = Greater?(x=w530, y=w527) -> (0:w531:bool)
        n44 = Select(t=w530, s=w531, f=w527) -> (s? t:f=w529:dbl)
        n45 = call "B09_Save_new_lattice_files.vi"("For Test"=FALSE, "Directory Path"=w535) -> ()  [unwired: 10 in]
        n46 = call <vilib>:"Application Directory.vi"() -> ("Application Directory"=w528:path)
        n47 = local read "Diff list"() -> (w538:string[][])
        n48 = call "B07_Save_changed_PVs.vi"("For Test"=FALSE, "想要限制的筆數"=1000, "Directory Path"=w528, "紀錄起始時間  門檻"=w529, "diff_Value 2"=w538) -> ()  [unwired: 5 in, 2 out]
      }
      event "Open Button": Value Change {
        n49 = event-data() -> ()  [unwired: 1 in, 6 out]
        n50 = call <vilib>:"Beep.vi"("use system alert? (T)"=FALSE, "duration (msec)"=u32 40, "frequency (Hz)"=u32 1700) -> ()  [unwired: 9 in]
        n51 = call "Main_Daily_path.vi"() -> ("Directory path(STR)"=w546:string, "Directory path"=w545:path)  [unwired: 10 in]
        n52 = call <vilib>:"Check if File or Folder Exists.vi"("path"=w545) -> ("error out"=w551:errorcluster, "file or folder exists?"=w549:bool, "dup path"=w550:path)  [unwired: 8 in]
        n53 = case shown="False" w549 {
          tunnel: w550 -> [w558 w560]
          tunnel: w551 -> [w557 w559]
          tunnel: [w556 w560] -> _
          tunnel: [w555 w559] -> w548
          frame False {
            n54 = Create Folder(path (use dialog)=w558, error in=w557) -> (created path=w556:path, error out=w555:errorcluster)  [unwired: 1 in, 1 out]
          }
          frame True {
          }
        }
        n55 = Concatenate Strings("explorer ", w546) -> (w553:string)
        n56 = call <vilib>:"System Exec.vi"("wait until completion? (T)"=FALSE, "error in (no error)"=w548, "command line"=w553) -> ()  [unwired: 5 in, 4 out]
      }
      event "Trip Evt B": Value Change {
        n57 = event-data() -> ()  [unwired: 1 in, 1 out]
        n58 = flat-sequence {
          tunnel: w564 -> [w569]
          tunnel: [w569] -> w561
          tunnel: [w585] -> w562
          tunnel: w561 -> [w588]
          tunnel: [w699] -> w563
          tunnel: w562 -> [w699]
          frame #0 {
            n59 = property on="result" class="Str"("Visible"=FALSE) -> ()  [unwired: 2 in, 2 out]
            n60 = call <vilib>:"Beep.vi"("use system alert? (T)"=FALSE, "duration (msec)"=u32 40, "frequency (Hz)"=u32 1700) -> ()  [unwired: 9 in]
          }
          frame #1 {
            n61 = Get Date/Time In Seconds() -> (seconds since 1Jan1904=w592:timestamp)
            n62 = Multiply(x=3600.0 ("y"), y=w588) -> (x*y=w601:dbl)
            n63 = call "TimeToString.vi"("Time Stamp Control"=w592) -> ("result string"=w599:string)
            n64 = Subtract(x=w592, y=w601) -> (x-y=w593:timestamp)
            n65 = call "TimeToString.vi"("Time Stamp Control"=w593) -> ("result string"=w600:string)
            n66 = call <vilib>:"Application Directory.vi"() -> ("Application Directory"=w598:path)
            n67 = Build Path(base path=w598, name or relative path="DSN\\172-18-0-32.dsn") -> (appended path=w596:path)
            n68 = Concatenate Strings("SELECT  float_val , smpl_time\nFROM sample \nwhere  channel_id = 104 and smpl_time between '" ("result string"), w600, "' ::timestamp and '" ("result string"), w599, "' ::timestamp" ("result string")) -> (w613:string)
            n69 = call-poly <vilib>:"DB Tools Open Connection.vi"("connection information"=w596) -> ("error out"=w603:errorcluster, "connection reference"=w604:T2)  [unwired: 7 in]
            n70 = call-poly <vilib>:"DB Tools Execute Query.vi"("error in (no error)"=w603, "SQL query"=w613, "connection reference"=w604) -> ("error out"=w606:errorcluster, "recordset reference"=w605:T3)  [unwired: 5 in]
            n71 = call-poly <vilib>:"DB Tools Fetch Recordset Data.vi"("error in (no error)"=w606, "recordset reference"=w605) -> ("error out"=w589:errorcluster, "recordset data"=w572:variant[][], "recordset reference out"=w607:T3)  [unwired: 3 in]
            n72 = call-poly <vilib>:"DB Tools Free Object.vi"("error in (no error)"=w589, "recordset reference"=w607) -> ("error out"=w609:errorcluster, "connection reference"=w608:T2)  [unwired: 8 in]
            n73 = Transpose 2D Array(2D array=w572) -> (transposed array=w576:variant[][])
            n74 = call <vilib>:"DB Tools Close Connection.vi"("error in (no error)"=w609, "connection reference"=w608) -> ("error out"=→"error out 4":errorcluster)  [unwired: 5 in]
            n75 = Index Array(array=w576, index (row) #1=1 ("index (row)"), index (row) #2=0 ("index (row)")) -> (element #1=w578:variant[], element #2=w579:variant[])  [unwired: 2 in]
            n76 = xnode "Database Variant To Data"("database variant"=w578, "type"=timestamp[] []) -> ("data"=w571:timestamp[])  [unwired: 1 in, 1 out]
            n77 = Variant To Data(type=dbl[] [], Variant=w579) -> (data=w570:dbl[])  [unwired: 1 in, 1 out]
            n78 = control-ref of="BeamCurrent History"() -> (w587:refnum<vi>)
            n79 = for {
              tunnel: w570 -> [w692] mode=indexing
              tunnel: w571 -> [w691] mode=indexing
              shift-right: [w692] -> _
              shift-left: 0.0 -> [w693]
              tunnel: [w691] -> w615 mode=indexing if=w690
              tunnel: [w689] -> _ mode=indexing
              n80 = Subtract(x=w692, y=w693) -> (x-y=w689:dbl)
              n81 = Less Or Equal?(x=w689, y=-100.0) -> (x <= y?=w690:bool)
            }
            n82 = To Double Precision Float(number=w571) -> (double precision float=w586:dbl[])
            n83 = To Double Precision Float(number=w592) -> (double precision float=w594:dbl)
            n84 = Array Max & Min(array=w570) -> (max value=w591:dbl, min value=w590:dbl)  [unwired: 2 out]
            n85 = To Double Precision Float(number=w593) -> (double precision float=w595:dbl)
            n86 = property on="Property Node" class="XYGraph (strict)"(reference=w587, "XScale.Maximum"=w594, "XScale.Minimum"=w595, "YScale.Maximum"=w591, "YScale.Minimum"=w590) -> ()  [unwired: 1 in, 2 out]
            n87 = Bundle(w586, w570) -> (w585:cluster{dbl[], dbl[]})  [unwired: 1 in]
            n88 = Array Size(array=w615) -> (size(s)=w582:i32)
            n89 = for {
              tunnel: w615 -> [w686] mode=indexing
              tunnel: [w682] -> w616 mode=indexing
              i -> [w685]
              n90 = Increment(x=w685) -> (x+1=w684:i32)
              n91 = Format Date/Time String(time format string (%c)="%Y/%m/%d %H:%M", seconds (now)=w686) -> (date/time string=w683:string)  [unwired: 1 in]
              n92 = Number To Decimal String(number=w684) -> (decimal integer string=w681:string)  [unwired: 1 in]
              n93 = Concatenate Strings(w681, "." ("string")) -> (w679:string)
              n94 = Build Array(w679, w683) -> (w682:string[])
            }
            n95 = Number To Decimal String(number=w582) -> (decimal integer string=w622:string)  [unwired: 1 in]
            n96 = Build Array (concatenate)(string[] ["No.", "Event Time"], w616) -> (w620:string[][])
            n97 = Array To Spreadsheet String(delimiter (Tab)="", array=w620, 3:"%s" ("format string")) -> (spreadsheet string=w624:string)
            n98 = Concatenate Strings("Beam Trip Events \nTatal Counts: ", w622, "\n" ("string"), w624, "\n(Threshold:100mA)") -> (w581:string)
            n99 = case shown="0" w582 {
              tunnel: ["Beam Trip Events \nTotal Counts: 0" w678] -> w580
              tunnel: w581 -> [_ w678]
              frame 0 {
              }
              frame 1, Default {
              }
            }
            "result" <- w580
          }
          frame #2 {
            n100 = local write "Trip Evt B"(FALSE ("Trip Evt B")) -> ()
            n101 = property on="result" class="Str"("Visible"=TRUE) -> ()  [unwired: 2 in, 2 out]
            n102 = call <vilib>:"Beep.vi"("use system alert? (T)"=FALSE, "duration (msec)"=u32 40, "frequency (Hz)"=u32 2000) -> ()  [unwired: 9 in]
          }
        }
      }
      event "Switch Tab": Value Change {
        n103 = event-data() -> ("NewVal"=w703:bool)  [unwired: 1 in, 1 out]
        n104 = Select(t=enum32{"_____", "           "}."_____" ("Tab Control"), s=w703, f=enum32{"_____", "           "}."           " ("Tab Control")) -> (s? t:f=→"Tab Control":enum32{"_____", "           "})
      }
      event "Refresh B": Value Change {
        n105 = event-data() -> ()  [unwired: 1 in, 6 out]
        n106 = flat-sequence {
          tunnel: w708 -> [w713]
          tunnel: [w713] -> w705
          tunnel: [w729] -> w706
          tunnel: w705 -> [w732]
          tunnel: [w843] -> w707
          tunnel: w706 -> [w843]
          frame #0 {
            n107 = property on="result" class="Str"("Visible"=FALSE) -> ()  [unwired: 2 in, 2 out]
            n108 = call <vilib>:"Beep.vi"("use system alert? (T)"=FALSE, "duration (msec)"=u32 40, "frequency (Hz)"=u32 1700) -> ()  [unwired: 9 in]
          }
          frame #1 {
            n109 = Get Date/Time In Seconds() -> (seconds since 1Jan1904=w736:timestamp)
            n110 = Multiply(x=3600.0 ("y"), y=w732) -> (x*y=w745:dbl)
            n111 = call "TimeToString.vi"("Time Stamp Control"=w736) -> ("result string"=w743:string)
            n112 = Subtract(x=w736, y=w745) -> (x-y=w737:timestamp)
            n113 = call "TimeToString.vi"("Time Stamp Control"=w737) -> ("result string"=w744:string)
            n114 = call <vilib>:"Application Directory.vi"() -> ("Application Directory"=w742:path)
            n115 = Build Path(base path=w742, name or relative path="DSN\\172-18-0-32.dsn") -> (appended path=w740:path)
            n116 = Concatenate Strings("SELECT  float_val , smpl_time\nFROM sample \nwhere  channel_id = 104 and smpl_time between '" ("result string"), w744, "' ::timestamp and '" ("result string"), w743, "' ::timestamp" ("result string")) -> (w757:string)
            n117 = call-poly <vilib>:"DB Tools Open Connection.vi"("connection information"=w740) -> ("error out"=w747:errorcluster, "connection reference"=w748:T2)  [unwired: 7 in]
            n118 = call-poly <vilib>:"DB Tools Execute Query.vi"("error in (no error)"=w747, "SQL query"=w757, "connection reference"=w748) -> ("error out"=w750:errorcluster, "recordset reference"=w749:T3)  [unwired: 5 in]
            n119 = call-poly <vilib>:"DB Tools Fetch Recordset Data.vi"("error in (no error)"=w750, "recordset reference"=w749) -> ("error out"=w733:errorcluster, "recordset data"=w716:variant[][], "recordset reference out"=w751:T3)  [unwired: 3 in]
            n120 = call-poly <vilib>:"DB Tools Free Object.vi"("error in (no error)"=w733, "recordset reference"=w751) -> ("error out"=w753:errorcluster, "connection reference"=w752:T2)  [unwired: 8 in]
            n121 = Transpose 2D Array(2D array=w716) -> (transposed array=w720:variant[][])
            n122 = call <vilib>:"DB Tools Close Connection.vi"("error in (no error)"=w753, "connection reference"=w752) -> ("error out"=→"error out 5":errorcluster)  [unwired: 5 in]
            n123 = Index Array(array=w720, index (row) #1=1 ("index (row)"), index (row) #2=0 ("index (row)")) -> (element #1=w722:variant[], element #2=w723:variant[])  [unwired: 2 in]
            n124 = xnode "Database Variant To Data"("database variant"=w722, "type"=timestamp[] []) -> ("data"=w715:timestamp[])  [unwired: 1 in, 1 out]
            n125 = Variant To Data(type=dbl[] [], Variant=w723) -> (data=w714:dbl[])  [unwired: 1 in, 1 out]
            n126 = control-ref of="BeamCurrent History"() -> (w731:refnum<vi>)
            n127 = for {
              tunnel: w714 -> [w836] mode=indexing
              tunnel: w715 -> [w835] mode=indexing
              shift-right: [w836] -> _
              shift-left: 0.0 -> [w837]
              tunnel: [w835] -> w759 mode=indexing if=w834
              tunnel: [w833] -> _ mode=indexing
              n128 = Subtract(x=w836, y=w837) -> (x-y=w833:dbl)
              n129 = Less Or Equal?(x=w833, y=-100.0) -> (x <= y?=w834:bool)
            }
            n130 = To Double Precision Float(number=w715) -> (double precision float=w730:dbl[])
            n131 = To Double Precision Float(number=w736) -> (double precision float=w738:dbl)
            n132 = Array Max & Min(array=w714) -> (max value=w735:dbl, min value=w734:dbl)  [unwired: 2 out]
            n133 = To Double Precision Float(number=w737) -> (double precision float=w739:dbl)
            n134 = property on="Property Node" class="XYGraph (strict)"(reference=w731, "XScale.Maximum"=w738, "XScale.Minimum"=w739, "YScale.Maximum"=w735, "YScale.Minimum"=w734) -> ()  [unwired: 1 in, 2 out]
            n135 = Bundle(w730, w714) -> (w729:cluster{dbl[], dbl[]})  [unwired: 1 in]
            n136 = Array Size(array=w759) -> (size(s)=w726:i32)
            n137 = for {
              tunnel: w759 -> [w830] mode=indexing
              tunnel: [w826] -> w760 mode=indexing
              i -> [w829]
              n138 = Increment(x=w829) -> (x+1=w828:i32)
              n139 = Format Date/Time String(time format string (%c)="%Y/%m/%d %H:%M", seconds (now)=w830) -> (date/time string=w827:string)  [unwired: 1 in]
              n140 = Number To Decimal String(number=w828) -> (decimal integer string=w825:string)  [unwired: 1 in]
              n141 = Concatenate Strings(w825, "." ("string")) -> (w823:string)
              n142 = Build Array(w823, w827) -> (w826:string[])
            }
            n143 = Number To Decimal String(number=w726) -> (decimal integer string=w766:string)  [unwired: 1 in]
            n144 = Build Array (concatenate)(string[] ["No.", "Event Time"], w760) -> (w764:string[][])
            n145 = Array To Spreadsheet String(delimiter (Tab)="", array=w764, 3:"%s" ("format string")) -> (spreadsheet string=w768:string)
            n146 = Concatenate Strings("Beam Trip Events \nTatal Counts: ", w766, "\n" ("string"), w768, "\n(Threshold:100mA)") -> (w725:string)
            n147 = case shown="0" w726 {
              tunnel: ["Beam Trip Events \nTotal Counts: 0" w822] -> w724
              tunnel: w725 -> [_ w822]
              frame 0 {
              }
              frame 1, Default {
              }
            }
            n148 = local write "result"(w724) -> ()
          }
          frame #2 {
            n149 = local write "Refresh B"(FALSE ("Trip Evt B")) -> ()
            n150 = property on="result" class="Str"("Visible"=TRUE) -> ()  [unwired: 2 in, 2 out]
            n151 = call <vilib>:"Beep.vi"("use system alert? (T)"=FALSE, "duration (msec)"=u32 40, "frequency (Hz)"=u32 2000) -> ()  [unwired: 9 in]
          }
        }
      }
      event "Save Lattice Button": Value Change {
        n152 = event-data() -> ()  [unwired: 1 in, 2 out]
        n153 = flat-sequence {
          frame #0 {
            n154 = call <vilib>:"Beep.vi"("use system alert? (T)"=FALSE, "duration (msec)"=u32 40, "frequency (Hz)"=u32 1700) -> ()  [unwired: 9 in]
          }
          frame #1 {
            n155 = call "Main_Daily_path.vi"() -> ("Directory path"=w848:path)  [unwired: 10 in, 1 out]
            n156 = call "B09_Save_new_lattice_files.vi"("For Test"=FALSE, "Directory Path"=w848) -> ()  [unwired: 10 in]
          }
          frame #2 {
            n157 = call <vilib>:"Beep.vi"("use system alert? (T)"=FALSE, "duration (msec)"=u32 40, "frequency (Hz)"=u32 2000) -> ()  [unwired: 9 in]
          }
        }
      }
      event "View Diff Button": Value Change {
        n158 = event-data() -> ()  [unwired: 1 in, 1 out]
        n159 = flat-sequence {
          tunnel: w855 -> [w861]
          tunnel: [w867] -> w853
          tunnel: [w872] -> w854
          tunnel: w853 -> [w872]
          tunnel: w854 -> [w874]
          frame #0 {
            # "12小時為43200sec"
            # "Save file"
            n160 = Get Date/Time In Seconds() -> (seconds since 1Jan1904=w866:timestamp)
            n161 = To Double Precision Float(number=w866) -> (double precision float=w865:dbl)
            n162 = call <vilib>:"Beep.vi"("use system alert? (T)"=FALSE, "duration (msec)"=u32 40, "frequency (Hz)"=u32 1700) -> ()  [unwired: 9 in]
            n163 = Subtract(x=w865, y=43200.0) -> (x-y=w862:dbl)
            n164 = Greater?(x=w862, y=w861) -> (0:w863:bool)
            n165 = Select(t=w862, s=w863, f=w861) -> (s? t:f=w860:dbl)
            n166 = local read "Diff list"() -> (w871:string[][])
            n167 = call "Main_Daily_path.vi"() -> ("Directory path"=w870:path)  [unwired: 10 in, 1 out]
            n168 = call "B07_Save_changed_PVs.vi"("For Test"=FALSE, "想要限制的筆數"=1000, "Directory Path"=w870, "紀錄起始時間  門檻"=w860, "diff_Value 2"=w871) -> ("saved file path"=w867:path)  [unwired: 5 in, 1 out]
          }
          frame #1 {
            # "Wait"
            n169 = Wait (ms)(milliseconds to wait=u32 300) -> ()  [unwired: 1 out]
          }
          frame #2 {
            # "Show"
            n170 = Path To String(path=w874) -> (string=w876:string)
            n171 = Concatenate Strings("explorer ", w876) -> (w875:string)
            n172 = call <vilib>:"System Exec.vi"("command line"=w875) -> ()  [unwired: 7 in, 4 out]
          }
          frame #3 {
            n173 = local write "View Diff Button"(FALSE ("View Diff Button")) -> ()
            n174 = call <vilib>:"Beep.vi"("use system alert? (T)"=FALSE, "duration (msec)"=u32 40, "frequency (Hz)"=u32 2000) -> ()  [unwired: 9 in]
          }
        }
      }
      event "Show Check list Button": Value Change {
        n175 = event-data() -> ()  [unwired: 1 in, 1 out]
        n176 = flat-sequence {
          frame #0 {
            n177 = call <vilib>:"Beep.vi"("use system alert? (T)"=FALSE, "duration (msec)"=u32 40, "frequency (Hz)"=u32 1700) -> ()  [unwired: 9 in]
          }
          frame #1 {
            n178 = local read "PV list"() -> (w886:string[])
            n179 = Array Size(array=w886) -> (size(s)=w887:i32)
            n180 = Array To Spreadsheet String(delimiter (Tab)="</BR>\n\r", array=w886, 3:"%s" ("format string")) -> (spreadsheet string=w898:string)
            n181 = Number To Decimal String(number=w887) -> (decimal integer string=w897:string)  [unwired: 1 in]
            n182 = call <vilib>:"Application Directory.vi"() -> ("Application Directory"=w888:path)
            n183 = Concatenate Strings("Tatal Checked PVs: ", w897, "</BR>\n\r" ("string"), w898) -> (w899:string)
            n184 = Build Path(base path=w888, name or relative path="Checked PV list.html") -> (appended path=w900:path)
            n185 = Write to Text File(file (use dialog)=w900, text=w899) -> ()  [unwired: 2 in, 3 out]
            n186 = flat-sequence {
              tunnel: w900 -> [w902]
              tunnel: [w902] -> w901
              frame #0 {
                n187 = Wait (ms)(milliseconds to wait=u32 500) -> ()  [unwired: 1 out]
              }
            }
            n188 = Path To String(path=w901) -> (string=w891:string)
            n189 = Concatenate Strings("explorer ", w891) -> (w890:string)
            n190 = call <vilib>:"System Exec.vi"("command line"=w890) -> ()  [unwired: 7 in, 4 out]
          }
          frame #2 {
            n191 = call <vilib>:"Beep.vi"("use system alert? (T)"=FALSE, "duration (msec)"=u32 40, "frequency (Hz)"=u32 2000) -> ()  [unwired: 9 in]
          }
        }
      }
      event Panel Close {
        n192 = event-data() -> ()  [unwired: 1 in, 2 out]
        n193 = Get Date/Time In Seconds() -> (seconds since 1Jan1904=w914:timestamp)
        n194 = To Double Precision Float(number=w914) -> (double precision float=w913:dbl)
        n195 = Subtract(x=w913, y=43200.0) -> (x-y=w910:dbl)
        n196 = call "Main_Daily_path.vi"() -> ("Directory path"=w915:path)  [unwired: 10 in, 1 out]
        n197 = Greater?(x=w910, y=w909) -> (0:w911:bool)
        n198 = Select(t=w910, s=w911, f=w909) -> (s? t:f=w908:dbl)
        n199 = call "B09_Save_new_lattice_files.vi"("For Test"=FALSE, "Directory Path"=w915) -> ()  [unwired: 10 in]
        n200 = call <vilib>:"Application Directory.vi"() -> ("Application Directory"=w907:path)
        n201 = local read "Diff list"() -> (w918:string[][])
        n202 = call "B07_Save_changed_PVs.vi"("For Test"=FALSE, "想要限制的筆數"=5000, "Directory Path"=w907, "紀錄起始時間  門檻"=w908, "diff_Value 2"=w918) -> ()  [unwired: 5 in, 2 out]
      }
      event "Save Button": Value Change {
        n203 = event-data() -> ()  [unwired: 1 in, 1 out]
        n204 = call <vilib>:"Beep.vi"("use system alert? (T)"=FALSE, "duration (msec)"=u32 40, "frequency (Hz)"=u32 1700) -> ()  [unwired: 9 in]
        n205 = Get Date/Time In Seconds() -> (seconds since 1Jan1904=w927:timestamp)
        n206 = Format Date/Time String(time format string (%c)="%Y", seconds (now)=w927, UTC format=FALSE) -> (date/time string=w946:string)
        n207 = Format Date/Time String(time format string (%c)="%d", seconds (now)=w927, UTC format=FALSE) -> (date/time string=w955:string)
        n208 = call "to_be_2_string.vi"("string 2"=w955) -> ("substring 2"=w956:string)  [unwired: 10 in]
        n209 = Format Date/Time String(time format string (%c)="%m", seconds (now)=w927, UTC format=FALSE) -> (date/time string=w950:string)
        n210 = Format Date/Time String(time format string (%c)="%Y%m%d%H%M%S", seconds (now)=w927) -> (date/time string=w934:string)  [unwired: 1 in]
        n211 = Concatenate Strings("D" ("磁碟位置"), ":\\LOG運轉紀錄\\", w946, "\\", w950, "\\", w956) -> (w939:string)
        n212 = String To Path(string=w939) -> (path=w942:path)
        n213 = call <vilib>:"Check if File or Folder Exists.vi"("path"=w942) -> ("error out"=w940:errorcluster, "file or folder exists?"=w954:bool, "dup path"=w941:path)  [unwired: 8 in]
        n214 = invoke on="Cluster" class="Clust (strict)" method="Get Image"() -> ("image data"=w925:T4)  [unwired: 6 in, 5 out]
        n215 = case shown="False" w954 {
          tunnel: w941 -> [w960 w962]
          tunnel: w940 -> [w959 w961]
          tunnel: [w958 w962] -> w926
          tunnel: [w957 w961] -> _
          frame False {
            n216 = Create Folder(path (use dialog)=w960, error in=w959) -> (created path=w958:path, error out=w957:errorcluster)  [unwired: 1 in, 1 out]
          }
          frame True {
          }
        }
        n217 = Path To String(path=w926) -> (string=w938:string)
        n218 = Concatenate Strings(w938, "\\" ("string"), w934) -> (w928:string)
        n219 = Concatenate Strings(w928, ".jpg" ("file format")) -> (w929:string)
        n220 = String To Path(string=w929) -> (path=w933:path)
        n221 = call <vilib>:"Write JPEG File.vi"("quality (80)"=100, "image data"=w925, "path to JPEG file"=w933) -> ("error out"=→"error out 3":errorcluster)  [unwired: 7 in, 1 out]
      }
    }
    n222 = call-poly <userlib>:"CaLabGet.vi"("PV Names"=string[] ["FE-DI-XBPM-051:signals:sa.X", "FE-DI-XBPM-051:signals:sa.Y", "FE-DI-XBPM-091:SA:SA_X_MONITOR", "FE-DI-XBPM-091:SA:SA_Y_MONITOR", "FE-DI-XBPM-211:SA:SA_X_MONITOR", "FE-DI-XBPM-211:SA:SA_Y_MONITOR", "FE-DI-XBPM-231:SA:SA_X_MONITOR", "FE-DI-XBPM-231:SA:SA_Y_MONITOR", "FE-DI-XBPM-251:SA:SA_X_MONITOR", "FE-DI-XBPM-251:SA:SA_Y_MONITOR", "FE-DI-XBPM-411:SA:SA_X_MONITOR", "FE-DI-XBPM-411:SA:SA_Y_MONITOR", "FE-DI-XBPM-451:SA:SA_X_MONITOR", "FE-DI-XBPM-451:SA:SA_Y_MONITOR", "FE-DI-XBPM-052:signals:sa.X", "FE-DI-XBPM-052:signals:sa.Y", "FE-DI-XBPM-092:SA:SA_X_MONITOR", "FE-DI-XBPM-092:SA:SA_Y_MONITOR", "FE-DI-XBPM-212:SA:SA_X_MONITOR", "FE-DI-XBPM-212:SA:SA_Y_MONITOR", "FE-DI-XBPM-232:SA:SA_X_MONITOR", "FE-DI-XBPM-232:SA:SA_Y_MONITOR", "FE-DI-XBPM-252:SA:SA_X_MONITOR", "FE-DI-XBPM-252:SA:SA_Y_MONITOR", "FE-DI-XBPM-412:SA:SA_X_MONITOR", "FE-DI-XBPM-412:SA:SA_Y_MONITOR", "FE-DI-XBPM-452:SA:SA_X_MONITOR", "FE-DI-XBPM-452:SA:SA_Y_MONITOR"] ("appended array")) -> ("1rst Value (number)"=w355:dbl[])  [unwired: 8 in, 6 out]
    n223 = Multiply(x=w355, y=0.001) -> (x*y=w354:dbl[])
    n224 = disable-structure shown="Disabled" {
      frame Disabled {
        n225 = To Long Integer() -> (32bit integer=w1007:i32)  [unwired: 1 in]
        n226 = case shown="1" w1007 {
          tunnel: ["Decay" "Top-Up"] -> _
          frame 0, Default {
          }
          frame 1 {
          }
        }
      }
      frame Enabled {
      }
    }
    n227 = call-poly <userlib>:"CaLabGet.vi"("PV Names"=string[] ["SR-DI-FP:CurrentBuffer"]) -> ("Value Array (number)"=w425:dbl[][])  [unwired: 8 in, 6 out]
    n228 = Index Array(array=w425, index (row)=0 ("index")) -> (element=w70:dbl[])  [unwired: 1 in]
    n229 = Index Array(array=w354, index #1=0 ("index"), index #2=1 ("index"), index #3=2 ("index"), index #4=3 ("index"), index #5=4 ("index"), index #6=5 ("index"), index #7=6 ("index"), index #8=7 ("index"), index #9=8 ("index"), index #10=9 ("index"), index #11=10 ("index"), index #12=11 ("index"), index #13=12 ("index"), index #14=13 ("index"), index #15=14 ("index"), index #16=15 ("index"), index #17=16 ("index"), index #18=17 ("index"), index #19=18 ("index"), index #20=19 ("index"), index #21=20 ("index"), index #22=21 ("index"), index #23=22 ("index"), index #24=23 ("index"), index #25=24 ("index"), index #26=25 ("index"), index #27=26 ("index"), index #28=27 ("index")) -> (element #1=w272:dbl, element #2=w265:dbl, element #3=w271:dbl, element #4=w264:dbl, element #5=w270:dbl, element #6=w263:dbl, element #7=w269:dbl, element #8=w262:dbl, element #9=w268:dbl, element #10=w261:dbl, element #11=w267:dbl, element #12=w260:dbl, element #13=w266:dbl, element #14=w259:dbl, element #15=w164:dbl, element #16=w163:dbl, element #17=w162:dbl, element #18=w161:dbl, element #19=w152:dbl, element #20=w151:dbl, element #21=w146:dbl, element #22=w145:dbl, element #23=w144:dbl, element #24=w143:dbl, element #25=w112:dbl, element #26=w111:dbl, element #27=w110:dbl, element #28=w109:dbl)
    n230 = Build Array (concatenate)(w70, w70) -> (w66:dbl[])
    n231 = for {
      tunnel: w66 -> [w524] mode=indexing
      shift-right: [w518] -> _
      shift-left: _ -> [w517]
      shift-right: [w521] -> _
      shift-left: 0 -> [w522]
      tunnel: [w519] -> w72 mode=indexing if=w512
      w523 = 0.05  # Threshold
      n232 = Increment(x=w522) -> (x+1=w519:i32)
      n233 = Less Or Equal?(x=w524, y=w523) -> (x <= y?=w518:bool)
      n234 = Not Equal?(x=w518, y=w517) -> ()  [unwired: 1 out]
      n235 = Equal?(x=w518, y=TRUE) -> (x = y?=w509:bool)
      n236 = Equal?(x=w517, y=FALSE) -> (x = y?=w508:bool)
      n237 = Equal?(x=w518, y=FALSE) -> (x = y?=w514:bool)
      n238 = Equal?(x=w517, y=TRUE) -> (x = y?=w513:bool)
      n239 = And(x=w509, y=w508) -> (x .and. y?=w507:bool)
      n240 = And(x=w514, y=w513) -> (x .and. y?=w512:bool)
      n241 = Select(t=0, s=w507, f=w519) -> (s? t:f=w521:i32)
    }
    n242 = Array Max & Min(array=w72) -> (max value=w73:i32)  [unwired: 3 out]
    n243 = Multiply(x=w73, y=2) -> (x*y=w69:i32)
    n244 = call-poly <userlib>:"CaLabGet.vi"("PV Names"=string[] ["LI-ES-CPS-01:PULSEMODE", "LI-ES-BPS-01:SETU:GRID", "LI-ES-BPS-01:SETU:MBM", "LI-ES-BPS-01:SETU:SBM", "LI-RF-HVP-31:SET:U", "CPCITM-TI-EVRTG:Pulse6DelaySet", "CPCITM-TI-EVRTG:Pulse7DelaySet", "CPCITM-TI-EVRTG:Pulse6WidthSet", "CPCITM-TI-EVRTG:Pulse7WidthSet", "CPCITM-TI-EVRTG:GTX6CtrlGTXPHSet", "CPCITM-TI-EVRTG:GTX7CtrlGTXPHSet", "CPCITM-TI-EVRTG:GTX6DlySet", "CPCITM-TI-EVRTG:GTX7DlySet"]) -> ("1rst Value (string)"=w417:string[], "1rst Value (number)"=w468:dbl[])  [unwired: 8 in, 5 out]
    n245 = call-poly <userlib>:"CaLabGet.vi"("PV Names"=string[] ["BR-PS-INJ-SE:setHV", "BR-PS-INJ-KI:setHV", "BR-PS-EXT-K1:setHV", "BR-PS-EXT-K2:setHV", "BR-PS-EXT-SE1:setHV", "BR-PS-EXT-SE2:setHV", "SR-PS-INJ-SE1:setHV", "SR-PS-INJ-SE2:setHV", "SR-PS-INJ-K1:setHV", "SR-PS-INJ-K2:setHV", "SR-PS-INJ-K3:setHV", "SR-PS-INJ-K4:setHV"]) -> ("1rst Value (number)"=w470:dbl[])  [unwired: 8 in, 6 out]
    n246 = call-poly <userlib>:"CaLabGet.vi"("PV Names"=string[] ["SR-RF-MSG:setFreq", "SR-RF2-LLRF:local", "SR-RF2-LLRF:getOperationMode", "SR-RF2-LLRF:getGapVoltage", "SR-RF2-LLRF:setGapVoltage", "SR-RF2-LLRF:setStationPhase", "SR-RF3-LLRF:local", "SR-RF3-LLRF:getOperationMode", "SR-RF3-LLRF:getGapVoltage", "SR-RF3-LLRF:setGapVoltage", "SR-RF3-LLRF:setStationPhase"]) -> ("1rst Value (number)"=w443:dbl[])  [unwired: 8 in, 6 out]
    n247 = call-poly <userlib>:"CaLabGet.vi"("PV Names"=string[] ["TI-INJ-PROC:TopupHiLowStart", "SR-DI-DCCT:BeamCurrent", "SR-DI-DCCT:BeamLifetime", "SR-DI-XPC-40:SigmaX", "SR-DI-XPC-40:SigmaY", "SR-DI-TUNE:nux", "SR-DI-TUNE:nuy", "IGPF:TPSX:SRAM:VEC:PEAKFREQ2", "IGPF:TPSY:SRAM:VEC:PEAKFREQ2", "TI-INJ-PROC:setBucketAddressStart", "TI-INJ-PROC:setBucketAddressLast", "TI-INJ-PROC:setBucketAddressStep"]) -> ("1rst Value (number)"=w504:dbl[])  [unwired: 8 in, 6 out]
    n248 = call-poly <userlib>:"CaLabGet.vi"("PV Names"=string[] ["LI:restoreFilename", "LTB:restoreFilename", "BR:restoreFilename", "BTS:restoreFilename", "SR:restoreFilename"]) -> ("1rst Value (string)"=w427:string[])  [unwired: 8 in, 6 out]
    n249 = Index Array(array=w417, index=0) -> (element=w415:string)
    n250 = Index Array(array=w468, index #1=0 ("index"), index #2=1 ("index"), index #3=2 ("index"), index #4=3 ("index"), index #5=4 ("index"), index #6=5 ("index"), index #7=6 ("index"), index #8=7 ("index"), index #9=8 ("index"), index #10=9 ("index"), index #11=10 ("index"), index #12=11 ("index"), index #13=12 ("index")) -> (element #2=w304:dbl, element #3=w419:dbl, element #4=w418:dbl, element #5=w302:dbl, element #8=w414:dbl, element #9=w413:dbl, element #10=w412:dbl, element #11=w411:dbl, element #12=w410:dbl, element #13=w409:dbl)  [unwired: 3 out]
    n251 = Index Array(array=w470, index #1=0 ("index"), index #2=1 ("index"), index #3=2 ("index"), index #4=3 ("index"), index #5=4 ("index"), index #6=5 ("index"), index #7=6 ("index"), index #8=7 ("index"), index #9=8 ("index"), index #10=9 ("index"), index #11=10 ("index"), index #12=11 ("index")) -> (element #1=w317:dbl, element #2=w316:dbl, element #3=w315:dbl, element #4=w314:dbl, element #5=w313:dbl, element #6=w312:dbl, element #7=w311:dbl, element #8=w310:dbl, element #9=w309:dbl, element #10=w308:dbl, element #11=w307:dbl, element #12=w306:dbl)
    n252 = Index Array(array=w443, index #1=0 ("index"), index #2=1 ("index"), index #3=2 ("index"), index #4=3 ("index"), index #5=4 ("index"), index #6=5 ("index"), index #7=6 ("index"), index #8=7 ("index"), index #9=8 ("index"), index #10=9 ("index"), index #11=10 ("index")) -> (element #1=w296:dbl, element #2=w440:dbl, element #3=w438:dbl, element #5=w220:dbl, element #6=w221:dbl, element #7=w435:dbl, element #8=w434:dbl, element #10=w292:dbl, element #11=w293:dbl)  [unwired: 2 out]
    n253 = Index Array(array=w504, index #1=0 ("index"), index #2=1 ("index"), index #3=2 ("index"), index #4=3 ("index"), index #5=4 ("index"), index #6=5 ("index"), index #7=6 ("index"), index #8=7 ("index"), index #9=8 ("index"), index #10=9 ("index"), index #11=10 ("index"), index #12=11 ("index")) -> (element #1=w502:dbl, element #2=w326:dbl, element #3=w325:dbl, element #4=w490:dbl, element #5=w488:dbl, element #6=w487:dbl, element #7=w486:dbl, element #8=w485:dbl, element #9=w483:dbl, element #10=w320:dbl, element #11=w319:dbl, element #12=w318:dbl)
    n254 = call-poly <userlib>:"CaLabGet.vi"("PV Names"=w194) -> ("1rst Value (number)"=w196:dbl[])  [unwired: 8 in, 6 out]
    n255 = Index Array(array=w427, index #1=0 ("index"), index #2=1 ("index"), index #3=2 ("index"), index #4=3 ("index"), index #5=4 ("index")) -> (element #1=w288:string, element #2=w287:string, element #3=w291:string, element #4=w290:string, element #5=w289:string)
    n256 = call-poly <userlib>:"CaLabGet.vi"("PV Names"=w388) -> ("1rst Value (string)"=w396:string[])  [unwired: 8 in, 6 out]
    n257 = To Byte Integer(number=w196) -> (8bit integer=w195:i8[])
    n258 = for {
      tunnel: w195 -> [w966] mode=indexing
      tunnel: [w963] -> w172 mode=indexing
      n259 = Number To Boolean Array(number=w966) -> (Boolean array=w965:bool[])
      n260 = Index Array(array=w965, index=0) -> (element=w963:bool)
    }
    n261 = for {
      tunnel: w396 -> [w976] mode=indexing
      tunnel: [w975] -> w397 mode=indexing
      n262 = case shown="\"Enable\"" w976 {
        tunnel: [FALSE TRUE] -> w975
        frame "Disable", Default {
        }
        frame "Enable" {
        }
      }
    }
    n263 = call-poly <userlib>:"CaLabGet.vi"("PV Names"=w407) -> ("1rst Value (string)"=w399:string[])  [unwired: 8 in, 6 out]
    n264 = call-poly <userlib>:"CaLabGet.vi"("PV Names"=string[] ["SR-ID-IU22-05:getGap", "SR-ID-IU22A-09:getGap", "SR-ID-IU22B-09:getGap", "SR-ID-IUT22-21:getGap", "SR-ID-IU22-23:getGap", "SR-ID-IU22A-25:getGap", "SR-ID-IU22B-25:getGap", "SR-ID-EPU48A-41:getGap", "SR-ID-EPU48A-41:getPhase", "SR-ID-EPU48B-41:getGap", "SR-ID-EPU48B-41:getPhase", "SR-ID-EPU46-45:getGap", "SR-ID-EPU46-45:getPhase", "SR-ID-IUT22-21:getGapTaper", "SR-ID-EPU48PS-41:getGap"]) -> ("1rst Value (number)"=w387:dbl[])  [unwired: 8 in, 6 out]
    n265 = for {
      tunnel: w399 -> [w980] mode=indexing
      tunnel: [w979] -> w398 mode=indexing
      n266 = case shown="\"enable\"" w980 {
        tunnel: [FALSE TRUE] -> w979
        frame "disable", Default {
        }
        frame "enable" {
        }
      }
    }
    n267 = call-poly <userlib>:"CaLabGet.vi"("PV Names"=string[] ["SR-ID-IU22-05:gapMotorOff", "SR-ID-IU22A-09:gapMotorOff", "SR-ID-IU22B-09:gapMotorOff", "SR-ID-IUT22-21:gapMotorOff", "SR-ID-IU22-23:gapMotorOff", "SR-ID-IU22A-25:gapMotorOff", "SR-ID-IU22B-25:gapMotorOff", "SR-ID-EPU48A-41:gapMotorOff", "SR-ID-EPU48B-41:gapMotorOff", "SR-ID-EPU46-45:gapMotorOff", "SR-ID-EPU48A-41:phaseMotorOff", "SR-ID-EPU48B-41:phaseMotorOff", "SR-ID-EPU46-45:phaseMotorOff"]) -> ("1rst Value (string)"=w339:string[])  [unwired: 8 in, 6 out]
    n268 = To Long Integer(number=w438) -> (32bit integer=w439:i32)
    n269 = To Long Integer(number=w440) -> (32bit integer=w441:i32)
    n270 = To Long Integer(number=w434) -> (32bit integer=w437:i32)
    n271 = To Long Integer(number=w435) -> (32bit integer=w436:i32)
    n272 = Index Array(array=w387, index #1=0 ("index"), index #2=1 ("index"), index #3=2 ("index"), index #4=3 ("index"), index #5=4 ("index"), index #6=5 ("index"), index #7=6 ("index"), index #8=7 ("index"), index #9=8 ("index"), index #10=9 ("index"), index #11=10 ("index"), index #12=11 ("index"), index #13=12 ("index"), index #14=13 ("index"), index #15=14 ("index")) -> (element #1=w286:dbl, element #2=w285:dbl, element #3=w284:dbl, element #4=w283:dbl, element #5=w282:dbl, element #6=w281:dbl, element #7=w280:dbl, element #8=w279:dbl, element #9=w278:dbl, element #10=w277:dbl, element #11=w276:dbl, element #12=w275:dbl, element #13=w274:dbl, element #14=w219:dbl, element #15=w273:dbl)
    n273 = for {
      tunnel: w339 -> [w972] mode=indexing
      tunnel: [w971] -> w338 mode=indexing
      n274 = case shown="\"1\", Default" w972 {
        tunnel: [FALSE TRUE] -> w971
        frame "1", Default {
        }
        frame "0" {
        }
      }
    }
    n275 = Index Array(array=w172, index #1=0 ("index"), index #2=1 ("index"), index #3=2 ("index"), index #4=3 ("index"), index #5=4 ("index"), index #6=5 ("index"), index #7=6 ("index"), index #8=7 ("index"), index #9=8 ("index"), index #10=9 ("index"), index #11=10 ("index"), index #12=11 ("index"), index #13=12 ("index"), index #14=13 ("index"), index #15=14 ("index"), index #16=15 ("index"), index #17=16 ("index"), index #18=17 ("index"), index #19=18 ("index"), index #20=19 ("index"), index #21=20 ("index")) -> (element #1=w169:bool, element #2=w168:bool, element #3=w167:bool, element #4=w156:bool, element #5=w155:bool, element #6=w154:bool, element #7=w149:bool, element #8=w148:bool, element #9=w147:bool, element #10=w138:bool, element #11=w137:bool, element #12=w136:bool, element #13=w131:bool, element #14=w130:bool, element #15=w129:bool, element #16=w128:bool, element #17=w127:bool, element #18=w126:bool, element #19=w125:bool, element #20=w124:bool, element #21=w123:bool)
    n276 = case shown="1" w441 {
      tunnel: [FALSE TRUE] -> w298
      frame 0, Default {
      }
      frame 1 {
      }
    }
    n277 = case shown="1" w436 {
      tunnel: [FALSE TRUE] -> w295
      frame 0, Default {
      }
      frame 1 {
      }
    }
    n278 = case shown="0" w439 {
      tunnel: [TRUE FALSE] -> w297
      frame 0 {
      }
      frame 1, Default {
      }
    }
    n279 = case shown="0" w437 {
      tunnel: [TRUE FALSE] -> w294
      frame 0 {
      }
      frame 1, Default {
      }
    }
    n280 = To Long Integer(number=w502) -> (32bit integer=w505:i32)
    n281 = Negate(x=w219) -> (-x=w218:dbl)
    n282 = case shown="1" w505 {
      tunnel: ["Decay" "Top-Up"] -> w327
      frame 0, Default {
      }
      frame 1 {
      }
    }
    n283 = Index Array(array=w397, index #1=0 ("index"), index #2=1 ("index"), index #3=2 ("index"), index #4=3 ("index"), index #5=4 ("index"), index #6=5 ("index"), index #7=6 ("index")) -> (element #1=w170:bool, element #2=w166:bool, element #3=w150:bool, element #4=w133:bool, element #5=w132:bool, element #6=w114:bool, element #7=w113:bool)
    n284 = case shown="\"MBM\", Default" w415 {
      tunnel: ["MBM" "SBM"] -> w305
      tunnel: w419 -> [w986 _]
      tunnel: [w986 w991] -> w303
      tunnel: w418 -> [_ w991]
      tunnel: w414 -> [_ w990]
      tunnel: w413 -> [w985 _]
      tunnel: [w985 w990] -> w301
      tunnel: w412 -> [_ w989]
      tunnel: w411 -> [w984 _]
      tunnel: [w984 w989] -> w300
      tunnel: w410 -> [_ w988]
      tunnel: w409 -> [w983 _]
      tunnel: [w983 w988] -> w299
      frame "MBM", Default {
      }
      frame "SBM" {
      }
    }
    n285 = Multiply(x=w490, y=w489) -> (x*y=w324:dbl)
    n286 = Divide(x=w485, y=w484) -> (x/y=w322:dbl)
    n287 = Multiply(x=w488, y=w489) -> (x*y=w323:dbl)
    n288 = Divide(x=w483, y=w484) -> (x/y=w321:dbl)
    n289 = Index Array(array=w398, index #1=0 ("index"), index #2=1 ("index"), index #3=2 ("index"), index #4=3 ("index"), index #5=4 ("index"), index #6=5 ("index"), index #7=6 ("index")) -> (element #1=w171:bool, element #2=w165:bool, element #3=w153:bool, element #4=w135:bool, element #5=w134:bool, element #6=w116:bool, element #7=w115:bool)
    n290 = call "FE_PAB_OpenState.vi"("FE"=w171, "XBPMX 2"=w164, "XBPMY 2"=w163, "Hutch"=w170, "PAB"=w169, "MGV"=w168, "FCV"=w167) -> ("XBPMX 2"=w160:string, "XBPMY 2"=w159:string)  [unwired: 7 in]
    n291 = call "FE_PAB_OpenState.vi"("FE"=w165, "XBPMX 2"=w162, "XBPMY 2"=w161, "Hutch"=w166, "PAB"=w156, "MGV"=w155, "FCV"=w154) -> ("XBPMX 2"=w158:string, "XBPMY 2"=w157:string)  [unwired: 7 in]
    n292 = call-poly <userlib>:"CaLabGet.vi"("PV Name"="TI-INJ-PROC:getTrig-SR-KICKER") -> ("1rst Value (string)"=w422:string)  [unwired: 8 in, 6 out]
    n293 = Index Array(array=w338, index #1=0 ("index"), index #2=1 ("index"), index #3=2 ("index"), index #4=3 ("index"), index #5=4 ("index"), index #6=5 ("index"), index #7=6 ("index"), index #8=7 ("index"), index #9=8 ("index"), index #10=9 ("index"), index #11=10 ("index"), index #12=11 ("index"), index #13=12 ("index")) -> (element #1=w258:bool, element #2=w257:bool, element #3=w256:bool, element #4=w255:bool, element #5=w254:bool, element #6=w253:bool, element #7=w252:bool, element #8=w251:bool, element #9=w250:bool, element #10=w249:bool, element #11=w248:bool, element #12=w247:bool, element #13=w246:bool)
    n294 = call-poly <userlib>:"CaLabGet.vi"("PV Names"=w329) -> ("1rst Value (number)"=w331:dbl[])  [unwired: 8 in, 6 out]
    n295 = call-poly <userlib>:"CaLabGet.vi"("PV Names"=w330) -> ("1rst Value (number)"=w333:dbl[])  [unwired: 8 in, 6 out]
    n296 = call "FE_PAB_OpenState.vi"("FE"=w153, "XBPMX 2"=w152, "XBPMY 2"=w151, "Hutch"=w150, "PAB"=w149, "MGV"=w148, "FCV"=w147) -> ("XBPMX 2"=w142:string, "XBPMY 2"=w141:string)  [unwired: 7 in]
    n297 = call-poly <userlib>:"CaLabGet.vi"("PV Names"=string[] ["SR-DI-FOFB-H:getStatus", "SR-DI-FOFB-V:getStatus", "IGPF:TPSX:FBCTRL", "IGPF:TPSY:FBCTRL", "TPS-SR-022:bpm3:ilk:enabled", "SR-DI-ANGLE-ILK:StatusX", "SR-DI-ANGLE-ILK:StatusY", "SR-DI-RF-FB:getStatus"]) -> ("1rst Value (string)"=w234:string[], "1rst Value (number)"=w235:dbl[])  [unwired: 8 in, 5 out]
    n298 = call "FE_PAB_OpenState.vi"("FE"=w135, "XBPMX 2"=w146, "XBPMY 2"=w145, "Hutch"=w133, "PAB"=w138, "MGV"=w137, "FCV"=w136) -> ("XBPMX 2"=w140:string, "XBPMY 2"=w139:string)  [unwired: 7 in]
    n299 = Multiply(x=w331, y=w332) -> (x*y=w212:dbl[])
    n300 = To Byte Integer(number=w235) -> (8bit integer=w231:i8[])
    n301 = Multiply(x=w333, y=w332) -> (x*y=w213:dbl[])
    n302 = for {
      tunnel: w231 -> [w968] mode=indexing
      tunnel: [w967] -> w241 mode=indexing
      n303 = case shown="1" w968 {
        tunnel: [TRUE FALSE] -> w967
        frame 1 {
        }
        frame 0, Default {
        }
      }
    }
    n304 = call "FE_PAB_OpenState.vi"("FE"=w134, "XBPMX 2"=w144, "XBPMY 2"=w143, "Hutch"=w132, "PAB"=w131, "MGV"=w130, "FCV"=w129) -> ("XBPMX 2"=w122:string, "XBPMY 2"=w121:string)  [unwired: 7 in]
    n305 = Index Array(array=w234, index #1=0 ("index"), index #2=1 ("index"), index #3=7 ("index")) -> (element #1=w229:string, element #2=w228:string, element #3=w79:string)
    n306 = call "FE_PAB_OpenState.vi"("FE"=w116, "XBPMX 2"=w112, "XBPMY 2"=w111, "Hutch"=w114, "PAB"=w128, "MGV"=w127, "FCV"=w126) -> ("XBPMX 2"=w120:string, "XBPMY 2"=w119:string)  [unwired: 7 in]
    n307 = call "FE_PAB_OpenState.vi"("FE"=w115, "XBPMX 2"=w110, "XBPMY 2"=w109, "Hutch"=w113, "PAB"=w125, "MGV"=w124, "FCV"=w123) -> ("XBPMX 2"=w118:string, "XBPMY 2"=w117:string)  [unwired: 7 in]
    n308 = Bundle("Array of X axis  平均分配至各段"=w77, w212) -> (w76:cluster{"Array of X axis  平均分配至各段":dbl[], dbl[]})  [unwired: 1 in]
    n309 = Bundle("Array of X axis  平均分配至各段"=w77, w213) -> (w75:cluster{"Array of X axis  平均分配至各段":dbl[], dbl[]})  [unwired: 1 in]
    n310 = Index Array(array=w241, index #1=2 ("index"), index #2=3 ("index"), index #3=4 ("index"), index #4=5 ("index"), index #5=6 ("index")) -> (element #1=w227:bool, element #2=w226:bool, element #3=w225:bool)  [unwired: 2 out]
    n311 = Equal?(x="1" ("1rst Value (string)"), y=w422) -> (x = y?=w420:bool)
    "x = y?" <- w420
    n312 = case shown="True" TRUE {
      tunnel: w84 -> [_ w525]
      frame False {
      }
      frame True {
        n313 = Quit LabVIEW(quit? (T)=w525) -> ()
      }
    }
    n314 = case shown="False" w420 {
      tunnel: w487 -> [_ w996]
      tunnel: w486 -> [_ w995]
      tunnel: [w994 w996] -> w217
      tunnel: [w993 w995] -> w216
      tunnel: w215 -> [w994 _]
      tunnel: w214 -> [w993 _]
      frame False {
      }
      frame True {
        n315 = local read "NOW date"() -> (→"date kickeron":string)
        n316 = local read "NOW time"() -> (→"time kickeron":string)
      }
    }
    n317 = Wait Until Next ms Multiple(millisecond multiple=u32 1000) -> ()  [unwired: 1 out]
    n318 = local read "date kickeron"() -> (w223:string)
    n319 = local read "time kickeron"() -> (w222:string)
    n320 = Get Date/Time In Seconds() -> (seconds since 1Jan1904=w335:timestamp)
    n321 = call-poly <userlib>:"CaLabGet.vi"("PV Names"=w108) -> ("1rst Value (string)"=w97:string[])  [unwired: 8 in, 6 out]
    n322 = Format Date/Time String(time format string (%c)="%Y/%m/%d", seconds (now)=w335) -> (date/time string=→"NOW date":string)  [unwired: 1 in]
    n323 = Format Date/Time String(time format string (%c)="%Y/%m/%d", seconds (now)=w335) -> (date/time string=w245:string)  [unwired: 1 in]
    n324 = Format Date/Time String(time format string (%c)="%H:%M:%S", seconds (now)=w335) -> (date/time string=w244:string)  [unwired: 1 in]
    "NOW time" <- w244
    n325 = Index Array(array=w97, index #1=0 ("index"), index #2=1 ("index"), index #3=2 ("index"), index #4=3 ("index"), index #5=4 ("index"), index #6=5 ("index"), index #7=6 ("index"), index #8=7 ("index"), index #9=8 ("index"), index #10=9 ("index")) -> (element #1=w96:string, element #2=w95:string, element #3=w94:string, element #4=w93:string, element #5=w92:string, element #6=w91:string, element #7=w90:string, element #8=w89:string, element #9=w88:string, element #10=w87:string)
    n326 = Bundle By Name(cluster=T1 {"SR Fill Pattern"=array[864 elements], "Beam Current(mA"=320.769453, "Beam Lifetime(min)"=354.3939151043138, "Beamsize X(um)"=63.15189373514937, "Beamsize Y(um)"=38.03691397287648, "Tune X(from BPM)"=0.1487279843444227, "Tune Y(from BPM)"=0.2309197651663405, "Mode"="Top-Up", "NuX(from BBF) "=0.15142063757609414, "NuY(from BBF)"=0.22496346361412184, "IU22-23gap(R)"=7.0, "IU22-05gap(R)"=7.372, "IU22-05M"=TRUE, "IU22A-09gap(R)"=8.05, "IU22A-09M"=TRUE, "IU22B-09gap(R)"=40.001, "IU22B-09M"=FALSE, "IUT22-21gap(R)"=7.0, "IUT22-21M"=TRUE, "IU22-23M"=TRUE, "IU22A-25gap(R)"=7.0, "IU22A-25M"=TRUE, "IU22B-25gap(R)"=40.0, "IU22B-25M"=FALSE, "EPU48A-41gap(R)"=65.00055, "EPU48A-41gM"=FALSE, "EPU48B-41gap(R)"=27.450000000000003, "EPU48B-41gM"=TRUE, "EPU46-45gap(R)"=44.99850000000001, "EPU46-45gM"=FALSE, "EPU48A-41phase(R)"=0.00055, "EPU48B-41phase(R)"=0.0, "EPU46-45phase(R)"=5e-05, "Grid volt.(V)(S)"=33.0, "Gun mode"="MBM", "Mod.3 HV(kV)(S)"=35.37999999999996, "SR"="SR_DMB_2017_1024_0300LOCO.data", "BR"="Booster_2017_1023_0900.data", "Linac"="Linac_2017_0413_1015.data", "LTB"="LTB_JT_2017_0828_1050.data", "BTS"="BTS_2017_1023_0900.data", "RF2 remote"=TRUE, "RF2 OP mode"=TRUE, "RF2 phase.(S)"=-42.0, "RF Freq.(s)"=499655365.67399085, "RF2 gap volt.(S)"=1600.0, "RF3 remote"=TRUE, "RF3 OP mode"=TRUE, "RF3 phase.(S)"=1.1999999999999995, "RF3 gap volt.(S)"=1600.0, "BBF V"=TRUE, "BBF H"=TRUE, "BR ext. kicker1(kV)"=17.666, "BR ext. kicker2(kV)"=17.666, "BR ext. sep.1(V)"=322.14, "BR ext. sep.2(V)"=441.1, "BR inj. sep.(V)"=104.95, "BR inj. kicker(kV)"=13.449999999999969, "SR kicker4(kV)"=7.945, "SR kicker3(kV)"=8.02, "SR kicker2(kV)"=8.142, "SR kicker1(kV)"=8.1, "SR inj. sep.2(V)"=397.2, "SR inj. sep.1(V)"=398.04, "Bucket Start"=100.0, "Bucket Last"=450.0, "Bucket Step"=10.0, "Orbit ILK(P)"=TRUE, "IU22-05 Hutch Enable"=TRUE, "IU22A-09M Hutch Enable"=TRUE, "IUT22-21M Hutch Enable"=TRUE, "IU22-23M Hutch Enable"=TRUE, "IU22A-25M Hutch Enable"=TRUE, "EPU48A-41M Hutch Enable"=TRUE, "EPU46-45M Hutch Enable"=FALSE, "EPU46-45 FE Enable"=TRUE, "EPU48A-41 FE Enable"=TRUE, "IU22A-25 FE Enable"=TRUE, "IU22-23 FE Enable"=TRUE, "IUT22-21 FE Enable"=TRUE, "IU22A-09 FE Enable"=TRUE, "IU22-05 FE Enable"=TRUE, "EPU48A-41pM"=FALSE, "EPU48B-41pM"=TRUE, "EPU46-45pM"=FALSE, "Gun volt.(V)(S)"=23.5, "Width count"=75.0, "2ns step"=2.0, "10ps delay"=150.0, "phase shifter"=130.0015, "Taper"=1.0899999999999999, "05XBPMX 1"=14.279, "09XBPMX 1"=-34.837, "21XBPMX 1"=-36.466, "23XBPMX 1"=-38.547000000000004, "25XBPMX 1"=-40.08, "41XBPMX 1"=-513.551, "45XBPMX 1"=-12.86, "05XBPMY 1"=51.999, "09XBPMY 1"=30.004, "21XBPMY 1"=-4.771, "23XBPMY 1"=19.080000000000002, "25XBPMY 1"=-4.366, "41XBPMY 1"=309.241, "45XBPMY 1"=1.842, "FOFB H"="On", "FOFB V"="On", "time string"="15:45:09", "date"="2017/10/28", "date (last kicker ON)"="2017/10/28", "time string (last kicker ON)"="15:43:52", "Radio Buttons 2"=enum."absolute", "09XBPMX 2"="23.77", "09XBPMY 2"="-18.01", "05XBPMY 2"="-459.85", "05XBPMX 2"="-403.56", "21XBPMY 2"="-134.87", "21XBPMX 2"="-31.92", "23XBPMY 2"="233.82", "23XBPMX 2"="11.09", "25XBPMY 2"="5171.53", "25XBPMX 2"="2152.43", "41XBPMY 2"=" closed", "41XBPMX 2"=" PAB ", "45XBPMX 2"=" Hutch ", "45XBPMY 2"=" closed", "05 mode"="Follow", "09A mode"="Follow", "09B mode"="Follow", "21 mode"="Follow", "23 mode"="Follow", "25A mode"="Follow", "25B mode"="Follow", "41A mode"="Follow", "41B mode"="Follow", "46 mode"="Follow", "BeamCurrent History"={"BPM NO.  1_172"=array[4319 elements], array[4319 elements]}, "SR Beam Current in            hours"=12.0, "RF FB"="On", "BPMX Graph 2"={"Array of X axis  平均分配至各段"=[1.0, 1.1666666666666667, 1.3333333333333333, 1.5, 1.6666666666666665, 1.8333333333333333, 2.0, 2.142857142857143, 2.2857142857142856, 2.4285714285714284, 2.571428571428571, 2.7142857142857144, 2.857142857142857, 3.0, 3.142857142857143, 3.2857142857142856, 3.4285714285714284, 3.571428571428571, 3.7142857142857144, 3.857142857142857, 4.0, 4.125, 4.25, 4.375, 4.5, 4.625, 4.75, 4.875, 5.0, 5.125, 5.25, 5.375, 5.5, 5.625, 5.75, 5.875, 6.0, 6.142857142857143, 6.285714285714286, 6.428571428571429, 6.571428571428571, 6.714285714285714, 6.857142857142857, 7.0, 7.142857142857143, 7.285714285714286, 7.428571428571429, 7.571428571428571, 7.714285714285714, 7.857142857142857, 8.0, 8.142857142857142, 8.285714285714286, 8.428571428571429, 8.571428571428571, 8.714285714285714, 8.857142857142858, 9.0, 9.142857142857142, 9.285714285714286, 9.428571428571429, 9.571428571428571, 9.714285714285714, 9.857142857142858, 10.0, 10.142857142857142, 10.285714285714286, 10.428571428571429, 10.571428571428571, 10.714285714285714, 10.857142857142858, 11.0, 11.142857142857142, 11.285714285714286, 11.428571428571429, 11.571428571428571, 11.714285714285714, 11.857142857142858, 12.0, 12.125, 12.25, 12.375, 12.5, 12.625, 12.75, 12.875, 13.0, 13.125, 13.25, 13.375, 13.5, 13.625, 13.75, 13.875, 14.0, 14.142857142857142, 14.285714285714286, 14.428571428571429, 14.571428571428571, 14.714285714285714, 14.857142857142858, 15.0, 15.142857142857142, 15.285714285714286, 15.428571428571429, 15.571428571428571, 15.714285714285714, 15.857142857142858, 16.0, 16.142857142857142, 16.285714285714285, 16.428571428571427, 16.571428571428573, 16.714285714285715, 16.857142857142858, 17.0, 17.142857142857142, 17.285714285714285, 17.428571428571427, 17.571428571428573, 17.714285714285715, 17.857142857142858, 18.0, 18.142857142857142, 18.285714285714285, 18.428571428571427, 18.571428571428573, 18.714285714285715, 18.857142857142858, 19.0, 19.142857142857142, 19.285714285714285, 19.428571428571427, 19.571428571428573, 19.714285714285715, 19.857142857142858, 20.0, 20.125, 20.25, 20.375, 20.5, 20.625, 20.75, 20.875, 21.0, 21.125, 21.25, 21.375, 21.5, 21.625, 21.75, 21.875, 22.0, 22.142857142857142, 22.285714285714285, 22.428571428571427, 22.571428571428573, 22.714285714285715, 22.857142857142858, 23.0, 23.142857142857142, 23.285714285714285, 23.428571428571427, 23.571428571428573, 23.714285714285715, 23.857142857142858, 24.0, 24.166666666666668, 24.333333333333332, 24.5, 24.666666666666668, 24.833333333333332], [-104.35000000000001, -27.61, -81.269, 31.074, 6.062, -136.0, 99.494, -88.141, -46.889, -165.06900000000002, 6.021, -84.98, 1.75, -8.811, 8.532, -133.949, -96.848, 24.799, 5.059, -100.301, 144.643, -9.353, 21.271, -55.053000000000004, 53.308, 191.175, 158.868, 222.566, -123.501, -26.869, 534.8770000000001, 573.141, -225.076, -6.779, 120.711, -75.419, 85.256, 50.948, -59.4, -203.09900000000002, -20.847, 130.465, -112.508, 76.115, 15.039, -35.207, -105.659, -16.897000000000002, 68.91, -141.159, 107.378, 144.351, -55.053000000000004, -193.076, 129.21, 58.157000000000004, -162.566, 153.643, 28.149, 9.358, -84.211, 85.112, 22.422, -31.252, 89.379, -47.49, 54.793, -68.275, 110.611, -118.584, -371.90500000000003, -20.115000000000002, -329.103, -249.097, -146.817, 118.556, -25.749, -98.32600000000001, 55.269, -122.093, 50.967, -55.89, 88.019, -0.462, -608.1560000000001, -139.752, -304.999, -215.022, 93.23400000000001, 44.699, -65.235, 37.049, -3.491, -169.852, 216.458, 50.398, -92.285, -132.13400000000001, -12.869, 66.74, -188.53300000000002, 148.653, -5.112, -71.334, -177.681, 41.168, -12.532, -184.913, 194.919, 52.414, -75.628, -80.415, -36.814, 105.73100000000001, -104.36800000000001, 110.101, 49.669000000000004, -67.327, -157.372, 29.624000000000002, 22.156, -105.663, 47.799, 11.591000000000001, -75.285, -79.821, 34.331, -24.937, -158.703, 177.15, 200.872, -165.849, -60.67, 20.183, -15.311, -111.206, 107.58800000000001, 26.489, 69.547, -41.230000000000004, 81.986, 54.43, 253.076, 378.43600000000004, -117.003, -304.999, 131.013, 2.21, -158.435, 94.489, 63.017, -82.94500000000001, 99.147, 65.752, -37.261, -102.577, 41.791000000000004, 66.599, -163.73, 160.137, -7.15, -51.275, -140.353, 33.772, 54.203, -147.597, 128.696, 58.22, -47.144, -184.493, 56.980000000000004, 67.437, -54.227000000000004, -0.031]}, "BPMY Graph 2"={"Array of X axis  平均分配至各段"=[1.0, 1.1666666666666667, 1.3333333333333333, 1.5, 1.6666666666666665, 1.8333333333333333, 2.0, 2.142857142857143, 2.2857142857142856, 2.4285714285714284, 2.571428571428571, 2.7142857142857144, 2.857142857142857, 3.0, 3.142857142857143, 3.2857142857142856, 3.4285714285714284, 3.571428571428571, 3.7142857142857144, 3.857142857142857, 4.0, 4.125, 4.25, 4.375, 4.5, 4.625, 4.75, 4.875, 5.0, 5.125, 5.25, 5.375, 5.5, 5.625, 5.75, 5.875, 6.0, 6.142857142857143, 6.285714285714286, 6.428571428571429, 6.571428571428571, 6.714285714285714, 6.857142857142857, 7.0, 7.142857142857143, 7.285714285714286, 7.428571428571429, 7.571428571428571, 7.714285714285714, 7.857142857142857, 8.0, 8.142857142857142, 8.285714285714286, 8.428571428571429, 8.571428571428571, 8.714285714285714, 8.857142857142858, 9.0, 9.142857142857142, 9.285714285714286, 9.428571428571429, 9.571428571428571, 9.714285714285714, 9.857142857142858, 10.0, 10.142857142857142, 10.285714285714286, 10.428571428571429, 10.571428571428571, 10.714285714285714, 10.857142857142858, 11.0, 11.142857142857142, 11.285714285714286, 11.428571428571429, 11.571428571428571, 11.714285714285714, 11.857142857142858, 12.0, 12.125, 12.25, 12.375, 12.5, 12.625, 12.75, 12.875, 13.0, 13.125, 13.25, 13.375, 13.5, 13.625, 13.75, 13.875, 14.0, 14.142857142857142, 14.285714285714286, 14.428571428571429, 14.571428571428571, 14.714285714285714, 14.857142857142858, 15.0, 15.142857142857142, 15.285714285714286, 15.428571428571429, 15.571428571428571, 15.714285714285714, 15.857142857142858, 16.0, 16.142857142857142, 16.285714285714285, 16.428571428571427, 16.571428571428573, 16.714285714285715, 16.857142857142858, 17.0, 17.142857142857142, 17.285714285714285, 17.428571428571427, 17.571428571428573, 17.714285714285715, 17.857142857142858, 18.0, 18.142857142857142, 18.285714285714285, 18.428571428571427, 18.571428571428573, 18.714285714285715, 18.857142857142858, 19.0, 19.142857142857142, 19.285714285714285, 19.428571428571427, 19.571428571428573, 19.714285714285715, 19.857142857142858, 20.0, 20.125, 20.25, 20.375, 20.5, 20.625, 20.75, 20.875, 21.0, 21.125, 21.25, 21.375, 21.5, 21.625, 21.75, 21.875, 22.0, 22.142857142857142, 22.285714285714285, 22.428571428571427, 22.571428571428573, 22.714285714285715, 22.857142857142858, 23.0, 23.142857142857142, 23.285714285714285, 23.428571428571427, 23.571428571428573, 23.714285714285715, 23.857142857142858, 24.0, 24.166666666666668, 24.333333333333332, 24.5, 24.666666666666668, 24.833333333333332], [-143.858, -13.775, -13.785, 122.665, -66.475, 31.541, 2.118, -24.67, 28.275000000000002, 0.139, -36.578, -28.396, 48.925000000000004, 9.287, -3.412, 70.053, -21.479, 14.89, -7.234, 5.521, -3.164, 19.558, -37.538000000000004, 37.11, -77.159, -13.755, 77.63, 28.249000000000002, -209.114, -44.569, 92.851, 173.641, -70.156, -22.722, 17.795, -6.59, 25.654, -41.882, 53.713, 9.237, -26.164, 18.357, 63.695, -8.542, 5.183, -5.99, 9.508000000000001, -5.462, -29.446, 36.574, -52.552, 51.439, -48.502, 0.73, -23.836000000000002, -3.648, -9.628, -5.485, -68.679, 95.486, -62.041000000000004, 54.633, -58.791000000000004, 68.305, -49.682, 29.838, -8.459, 3.213, -5.561, -80.617, 58.144, 15.346, -158.743, -40.726, 5.259, 3.258, 41.128, -54.377, 5.01, 18.84, 11.403, -20.73, 21.792, -17.296, 27.29, 0.783, -6.804, -137.476, 116.70700000000001, -6.929, 17.846, -3.586, 11.754, 6.341, 0.292, -0.911, -8.236, -5.312, 14.939, -29.945, 30.573, -9.991, -49.344, 82.117, -27.45, 22.291, -6.636, -9.389, 10.034, -14.218, 14.215, -7.3, 12.409, -44.302, 50.197, -36.089, -9.120000000000001, 45.881, 14.836, -27.324, 10.765, -10.139, -33.252, 2.737, -9.99, -6.019, -53.329, -28.159, 2.676, -36.9, -2.372, 8.92, 13.599, -25.723, -16.436, 7.722, -0.088, -29.122, 32.814, -20.521, 30.155, -45.734, 36.611000000000004, 74.528, 68.482, -22.548000000000002, -31.398, 134.603, -45.587, -0.981, -40.156, 24.441, 20.477, -31.424, 19.5, -11.789, 16.394000000000002, -38.567, 9.523, 0.09, -0.058, -4.8500000000000005, 11.71, 25.637, -10.51, -18.101, -12.389000000000001, 95.417, -138.726, 30.355, 96.245, -48.666000000000004, 40.851, -0.71]}, "gap value："=300} ("Cluster"), "Tune X(from BPM)"=w217, "Tune Y(from BPM)"=w216, "date (last kicker ON)"=w223, "time string (last kicker ON)"=w222, "date"=w245, "time string"=w244, "Mode"=w327, "Beam Current(mA"=w326, "Beam Lifetime(min)"=w325, "Beamsize X(um)"=w324, "Beamsize Y(um)"=w323, "NuX(from BBF)"=w322, "NuY(from BBF)"=w321, "Bucket Start"=w320, "Bucket Last"=w319, "Bucket Step"=w318, "BR inj. sep.(V)"=w317, "BR inj. kicker(kV)"=w316, "BR ext. kicker1(kV)"=w315, "BR ext. kicker2(kV)"=w314, "BR ext. sep.1(V)"=w313, "BR ext. sep.2(V)"=w312, "SR inj. sep.1(V)"=w311, "SR inj. sep.2(V)"=w310, "SR kicker1(kV)"=w309, "SR kicker2(kV)"=w308, "SR kicker3(kV)"=w307, "SR kicker4(kV)"=w306, "Gun mode"=w305, "Grid volt.(V)(S)"=w304, "Gun volt.(V)(S)"=w303, "Mod.3 HV(kV)(S)"=w302, "Width count"=w301, "2ns step"=w300, "10ps delay"=w299, "RF2 remote"=w298, "RF2 OP mode"=w297, "RF2 phase.(S)"=w221, "RF Freq.(s)"=w296, "RF2 gap volt.(S)"=w220, "RF3 remote"=w295, "RF3 OP mode"=w294, "RF3 phase.(S)"=w293, "RF3 gap volt.(S)"=w292, "BR"=w291, "BTS"=w290, "Linac"=w288, "LTB"=w287, "SR"=w289, "SR Fill Pattern"=w70, "IU22-05 Hutch Enable"=w170, "IU22A-09M Hutch Enable"=w166, "IUT22-21M Hutch Enable"=w150, "IU22-23M Hutch Enable"=w133, "IU22A-25M Hutch Enable"=w132, "EPU48A-41M Hutch Enable"=w114, "EPU46-45M Hutch Enable"=w113, "EPU46-45 FE Enable"=w115, "EPU48A-41 FE Enable"=w116, "IU22A-25 FE Enable"=w134, "IU22-23 FE Enable"=w135, "IUT22-21 FE Enable"=w153, "IU22A-09 FE Enable"=w165, "IU22-05 FE Enable"=w171, "IU22-05gap(R)"=w286, "IU22A-09gap(R)"=w285, "IU22B-09gap(R)"=w284, "IUT22-21gap(R)"=w283, "IU22-23gap(R)"=w282, "IU22A-25gap(R)"=w281, "IU22B-25gap(R)"=w280, "EPU48A-41gap(R)"=w279, "EPU48A-41phase(R)"=w278, "EPU48B-41gap(R)"=w277, "EPU48B-41phase(R)"=w276, "EPU46-45gap(R)"=w275, "EPU46-45phase(R)"=w274, "Taper"=w218, "phase shifter"=w273, "05XBPMX 1"=w272, "09XBPMX 1"=w271, "21XBPMX 1"=w270, "23XBPMX 1"=w269, "25XBPMX 1"=w268, "41XBPMX 1"=w267, "45XBPMX 1"=w266, "05XBPMY 1"=w265, "09XBPMY 1"=w264, "21XBPMY 1"=w263, "23XBPMY 1"=w262, "25XBPMY 1"=w261, "41XBPMY 1"=w260, "45XBPMY 1"=w259, "IU22-05M"=w258, "IU22A-09M"=w257, "IU22B-09M"=w256, "IUT22-21M"=w255, "IU22-23M"=w254, "IU22A-25M"=w253, "IU22B-25M"=w252, "EPU48A-41gM"=w251, "EPU48B-41gM"=w250, "EPU46-45gM"=w249, "EPU48A-41pM"=w248, "EPU48B-41pM"=w247, "EPU46-45pM"=w246, "BPMX Graph 2"=w76, "BPMY Graph 2"=w75, "Radio Buttons 2"=enum32{"absolute", "different with"}."absolute", "FOFB H"=w229, "FOFB V"=w228, "BBF H"=w227, "BBF V"=w226, "Orbit ILK(P)"=w225, "05XBPMX 2"=w160, "05XBPMY 2"=w159, "09XBPMX 2"=w158, "09XBPMY 2"=w157, "21XBPMX 2"=w142, "21XBPMY 2"=w141, "23XBPMX 2"=w140, "23XBPMY 2"=w139, "25XBPMX 2"=w122, "25XBPMY 2"=w121, "41XBPMX 2"=w120, "41XBPMY 2"=w119, "45XBPMX 2"=w118, "45XBPMY 2"=w117, "05 mode"=w96, "09A mode"=w95, "09B mode"=w94, "21 mode"=w93, "23 mode"=w92, "25A mode"=w91, "25B mode"=w90, "41A mode"=w89, "41B mode"=w88, "46 mode"=w87, "BeamCurrent History"=w83, "RF FB"=w79, "gap value："=w69) -> (→"Cluster":T1)
  }
  n327 = while {
    tunnel: w8 -> [_]
    shift-right: [w1035] -> _
    shift-left: string[] [] -> [w1032]
    shift-right: [w1014] -> _
    shift-left: string[][] [] -> [w1021]
    tunnel: w18 -> [w1024]
    i -> [w1022]
    stop <- w1023 stop-if-true
    w1018 = 5000  # limit
    # "為了使檯面上記憶體不要使用太多而做的筆數限制"
    n328 = flat-sequence {
      tunnel: [w1048] -> w1036
      tunnel: [w1047] -> w1033
      tunnel: w1032 -> [w1047]
      tunnel: [w1046] -> w1025
      tunnel: w1024 -> [w1046]
      tunnel: [w1058] -> w1037
      tunnel: w1036 -> [w1058]
      tunnel: [w1056] -> w1034
      tunnel: w1033 -> [w1057]
      tunnel: [w1050] -> w1031
      tunnel: w1025 -> [w1049]
      tunnel: w1037 -> [w1081]
      tunnel: [w1079] -> w1035
      tunnel: w1034 -> [w1079]
      tunnel: w1031 -> [w1078]
      tunnel: [w1078] -> w1027
      frame #0 {
        n329 = Tick Count (ms)() -> (millisecond timer value=w1048:u32)
      }
      frame #1 {
        n330 = Get Date/Time In Seconds() -> (seconds since 1Jan1904=w1053:timestamp)
        n331 = To Double Precision Float(number=w1053) -> (double precision float=w1052:dbl)
        n332 = Format Date/Time String(time format string (%c)="%Y/%m/%d %H:%M:%S", seconds (now)=w1053) -> (date/time string=w1054:string)  [unwired: 1 in]
        n333 = Number To Fractional String(number=w1052) -> (F-format string=w1051:string)  [unwired: 3 in]
        n334 = call-poly <userlib>:"CaLabGet.vi"("PV Names"=w1049) -> ("1rst Value (string)"=w1056:string[])  [unwired: 8 in, 6 out]
        n335 = for {
          tunnel: w1057 -> [w1060] mode=indexing
          tunnel: w1056 -> [w1059] mode=indexing
          tunnel: w1049 -> [w1068] mode=indexing
          tunnel: w1054 -> [w1067]
          tunnel: [w1066] -> w1050 mode=indexing if=w1064
          tunnel: w1051 -> [w1065]
          i -> [w1063]
          n336 = Greater Or Equal?(x=w1063, y=1) -> (x >= y?=w1061:bool)
          n337 = case shown="True" w1061 {
            tunnel: w1068 -> [_ w1077]
            tunnel: w1060 -> [_ w1076]
            tunnel: w1059 -> [_ w1075]
            tunnel: w1067 -> [_ w1074]
            tunnel: [string[] [] w1073] -> w1066
            tunnel: w1065 -> [_ w1072]
            tunnel: [FALSE w1071] -> w1064
            frame False {
            }
            frame True {
              n338 = Not Equal?(x=w1076, y=w1075) -> (x != y?=w1071:bool)
              n339 = Build Array(w1074, w1077, w1076, w1075, w1072) -> (w1073:string[])
            }
          }
        }
      }
      frame #2 {
        n340 = Tick Count (ms)() -> (millisecond timer value=w1082:u32)
        n341 = Subtract(x=w1082, y=w1081) -> (x-y=→"dT":u32)
      }
    }
    n342 = while {
      i -> [w1039]
      stop <- w1043 stop-if-true
      # "每60秒，表示法:\n100 600"
      # "每十秒，表示法:\n100 100"
      n343 = local read "stop"() -> (w1042:bool)
      n344 = Multiply(x="Check period", y=10) -> (x*y=w1040:i32)
      n345 = Greater Or Equal?(x=w1039, y=w1040) -> (x >= y?=w1044:bool)
      n346 = Wait Until Next ms Multiple(millisecond multiple=u32 99) -> ()  [unwired: 1 out]
      n347 = Or(x=w1044, y=w1042) -> (x .or. y?=w1043:bool)
    }
    n348 = Index Array(array=w1021, index (row)=0) -> (element=w1029:string[])  [unwired: 1 in]
    n349 = Array Size(array=w1029) -> (size(s)=w1012:i32)
    "EVENTs" <- w1012
    n350 = Greater?(x=w1012, y=0) -> (0:→"x > y?":bool)
    n351 = Build Array (concatenate)(w1021, w1027) -> (w1013:string[][])
    n352 = local read "stop"() -> (w1023:bool)
    n353 = Subtract(x=w1012, y=w1018) -> (x-y=w1017:i32)
    n354 = Add(x=w1018, y=3) -> (x+y=w1020:i32)
    n355 = Array Subset(array=w1013, index (row)=w1017, length (row)=w1020, index (col)=0 ("index"), length (col)=5 ("length")) -> (w1014:string[][])
    "Diff list" <- w1014
    "check loop" <- w1022
  }
  n356 = local write "stop"(FALSE ("stop")) -> ()
